vi "TC-4.59-backup.vi"() -> ()   [LabVIEW 2013]
uses:
  1. Sources/Lib/Lib.llb/CS mode.ctl
  1. Sources/Lib/Lib.llb/R.ctl
  1. Sources/Lib/Lib.llb/T.ctl
  1. Sources/Lib/Lib.llb/Calibrations.ctl
  1. Sources/Lib/Lib.llb/CS.lvclass
  1. Sources/Lib/Lib.llb/PID Settings.ctl
  1. Sources/Lib/Lib.llb/AVS_exc_n_ranges.ctl
  1. Sources/Lib/Lib.llb/AVS_excitation.ctl
  1. Sources/Lib/Lib.llb/AVS47_range.ctl
  1. Sources/Lib/Lib.llb/Ch descriptions.ctl
  1. Sources/Lib/Lib.llb/Cursor Controls.ctl
  1. Sources/Lib/Lib.llb/DataArray.ctl
  1. Sources/Lib/Lib.llb/Unit.ctl
  1. Sources/Lib/Lib.llb/Control 6.ctl
  1. Sources/Lib/Lib.llb/Control 4.ctl
  1. Sources/Lib/Lib.llb/Control 8.ctl
  1. Sources/Lib/Lib.llb/VI FPO Ref.ctl
  1. Sources/Lib/support/Class ID ENUM.ctl
  1. Sources/Lib/Lib.llb/Type Descriptor Enumeration__ogtk.ctl
  1. Sources/Lib/Lib.llb/Refnum Subtype Enum__ogtk.ctl
  1. Sources/Lib/Lib.llb/Waveform Subtype Enum__ogtk.ctl
  1. Sources/Lib/Lib.llb/LV Data cluster.ctl
  1. Sources/Lib/Lib.llb/Action.ctl
  Leiden to DSC/TC to DSC/Typedefs/TC-cluster.ctl
  1. Sources/Lib/Lib.llb/TCS.lvclass
  1. Sources/Lib/Lib.llb/QCS.lvclass
  1. Sources/Lib/Lib.llb/CS Emulation.lvclass
  1. Sources/Lib/Lib.llb/PCS.lvclass
  1. Sources/Lib/Lib.llb/Byte Params.ctl
  1. Sources/Lib/Lib.llb/MView.lvlib
panel:
  out "R Array":dbl[](array[numeric])
  out "_SetControl":T1
  out "ControlNames":string[](array[string])
  out "VIRef":T2 {"Array DataType" format="%.0x"; "WaveForm Type" format="%.0x"; "RefNum Type" format="%.0x"; "DataType" format="%.0x"}
  out "VI called?":bool=TRUE
  out "Error code":u8
  out "_zBridgeSetNr":u8 caption="zBridge set nr."
  out "_zBridgeDll":path=path "C:/Users/Sasha/Dropbox/Labview/LC Software/ImpSoft-V5.2.2-multithreaded/ImpBridgeLabview/ImpBridgeDll.dll"
  in  "_String":string="^ Click the Run button to start the program "
  in  "Top Toolbar":enum32{"Page 1", "Page 2"}(tab)
  in  "Load config":bool
  in  "Start":bool
  in  "Load Data":bool
  in  "Pause":bool
  in  "Stop":bool
  in  "Copy to Clipboard":bool
  in  "Save config":bool
  in  "Clear all plots":bool
  in  "ColorBox":enum32{"Page 1", "Page 2"}(tab)
  in  "Colors":picture
  out "Color":u32(colorbox)
  in  "Graph-open popup":bool
  out "_CalibFilesPath":path=path "C:/avs-47/aaaa"
  out "_LogFilesPath":path
  out "_AVS_VISA":refnum<visa-resource-name>="COM3"
  in  "Minimize UI 2":bool
  out "VI Version":string="TC" caption="V"
  in  "Minimize UI 1":bool
  in  "Main Panel":enum32{"AVS"}(tab)
  in  "Graph Controls Bar":enum32{"Page 1"}(tab)
  in  "Mode Buttons":T7
  in  "Erase all":bool
  in  "Plot-Save All":bool
  in  "Plot-save-screen":bool
  in  "Channels Panel":T8(tab)=enum."All"
  out "T0":dbl=nan caption="T" format="%#.2p"
  out "R0":dbl caption="R" format="%.3p"
  out "R-Plot 0":cluster{dbl[], dbl[]}(graph) caption="R-Plot"
  out "T1":dbl=nan caption="T" format="%#.2p"
  out "R1":dbl caption="R" format="%.3p"
  out "R-Plot 1":cluster{dbl[], dbl[]}(graph) caption="R-Plot"
  out "T2":dbl=nan caption="T" format="%#.2p"
  out "R2":dbl caption="R" format="%.3p"
  out "R-Plot 2":cluster{dbl[], dbl[]}(graph) caption="R-Plot"
  out "T3":dbl=nan caption="T" format="%#.2p"
  out "R3":dbl caption="R" format="%.3p"
  out "R-Plot 3":cluster{dbl[], dbl[]}(graph) caption="R-Plot"
  out "T4":dbl=nan caption="T" format="%#.2p"
  out "R4":dbl caption="R" format="%.3p"
  out "R-Plot 4":cluster{dbl[], dbl[]}(graph) caption="R-Plot"
  out "T5":dbl=nan caption="T" format="%#.2p"
  out "R5":dbl caption="R" format="%.3p"
  out "R-Plot 5":cluster{dbl[], dbl[]}(graph) caption="R-Plot"
  out "T6":dbl=nan caption="T" format="%#.2p"
  out "R6":dbl caption="R" format="%.3p"
  out "R-Plot 6":cluster{dbl[], dbl[]}(graph) caption="R-Plot"
  out "T7":dbl=nan caption="T" format="%#.2p"
  out "R7":dbl caption="R" format="%.3p"
  out "R-Plot 7":cluster{dbl[], dbl[]}(graph) caption="R-Plot"
  out "T8":dbl=nan caption="T" format="%#.2p"
  out "R8":dbl caption="R" format="%.3p"
  out "R-Plot 8":cluster{dbl[], dbl[]}(graph) caption="R-Plot"
  out "T9":dbl=nan caption="T" format="%#.2p"
  out "R9":dbl caption="R" format="%.3p"
  out "R-Plot 9":cluster{dbl[], dbl[]}(graph) caption="R-Plot"
  out "T Cluster":T9 {"T9" format="%.2p"; "T8" format="%.2p"; "T7" format="%.2p"; "T6" format="%.2p"; "T5" format="%.2p"; "T4" format="%.2p"; "T3" format="%.2p"; "T2" format="%.2p"; "T1" format="%.2p"; "T0" format="%.2p"}
  in  "Sensor Names":T10={"AVS Name 0"="C_still", "AVS Name 1"="3K", "AVS Name 2"="Still", "AVS Name 3"="50mK", "AVS Name 4"="MC", "AVS Name 5"="MC", "AVS Name 6"="MC", "AVS Name 7"="", "AVS Name 8"="", "AVS Name 9"=""}
  in  "Edit Calibrations":T11
  in  "Sensor Calibrations":T12 {"Sensor 10" items=["No Calibration", "PT100", "PT1000", "RuO2 10k", "RuO2 1k5", "RuO2 2k", "Emulation R", "PT 1000", "RuO2-10K-NEW", "testCMN", "No Calibration"]; "Sensor 9" items=["No Calibration", "PT100", "PT1000", "RuO2 10k", "RuO2 1k5", "RuO2 2k", "Emulation R", "PT 1000", "RuO2-10K-NEW", "testCMN", "No Calibration"]; "Sensor 8" items=["No Calibration", "PT100", "PT1000", "RuO2 10k", "RuO2 1k5", "RuO2 2k", "Emulation R", "PT 1000", "RuO2-10K-NEW", "testCMN", "No Calibration"]; "Sensor 7" items=["No Calibration", "PT100", "PT1000", "RuO2 10k", "RuO2 1k5", "RuO2 2k", "Emulation R", "PT 1000", "RuO2-10K-NEW", "testCMN", "No Calibration"]; "Sensor 6" items=["No Calibration", "PT100", "PT1000", "RuO2 10k", "RuO2 1k5", "RuO2 2k", "Emulation R", "PT 1000", "RuO2-10K-NEW", "testCMN", "No Calibration"]; "Sensor 5" items=["No Calibration", "PT100", "PT1000", "RuO2 10k", "RuO2 1k5", "RuO2 2k", "Emulation R", "PT 1000", "RuO2-10K-NEW", "testCMN", "No Calibration"]; "Sensor 4" items=["No Calibration", "PT100", "PT1000", "RuO2 10k", "RuO2 1k5", "RuO2 2k", "Emulation R", "PT 1000", "RuO2-10K-NEW", "testCMN", "No Calibration"]; "Sensor 3" items=["No Calibration", "PT100", "PT1000", "RuO2 10k", "RuO2 1k5", "RuO2 2k", "Emulation R", "PT 1000", "RuO2-10K-NEW", "testCMN", "No Calibration"]; "Sensor 2" items=["No Calibration", "PT100", "PT1000", "RuO2 10k", "RuO2 1k5", "RuO2 2k", "Emulation R", "PT 1000", "RuO2-10K-NEW", "testCMN", "No Calibration"]; "Sensor 1" items=["No Calibration", "PT100", "PT1000", "RuO2 10k", "RuO2 1k5", "RuO2 2k", "Emulation R", "PT 1000", "RuO2-10K-NEW", "testCMN", "No Calibration"]}
  out "Units":T13
  out "R Cluster":T14={"R0"=0.0, "R1"=0.0, "R2"=-0.0, "R3"=0.0, "R4"=0.0, "R5"=0.0, "R6"=0.0, "R7"=0.0, "R8"=0.0, "R9"=0.0} {"R9" format="%.3p"; "R8" format="%.3p"; "R7" format="%.3p"; "R6" format="%.3p"; "R5" format="%.3p"; "R4" format="%.3p"; "R3" format="%.3p"; "R2" format="%.3p"; "R1" format="%.3p"; "R0" format="%.3p"}
  in  "AVS Scan Parameters":enum32{"Page 1", "Page 2"}(tab)
  in  "AVS Exc&Ranges":T15={"Excitation 0"=4, "Excitation 1"=4, "Excitation 2"=3, "Excitation 3"=3, "Excitation 4"=3, "Excitation 5"=3, "Excitation 6"=3, "Excitation 7"=3, "Range 0"=5, "Range 1"=5, "Range 2"=5, "Range 3"=5, "Range 4"=5, "Range 5"=5, "Range 6"=5, "Range 7"=5} {"Range 7" items=["n.a."=-1, "open"=0, "2 Ohm"=1, "20 Ohm"=2, "200 Ohm"=3, "2k Ohm"=4, "20k Ohm"=5, "200k Ohm"=6, "2M Ohm"=7]; "Range 6" items=["n.a."=-1, "open"=0, "2 Ohm"=1, "20 Ohm"=2, "200 Ohm"=3, "2k Ohm"=4, "20k Ohm"=5, "200k Ohm"=6, "2M Ohm"=7]; "Range 5" items=["n.a."=-1, "open"=0, "2 Ohm"=1, "20 Ohm"=2, "200 Ohm"=3, "2k Ohm"=4, "20k Ohm"=5, "200k Ohm"=6, "2M Ohm"=7]; "Range 4" items=["n.a."=-1, "open"=0, "2 Ohm"=1, "20 Ohm"=2, "200 Ohm"=3, "2k Ohm"=4, "20k Ohm"=5, "200k Ohm"=6, "2M Ohm"=7]; "Range 3" items=["n.a."=-1, "open"=0, "2 Ohm"=1, "20 Ohm"=2, "200 Ohm"=3, "2k Ohm"=4, "20k Ohm"=5, "200k Ohm"=6, "2M Ohm"=7]; "Range 2" items=["n.a."=-1, "open"=0, "2 Ohm"=1, "20 Ohm"=2, "200 Ohm"=3, "2k Ohm"=4, "20k Ohm"=5, "200k Ohm"=6, "2M Ohm"=7]; "Range 1" items=["n.a."=-1, "open"=0, "2 Ohm"=1, "20 Ohm"=2, "200 Ohm"=3, "2k Ohm"=4, "20k Ohm"=5, "200k Ohm"=6, "2M Ohm"=7]; "Range 0" items=["n.a."=-1, "open"=0, "2 Ohm"=1, "20 Ohm"=2, "200 Ohm"=3, "2k Ohm"=4, "20k Ohm"=5, "200k Ohm"=6, "2M Ohm"=7]; "Excitation 7" items=["none", "3 µV", "10 µV", "30 µV", "100 µV", "300 µV", "1 mV", "3 mV"]; "Excitation 6" items=["none", "3 µV", "10 µV", "30 µV", "100 µV", "300 µV", "1 mV", "3 mV"]; "Excitation 5" items=["none", "3 µV", "10 µV", "30 µV", "100 µV", "300 µV", "1 mV", "3 mV"]; "Excitation 4" items=["none", "3 µV", "10 µV", "30 µV", "100 µV", "300 µV", "1 mV", "3 mV"]; "Excitation 3" items=["none", "3 µV", "10 µV", "30 µV", "100 µV", "300 µV", "1 mV", "3 mV"]; "Excitation 2" items=["none", "3 µV", "10 µV", "30 µV", "100 µV", "300 µV", "1 mV", "3 mV"]; "Excitation 1" items=["none", "3 µV", "10 µV", "30 µV", "100 µV", "300 µV", "1 mV", "3 mV"]; "Excitation 0" items=["none", "3 µV", "10 µV", "30 µV", "100 µV", "300 µV", "1 mV", "3 mV"]}
  out "zBridge.Scan Phase":T18
  out "zBridge params":T19
  out "uPlots":T20
  out "zBridge.Active Channels":T21={"active Channel 0"=TRUE, "active Channel 1"=TRUE, "active Channel 2"=TRUE, "active Channel 3"=FALSE, "active Channel 4"=FALSE, "active Channel 5"=FALSE, "active Channel 6"=FALSE, "active Channel 7"=FALSE, "active Channel 8"=FALSE, "active Channel 9"=FALSE}
  out "Waveform Chart":T22(graph)
  in  "_CS_Address":u32
  in  "Edit calibration":bool
  in  "Convert R-T":bool
  out "T7":dbl caption="T=" format="%#.2p"
  in  "QuickR":dbl caption="R=" format="%_6g"
  in  "_QuickConvertCal":u16(ring) items=["No Calibration", "PT100", "PT1000", "RuO2 10k", "RuO2 1k5", "RuO2 2k", "Emulation R", "PT 1000", "RuO2-10K-NEW", "testCMN", "No Calibration"]
  out "_CSMode1List[i]":T23[](array[typedef]) caption="I_list[i]" min=-1.0
  out "CS.Automode Current":T23[](array[typedef]) min=-1.0
  in  "Lower Panel":enum32{"Page 1", "Page 2"}(tab)
  in  "Data History/RT Settings":enum32{"History", "Settings"}(tab)=enum."Settings"
  out "AVS names small":T10={"AVS Name 0"="3K", "AVS Name 1"="Still", "AVS Name 2"="50 mK", "AVS Name 3"="MC", "AVS Name 4"="MC", "AVS Name 5"="", "AVS Name 6"="", "AVS Name 7"="", "AVS Name 8"="", "AVS Name 9"=""}
  out "zBridge.Active channel":T24
  out "Small T Cluster":T25 caption="T" {"T0" format="%#.2p"; "T1" format="%#.2p"; "T2" format="%#.2p"; "T3" format="%#.2p"; "T4" format="%#.2p"; "T5" format="%#.2p"; "T6" format="%#.2p"; "T7" format="%#.2p"; "T8" format="%#.2p"; "T9" format="%#.2p"}
  out "Small R Cluster":T26 caption="R" {"R0" format="%#_5p"; "R1" format="%#_5p"; "R2" format="%#_5p"; "R3" format="%#_5p"; "R4" format="%#_5p"; "R5" format="%#_5p"; "R6" format="%#_5p"; "R7" format="%#_5p"; "R8" format="%#_5p"; "R9" format="%#_5p"}
  out "Time":dbl format="%<%X\n%x>T"
  in  "Runtime Settings":T27={"Read AVS channels from"=0, "Last Channel"=7, "Delay Between Scans"=0, "Stabilisation Delay"=5.0, "Averages"=2, "Data Memory"=25000, "Filter Graphs"=FALSE, "Y_min"=0.0, "Y_max"=2000000.0, "Plot type"=enum."T vs Time", "Allow neg R"=TRUE, "Miniplot Time"=30.0} {"Miniplot Time" min=0.0; "Delay Between Scans" format="%.0f s"; "Averages" min=1 max=1000; "Stabilisation Delay" min=0.5; "Last Channel" min=0 max=7 step=1; "Read AVS channels from" min=0 max=7 step=1; "Y_max" format="%#_6f"; "Y_min" min=0.0 format="%#_6f"; "Data Memory" min=3 max=50000}
  out "CS.Current Value":dbl[](array[numeric])
  in  "Data Array":T28=[{"R"=[], "T"=[], "Time"=[]}, {"R"=[0.0, 2.0], "T"=[], "Time"=[]}]
  out "T Array":dbl[](array[numeric])
  in  "_ScanData":dbl[](array[numeric])
  out "_I3SetPnt":dbl
  out "_CurrentsChanged":bool
  in  "_AVSRanges":T29={"Excitationl 0"=5, "Excitation 1"=5, "Excitation 2"=5, "Excitation 3"=5, "Excitation 4"=5, "Excitation 5"=5, "Excitation 6"=5, "Excitation 7"=5} caption="Ranges" {"Excitation 7" items=["n.a."=-1, "open"=0, "2 Ohm"=1, "20 Ohm"=2, "200 Ohm"=3, "2k Ohm"=4, "20k Ohm"=5, "200k Ohm"=6, "2M Ohm"=7]; "Excitation 6" items=["n.a."=-1, "open"=0, "2 Ohm"=1, "20 Ohm"=2, "200 Ohm"=3, "2k Ohm"=4, "20k Ohm"=5, "200k Ohm"=6, "2M Ohm"=7]; "Excitation 5" items=["n.a."=-1, "open"=0, "2 Ohm"=1, "20 Ohm"=2, "200 Ohm"=3, "2k Ohm"=4, "20k Ohm"=5, "200k Ohm"=6, "2M Ohm"=7]; "Excitation 4" items=["n.a."=-1, "open"=0, "2 Ohm"=1, "20 Ohm"=2, "200 Ohm"=3, "2k Ohm"=4, "20k Ohm"=5, "200k Ohm"=6, "2M Ohm"=7]; "Excitation 3" items=["n.a."=-1, "open"=0, "2 Ohm"=1, "20 Ohm"=2, "200 Ohm"=3, "2k Ohm"=4, "20k Ohm"=5, "200k Ohm"=6, "2M Ohm"=7]; "Excitation 2" items=["n.a."=-1, "open"=0, "2 Ohm"=1, "20 Ohm"=2, "200 Ohm"=3, "2k Ohm"=4, "20k Ohm"=5, "200k Ohm"=6, "2M Ohm"=7]; "Excitation 1" items=["n.a."=-1, "open"=0, "2 Ohm"=1, "20 Ohm"=2, "200 Ohm"=3, "2k Ohm"=4, "20k Ohm"=5, "200k Ohm"=6, "2M Ohm"=7]; "Excitationl 0" items=["n.a."=-1, "open"=0, "2 Ohm"=1, "20 Ohm"=2, "200 Ohm"=3, "2k Ohm"=4, "20k Ohm"=5, "200k Ohm"=6, "2M Ohm"=7]}
  out "_CSClassRef":refnum<class "CS.lvclass">
  in  "CS Indicators Panel":enum32{"Page 1", "Page 2"}(tab)
  out "CS.Automode 0":bool
  out "CS.Automode 1":bool
  out "QCS. I0 Mapping":T30(ring) caption="Output to"
  in  "uA 0":u32
  in  "CS Cannel Names":T31={"CS Name 0"="N.C.", "CS Name 1"="3K", "CS Name 2"="Still", "CS Name 3"="MC"}
  out "I0":T32={"uA"="000", "ON"=FALSE, "Gated"=FALSE, "current flows"=FALSE, "Error"=FALSE} caption="Ch0 -"
  in  "uA 3":u32
  in  "uA 2":u32
  in  "uA 1":u32
  out "CS.Automode 3":bool
  out "CS.Automode 2":bool
  out "I3":T32={"uA"="000", "ON"=FALSE, "Gated"=FALSE, "current flows"=FALSE, "Error"=FALSE} caption="Chn 3"
  out "I2":T32={"uA"="000", "ON"=FALSE, "Gated"=FALSE, "current flows"=FALSE, "Error"=FALSE} caption="Chn 2"
  out "I1":T32={"uA"="000", "ON"=FALSE, "Gated"=FALSE, "current flows"=FALSE, "Error"=FALSE} caption="Chn 1"
  out "_ExtVIReference":refnum<vi>
  out "Small I":cluster{"I1":dbl, "I2":dbl, "I3":dbl, "I4":dbl} caption="I" {"I1" format="%#.2f"; "I2" format="%#.2p"; "I3" format="%#.2p"; "I4" format="%#.2p"}
  out "CS.Actual Current":dbl[](array[numeric])
  in  "Save Data 2":bool
  in  "Show PID graph?":bool
  in  "Set Color":bool
  out "_ZBridgeUnit":string caption="Unit"
  out "_zBridgeParText":string caption="zBridge params/Error"
  out "_CurCalibrations":T33
  out "_LMBDown":bool
  in  "Side Panel":T34(tab)
  in  "Reload Calibrations":bool
  in  "zBridge settings":bool
  out "CS.ID":string
  out "CS status":errorcluster
  out "General Error":errorcluster caption="General status"
  in  "Bridge settings":T35={"Bridge Type"=enum."AVS47A (GPIB interface)", "AVS RS232 Port"="COM5", "AVS GPIB Address"="GPIB0::20::INSTR", "Calibrations Folder"=path "C:/LC Data/Calibrations"}
  in  "CS Settings":T36={"TCS RS232 Port"="COM1", "TCS_Imax"=5, "CS type"=enum."TCS", "CS.QCS Device Nr"=0}
  in  "Data Logging Settings":T37={"Log Files Folder"=path "C:/LC Data/Data", "Log Files Name"="LogAVS", "Automode Files Name"="calibration", "Filenames Suffix"="_%Y-%m-%d-%H-%M-%S", "Delimeter"="\t", "New File Interval"=7, "New File Interval Units"=enum."Days", "Date Format"="%Y-%m-%d %H:%M:%S", "External VI Path"=path "", "Query Description"=FALSE, "Run Description"="\n"}
  out "Bridge status":errorcluster
  in  "CS.QCS I0 Output":T38(ring) caption="Set Channel 0 output to"
  in  "CS.Mode":T39 caption="CS mode"
  out "_TimeOld":dbl format="%#_16g"
  in  "CS Modes Panel":T40(tab)=enum."Automatic 1"
  in  "CS.I3":T41={"Toggle ON/OFF"=FALSE, "Toggle Gated"=FALSE, "I"=0, "Range"=enum."x1 uA"} caption="Chn 3" {"I" max=100000 step=1}
  in  "CS.I2":T41={"Toggle ON/OFF"=FALSE, "Toggle Gated"=FALSE, "I"=0, "Range"=enum."x1 uA"} caption="Chn 2" {"I" max=100000 step=1}
  in  "CS.I1":T41={"Toggle ON/OFF"=FALSE, "Toggle Gated"=FALSE, "I"=0, "Range"=enum."x1 uA"} caption="Chn 1" {"I" max=100000 step=1}
  in  "CS.I0":T41={"Toggle ON/OFF"=FALSE, "Toggle Gated"=FALSE, "I"=0, "Range"=enum."x1 uA"} caption="Chn 0" {"I" max=100000 step=1}
  in  "CS.Mode1.PID Settings":T42={"FB on 2"=enum."3", "Proportional Gain"=3.0, "Integral Gain"=3.0, "Derivative Gain"=1.0, "Deadband"=0.1, "Feed Fwd Gain [uA/mK]"=0.0, "Integral Gain Bandwidth"=10.0, "Integral Gain Background"=1.0, "Current limit, [uA]"=1.0} {"Integral Gain Background" format="%#.6g"; "Integral Gain Bandwidth" format="%#.6g"; "Feed Fwd Gain [uA/mK]" format="%#.5g"; "Deadband" format="%#.5g"; "Derivative Gain" format="%#.6g"; "Integral Gain" format="%#.6g"; "Proportional Gain" format="%#.6g"; "Current limit, [uA]" format="%#.5g"}
  in  "CS.Mode1.Start":bool
  in  "CS.Mode1.List":T23[][](array[typedef]) min=-1.0
  out "CS.Mode1.PID Column":T43[](array[typedef])
  out "CS.Mode1.Row":T44[](array[typedef])=[TRUE, FALSE, FALSE, FALSE, FALSE, FALSE, FALSE, FALSE, FALSE, FALSE]
  out "CS.Mode1.PID Stabilized?":bool caption="SP reached?"
  out "CS.Mode1.PID Error":dbl=10.0 caption="Error" format="%#_6f"
  out "CS.Mode1.Slope":dbl caption="Slope" format="%#_3g %"
  out "CS.Mode1.Timer":dbl caption="Timer" format="%<%H:%M:%S>t"
  out "CS.Mode1.List:Count":i32=10 caption="/"
  out "CS.Mode1.List:Index":i32=10 caption="Point #"
  in  "CS.Mode1.Next":bool
  in  "CS.Mode1.Reset PID":bool
  in  "CS.Mode1.Auto Advance":bool=TRUE caption="Enable automatic sweeping/list iteration"
  in  "CS.Mode1.Settings":T45={"Bridge Channel"=0, "N averages"=10, "Delay Time"=10.0, "T stability"=0.3, "FB on"=enum."Temperature"} {"Delay Time" min=0.0 format="%#_g min"; "Bridge Channel" min=-1 max=9 step=1}
  in  "CS.Mode1.Call VI?":bool caption="Call Ext. VI"
  out "CS.Mode1.VI State":T46(ring) caption="- state"
  in  "CS.Mode1.Trigger all TC":bool caption="Trigger other running TC instances"
  in  "CS.Mode1.List:Prev":bool
  in  "CS.Mode1.List:Next":bool
  in  "CS.Mode1.List:To First":bool
  in  "CS.Mode1.List:Save":bool
  in  "CS.Mode1.List:Load":bool
  in  "CS.Mode1.Write To Log":bool
  in  "CS.Mode1.PID":cluster{"Enabled":bool}
  in  "CS.Mode1.List:Clear":bool
  in  "CS.Mode2.Settings":T47={"FB on"=enum."Temperature", "Bridge Channel"=0, "Hysteresis"=10} {"Hysteresis" max=100 format="%.0f %%"; "Bridge Channel" min=-1 max=9 step=1}
  in  "CS.Mode2.Start":bool
  in  "CS.Mode2.Add Row":bool
  in  "CS.Mode2.New Row":dbl[](array[numeric])=[0.0, 0.0, 0.0, 0.0, 0.0, 0.0] caption="New range" min=-1.0
  in  "CS.Mode2.List":dbl[][](array[numeric])=[[0.0, 0.0, 0.0, 0.0, 0.0, inf]] min=-1.0
  out "CS.Mode2.Row":T44[](array[typedef])=[TRUE, FALSE, FALSE, FALSE, FALSE, FALSE, FALSE, FALSE, FALSE, FALSE]
  in  "T Sweep":T48={"Start value"=200.0, "End value"=250.0, "Step"=10.0, "Current"=0.0, "I_next"=FALSE, "I_prev"=FALSE, "Interrrupt Sweep"=FALSE, "Start"=FALSE, "Boolean"=TRUE} {"Step" min=0.0; "End value" min=0.0; "Start value" min=0.0}
  # "Quick convert R->T:"
  # "Ohm"
  # "mK"
  # "Ch#"
  # "Miniplot"
  # "Channel parameters"
  # "Impedance"
  # "Unit"
  # "Type of sensor"
  # "T [mK]"
  # "Description"
  # "0"
  # "1"
  # "2"
  # "3"
  # "4"
  # "5"
  # "6"
  # "7"
  # "8"
  # "9"
  # "0"
  # "1"
  # "2"
  # "3"
  # "4"
  # "5"
  # "7"
  # "8"
  # "9"
  # "6"
  # "auto"
  # "auto"
  # "auto"
  # "auto"
  # "gated"
  # "gated"
  # "gated"
  # "gated"
  # "Status"
  # "Current source mode"
  # "Current source manual control"
  # "Current source automatic mode #1"
  # "Currents List"
  # "Settings"
  # "I0"
  # "I1"
  # "I2"
  # "I3"
  # "Status"
  # "On temperature stabilized"
  # "Current source automatic mode #2"
  # "Currents List"
  # "Settings"
  # "T0"
  # "T1"
  # "I0"
  # "I1"
  # "I2"
  # "I3"
  # "T0"
  # "T1"
  # "I0"
  # "I1"
  # "I2"
  # "I3"
  # "Ch3"
types:
  T1 = typedef "MView.lvlib/LV Data cluster.ctl" = cluster{"Name":string, "Scalar":string, "Array":string[][]}
  T2 = typedef "MView.lvlib/VI FPO Ref.ctl" = cluster{"Control Ref ID":refnum<vi>[], "Full Name":string[], "ClassID":T3[], "Short Name":string[], "DataType":T4[], "RefNum Type":T5[], "WaveForm Type":T6[], "Parent":i32[], "Array DataType":T4[], "Owning VI":refnum<vi>[], "Active?":bool[]}
  T3 = typedef "Class ID ENUM.ctl" = enum16{"<Null>", "1", "2", "Generic", "Decoration", "Text", "Control", "ColorBox", "Boolean", "RefNum", "Variant", "Path", "ListBox", "Table", "Array", "Picture", "ActiveXContainer", "Numeric", "Digital", "NamedNumeric", "ColorRamp", "Slide", "GraphOrChart", "WaveformChart", "WaveformGraph", "IntensityChart", "IntensityGraph", "String", "IOName", "ComboBox", "Cluster", "Panel", "Knob", "NumWithScale", "Ring", "Enum", "GObject", "Plot", "Cursor", "NumericText", "Scale", "ColorScale", "GraphScale", "ColorGraphScale", "TypedRefNum", "OldKnobScale", "MCListbox", "MeasureData", "BVTag", "DAQName", "VISAName", "IVIName", "SlideScale", "TabControl", "Page", "TabArrayTabControl", "ConPane", "57", "58", "59", "60", "61", "62", "63", "64", "SubPanel", "TreeControl", "67", "68", "69", "70", "71", "72", "73", "74", "75", "SplitterBar"}
  T4 = typedef "Type Descriptor Enumeration__ogtk.ctl" = enum8{"<Null>", "I8", "I16", "I32", "I64", "U8", "U16", "U32", "U64", "SGL", "DBL", "EXT", "CSG", "CDB", "CXT", "0x0F", "0x10", "0x11", "0x12", "0x13", "0x14", "Enum U8", "Enum U16", "Enum U32", "Enum U64", "SGL PQ", "DBL PQ", "EXT PQ", "CSG PQ", "CDB PQ", "CXT PQ", "0x1F", "0x20", "Boolean", "0x22", "0x23", "0x24", "0x25", "0x26", "0x27", "0x28", "0x29", "0x2A", "0x2B", "0x2C", "0x2D", "0x2E", "0x2F", "String", "0x31", "Path", "Pict", "0x34", "0x35", "0x36", "DAQ", "0x38", "0x39", "0x3A", "0x3B", "0x3C", "0x3D", "0x3E", "0x3F", "Array", "0x41", "0x42", "0x43", "0x44", "0x45", "0x46", "0x47", "0x48", "0x49", "0x4A", "0x4B", "0x4C", "0x4D", "0x4E", "0x4F", "Cluster", "0x51", "0x52", "Variant", "Waveform", "0x55", "0x56", "0x57", "0x58", "0x59", "0x5A", "0x5B", "0x5C", "0x5D", "0x5E", "0x5F", "0x60", "0x61", "0x62", "0x63", "0x64", "0x65", "0x66", "0x67", "0x68", "0x69", "0x6A", "0x6B", "0x6C", "0x6D", "0x6E", "0x6F", "Refnum"}
  T5 = typedef "Refnum Subtype Enum__ogtk.ctl" = enum8{"Generic", "Datalog File Refnum", "Byte Stream File Refnum", "Device Refnum", "Occurence Refnum", "TCP Connection Refnum", "VISA Refnum (Obsolete)", "Automation Renum", "VI Server Refnum", "Menu Refnum", "IVI Refnum (Obsolete)", "IMAQ Session", "0x0C", "Datasocket Refnum", "VISA Resource", "IVI Logical Name", "UDP Connection Refnum", "Notifier Refnum", "Queue Refnum", "IrDA Refnum", "Hardware Plugin Refnum", "Hardware Plugin Tag Refnum", "DAQmx Refnum", "Event Registration Refnum", ".NET Refnum", "User Event Refnum", "0x1A", "Event Callback", "0x1C", "0x1D", "Only Used Internal to LabVIEW", "Bluetooth", "Data Value References", "RT FIFO", "TDM Streaming"}
  T6 = typedef "Waveform Subtype Enum__ogtk.ctl" = enum8{"<Not a Waveform Type>", "0x01", "Analog 16-bit signed", "Analog Double-Precision", "0x04", "Analog Single Precision", "Timestamp", "Digital Data", "Digital Waveform", "Dynamic Data", "Analog Extended-Precision", "Analog 8-bit unsigned", "Analog 16-bit unsigned", "Analog 32-bit unsigned", "Analog 8-bit signed", "Analog 32-bit signed", "Analog Complex Single-Precision", "Analog Complex Double-Precision", "Analog Complex Extended Precision", "Analog 64-bit signed", "Analog 64-bit unsigned"}
  T7 = typedef "Cursor Controls.ctl" = enum32{"No Selection", "Cursor mode", "Erase point", "Erase range"}
  T8 = enum32{"0", "1", "2", "3", "4", "5", "6", "7", "8", "9", "All", "PID loop"}
  T9 = typedef "T.ctl" = cluster{"T0":dbl, "T1":dbl, "T2":dbl, "T3":dbl, "T4":dbl, "T5":dbl, "T6":dbl, "T7":dbl, "T8":dbl, "T9":dbl}
  T10 = typedef "Ch descriptions.ctl" = cluster{"AVS Name 0":string, "AVS Name 1":string, "AVS Name 2":string, "AVS Name 3":string, "AVS Name 4":string, "AVS Name 5":string, "AVS Name 6":string, "AVS Name 7":string, "AVS Name 8":string, "AVS Name 9":string}
  T11 = cluster{"Boolean":bool, "Boolean 2":bool, "Boolean 3":bool, "Boolean 4":bool, "Boolean 5":bool, "Boolean 6":bool, "Boolean 7":bool, "Boolean 8":bool, "Boolean 9":bool, "Boolean 10":bool}
  T12 = typedef "Calibrations.ctl" = cluster{"Sensor 1":u16, "Sensor 2":u16, "Sensor 3":u16, "Sensor 4":u16, "Sensor 5":u16, "Sensor 6":u16, "Sensor 7":u16, "Sensor 8":u16, "Sensor 9":u16, "Sensor 10":u16}
  T13 = typedef "Unit.ctl" = cluster{"Value 0":string, "Value 1":string, "Value 2":string, "Value 3":string, "Value 4":string, "Value 5":string, "Value 6":string, "Value 7":string, "Value 8":string, "Value 9":string}
  T14 = typedef "R.ctl" = cluster{"R0":dbl, "R1":dbl, "R2":dbl, "R3":dbl, "R4":dbl, "R5":dbl, "R6":dbl, "R7":dbl, "R8":dbl, "R9":dbl}
  T15 = typedef "AVS_exc_n_ranges.ctl" = cluster{"Excitation 0":T16, "Excitation 1":T16, "Excitation 2":T16, "Excitation 3":T16, "Excitation 4":T16, "Excitation 5":T16, "Excitation 6":T16, "Excitation 7":T16, "Range 0":T17, "Range 1":T17, "Range 2":T17, "Range 3":T17, "Range 4":T17, "Range 5":T17, "Range 6":T17, "Range 7":T17}
  T16 = typedef "AVS_excitation.ctl" = i16
  T17 = typedef "AVS47_range.ctl" = i16
  T18 = cluster{"Value 0":dbl, "Value 1":dbl, "Value 2":dbl, "Value 3":dbl, "Value 4":dbl, "Value 5":dbl, "Value 6":dbl, "Value 7":dbl, "Value 8":dbl, "Value 9":dbl}
  T19 = cluster{"AVS Name 0":string, "AVS Name 1":string, "AVS Name 2":string, "AVS Name 3":string, "AVS Name 4":string, "AVS Name 5":string, "AVS Name 6":string, "AVS Name 7":string, "AVS Name 8":string, "AVS Name 9":string}
  T20 = cluster{"uPlot 0":cluster{dbl[], dbl[]}, "uPlot 1":cluster{dbl[], dbl[]}, "uPlot 2":cluster{dbl[], dbl[]}, "uPlot 3":cluster{dbl[], dbl[]}, "uPlot 4":cluster{dbl[], dbl[]}, "uPlot 5":cluster{dbl[], dbl[]}, "uPlot 6":cluster{dbl[], dbl[]}, "uPlot 7":cluster{dbl[], dbl[]}, "uPlot 8":cluster{dbl[], dbl[]}, "uPlot 9":cluster{dbl[], dbl[]}}
  T21 = cluster{"active Channel 0":bool, "active Channel 1":bool, "active Channel 2":bool, "active Channel 3":bool, "active Channel 4":bool, "active Channel 5":bool, "active Channel 6":bool, "active Channel 7":bool, "active Channel 8":bool, "active Channel 9":bool}
  T22 = cluster{"Ip":dbl, "Ii":dbl, "Id":dbl, "Iff":dbl, "I_tot":dbl}
  T23 = typedef "Control 4.ctl" = dbl
  T24 = cluster{"Boolean 5":bool, "Boolean 5":bool, "Boolean 5":bool, "Boolean 5":bool, "Boolean 5":bool, "Boolean 5":bool, "Boolean 5":bool, "Boolean 5":bool, "Boolean 5":bool, "Boolean 5":bool}
  T25 = cluster{"T0":dbl, "T1":dbl, "T2":dbl, "T3":dbl, "T4":dbl, "T5":dbl, "T6":dbl, "T7":dbl, "T8":dbl, "T9":dbl}
  T26 = cluster{"R0":dbl, "R1":dbl, "R2":dbl, "R3":dbl, "R4":dbl, "R5":dbl, "R6":dbl, "R7":dbl, "R8":dbl, "R9":dbl}
  T27 = cluster{"Read AVS channels from":i8, "Last Channel":i8, "Delay Between Scans":u32, "Stabilisation Delay":dbl, "Averages":u16, "Data Memory":u16, "Filter Graphs":bool, "Y_min":dbl, "Y_max":dbl, "Plot type":enum16{"R vs Time", "T vs Time"}, "Allow neg R":bool, "Miniplot Time":dbl}
  T28 = typedef "DataArray.ctl" = cluster{"R":dbl[], "T":dbl[], "Time":dbl[]}[]
  T29 = cluster{"Excitationl 0":i16, "Excitation 1":i16, "Excitation 2":i16, "Excitation 3":i16, "Excitation 4":i16, "Excitation 5":i16, "Excitation 6":i16, "Excitation 7":i16}
  T30 = enum16{"Chn 0", "Aux 0", "Aux 1", "Aux 2", "Aux 3"}
  T31 = cluster{"CS Name 0":string, "CS Name 1":string, "CS Name 2":string, "CS Name 3":string}
  T32 = cluster{"uA":string, "ON":bool, "Gated":bool, "current flows":bool, "Error":bool}
  T33 = cluster{"[0]":string, "[1]":string, "[2]":string, "[3]":string, "[4]":string, "[5]":string, "[6]":string, "[7]":string, "[8]":string, "[9]":string}
  T34 = enum32{"Devices Settings", "Current source control"}
  T35 = cluster{"Bridge Type":enum16{"AVS47A (GPIB interface)", "AVS47B (RS232 interface)", "AVS48SI (RS232 interface)", "AVS Emulation", "Impedance Bridge", "Disabled"}, "AVS RS232 Port":refnum<visa-resource-name>, "AVS GPIB Address":refnum<visa-resource-name>, "Calibrations Folder":path}
  T36 = cluster{"TCS RS232 Port":refnum<visa-resource-name>, "TCS_Imax":i32, "CS type":enum16{"TCS", "QCS v1", "PCS (n.a.)", "CS Emulation", "Disabled"}, "CS.QCS Device Nr":u16}
  T37 = cluster{"Log Files Folder":path, "Log Files Name":string, "Automode Files Name":string, "Filenames Suffix":string, "Delimeter":string, "New File Interval":u32, "New File Interval Units":enum16{"Minutes", "Hours", "Days"}, "Date Format":string, "External VI Path":path, "Query Description":bool, "Run Description":string}
  T38 = enum16{"Channel 0", "Aux 0", "Aux 1", "Aux 2", "Aux 3"}
  T39 = typedef "CS mode.ctl" = enum16{"Manual", "Mode 1", "Mode2"}
  T40 = enum32{"Manual", "Automatic 1", "Automatic 2", "Automatic 3"}
  T41 = cluster{"Toggle ON/OFF":bool, "Toggle Gated":bool, "I":u32, "Range":enum8{"Auto", "x1 uA", "x10 uA", "x100 uA", "x1 mA"}}
  T42 = typedef "PID Settings.ctl" = cluster{"FB on 2":enum16{"0", "1", "2", "3"}, "Proportional Gain":dbl, "Integral Gain":dbl, "Derivative Gain":dbl, "Deadband":dbl, "Feed Fwd Gain [uA/mK]":dbl, "Integral Gain Bandwidth":dbl, "Integral Gain Background":dbl, "Current limit, [uA]":dbl}
  T43 = typedef "Control 8.ctl" = bool
  T44 = typedef "Control 6.ctl" = bool
  T45 = cluster{"Bridge Channel":i32, "N averages":i32, "Delay Time":dbl, "T stability":dbl, "FB on":enum16{"Resistance", "Temperature"}}
  T46 = enum32{"Bad", "Idle", "Run top level", "Running"}
  T47 = cluster{"FB on":enum16{"Resistance", "Temperature"}, "Bridge Channel":i32, "Hysteresis":u8}
  T48 = cluster{"Start value":dbl, "End value":dbl, "Step":dbl, "Current":dbl, "I_next":bool, "I_prev":bool, "Interrrupt Sweep":bool, "Start":bool, "Boolean":bool}
  T49 = cluster{"UpdateChannelInfo":refnum<user-event>, "UpdateValuesAVS":refnum<user-event>, "UpdateCalibrations":refnum<user-event>, "UpdateLogFilePath":refnum<user-event>, "TempStabilized":refnum<user-event>, "Reset PID loop":refnum<user-event>, "UpdateValuesZBridge":refnum<user-event>, "CS Automode":refnum<user-event>, "CallExtVI":refnum<user-event>, "Data Array":refnum<user-event>}
  T50 = cluster{"Config folder":path, "Config File":path, "Calibrations Folder":path, "zBridge dll":path, "Variables Library":path}
  T51 = enum32{"Page Enabled", "Page Disabled", "Page Disabled & Grayed"}
  T52 = cluster{"error":bool, "code":i32, "source":string}
  T53 = typedef "Action.ctl" = enum16{"Init", "Write", "Read"}
  T54 = enum16{"AVS47A (GPIB interface)", "AVS47B (RS232 interface)", "AVS48", "AVS Emulation", "Impedance Bridge", "Disabled"}
  T55 = typedef "TC-cluster.ctl" = cluster{"R":dbl[], "T":dbl[], "I":dbl[], "AVS type":enum16{"AVS47A (GPIB interface)", "AVS47B (RS232 interface)", "AVS48", "AVS Emulation", "Impedance Bridge", "Disabled"}, "AVS names":cluster{"AVS Name 0":string, "AVS Name 1":string, "AVS Name 2":string, "AVS Name 3":string, "AVS Name 4":string, "AVS Name 5":string, "AVS Name 6":string, "AVS Name 7":string, "AVS Name 8":string, "AVS Name 9":string}, "Calibration":refnum<vi>[]}
  T56 = enum32{"No Selection", "Cursor mode", "Erase point", "Erase range"}
  T57 = enum16{"TCS", "QCS v1", "PCS (n.a.)", "CS Emulation", "Disabled"}
  T58 = enum8{"Auto", "x1 uA", "x10 uA", "x100 uA", "x1 mA"}
  T59 = cluster{"Cluster":cluster{"Time":dbl[], "T":dbl[]}, "Cluster":cluster{"Time":dbl[], "T":dbl[]}, "Cluster":cluster{"Time":dbl[], "T":dbl[]}, "Cluster":cluster{"Time":dbl[], "T":dbl[]}, "Cluster":cluster{"Time":dbl[], "T":dbl[]}, "Cluster":cluster{"Time":dbl[], "T":dbl[]}, "Cluster":cluster{"Time":dbl[], "T":dbl[]}, "Cluster":cluster{"Time":dbl[], "T":dbl[]}, "Cluster":cluster{"Time":dbl[], "T":dbl[]}, "Cluster":cluster{"Time":dbl[], "T":dbl[]}}
  T60 = enum32{"invalid app kind", "Development System", "Run Time System", "Student Edition", "Embedded LabVIEW", "Evaluation", "Custom"}
  T61 = enum16{"AVS47A (GPIB interface)", "AVS47B (RS232 interface)", "AVS48SI (RS232 interface)", "AVS Emulation", "Impedance Bridge", "Disabled"}
  T62 = cluster{"[0]":dbl, "[1]":dbl, "[2]":dbl, "[3]":dbl, "[4]":dbl, "[5]":dbl, "[6]":dbl, "[7]":dbl, "[8]":dbl, "[9]":dbl}
  T63 = cluster{"Temperature[0]":dbl, "Temperature[1]":dbl, "Temperature[2]":dbl, "Temperature[3]":dbl, "Temperature[4]":dbl, "Temperature[5]":dbl, "Temperature[6]":dbl, "Temperature[7]":dbl, "Temperature[8]":dbl, "Temperature[9]":dbl}
  T64 = cluster{"Current Time (double)":dbl, "R":dbl[], "T":dbl[]}
  T65 = typedef "File Info Record__ogtk.ctl" = cluster{"type":string, "creator":string, "permissions":i32, "data size":i32, "res size":i32, "creation date":u32, "modification date":u32, "bFolder":bool, "bInvisible":bool, "location":cluster{"vertical":i16, "horizontal":i16}, "owner":string, "group":string}
  T66 = cluster{"Units[0]":string, "Units[1]":string, "Units[2]":string, "Units[3]":string, "Units[4]":string, "Units[5]":string, "Units[6]":string, "Units[7]":string, "Units[8]":string, "Units[9]":string}
  T67 = cluster{"zBridge params[0]":string, "zBridge params[1]":string, "zBridge params[2]":string, "zBridge params[3]":string, "zBridge params[4]":string, "zBridge params[5]":string, "zBridge params[6]":string, "zBridge params[7]":string, "zBridge params[8]":string, "zBridge params[9]":string}
  T68 = cluster{"date/time string":string, "Value":dbl[], "Value":dbl[], "Value":dbl[]}
  T69 = typedef "imagedata.ctl" = cluster{"image type":i32, "image depth":i32, "image":u8[], "mask":u8[], "colors":u32[], "Rectangle":cluster{"left":i16, "top":i16, "right":i16, "bottom":i16}}
  T70 = typedef "LVPoint32TypeDef.ctl" = cluster{"Horizontal":i32, "Vertical":i32}
  T71 = cluster{"Shift":bool, "Ctrl":bool, "Alt":bool, "Cmd":bool, "Opt":bool}
  T72 = cluster{"Output Array":dbl[], "array w/ subset deleted":dbl[], "array w/ subset deleted":dbl[]}
  T73 = typedef "LVRectTypeDef.ctl" = cluster{"Left":i16, "Top":i16, "Right":i16, "Bottom":i16}
  T74 = typedef "Exc_n_Ranges.ctl" = cluster{"Excitationl 0":i16, "Excitation 1":i16, "Excitation 2":i16, "Excitation 3":i16, "Excitation 4":i16, "Excitation 5":i16, "Excitation 6":i16, "Excitation 7":i16, "Range 0":i16, "Range 1":i16, "Range 2":i16, "Range 3":i16, "Range 4":i16, "Range 5":i16, "Range 6":i16, "Range 7":i16}
  T75 = enum32{"HKEY_CLASSES_ROOT", "HKEY_CURRENT_USER", "HKEY_LOCAL_MACHINE", "HKEY_USERS", "HKEY_PERFORMANCE_DATA", "HKEY_CURRENT_CONFIG", "HKEY_DYN_DATA"}
  T76 = typedef "Byte Params.ctl" = enum8{"Active", "Channel Type", "Channel No", "Reference No", "RLC select", "Save Data", "L Inverted", "Menu Active"}
  T77 = typedef "LVPositionTypeDef.ctl" = cluster{"Left":i32, "Top":i32}
  T78 = cluster{"Range 0":i16, "Range 1":i16, "Range 2":i16, "Range 3":i16, "Range 4":i16, "Range 7":i16, "Range 5":i16, "Range 6":i16}
  T79 = cluster{"Range 0":i16, "Range 1":i16, "Range 2":i16, "Range 3":i16, "Range 4":i16, "Range 5":i16, "Range 6":i16, "Range 7":i16}
  T80 = cluster{"RANGE 0":u16, "RANGE 1":u16, "RANGE 2":u16, "RANGE 3":u16, "RANGE 4":u16, "RANGE 5":u16, "RANGE 6":u16, "RANGE 7":u16}
  T81 = typedef "LCR Channel parameters.ctl" = cluster{"Set_number":u8, "Set_char":u16, "Ch_number":u8, "Ch_type":u8, "Freq":dbl, "T_int":dbl, "I_exc":dbl, "V_exc":dbl, "SNR":dbl, "Vnoise":dbl, "P_diss":dbl}
  T82 = typedef "CS Data.ctl" = cluster{"Range":u8, "Current":dbl, "Current (string)":string, "On?":bool, "G?":bool, "I?":bool, "Err?":bool}
  T83 = typedef "TCS indicator.ctl" = cluster{"uA":string, " ON":bool, "Gated":bool, "current flows":bool, "Error":bool}
  T84 = cluster{"Toggle ON/OFF":bool, "Toggle Gated":bool}
  T85 = cluster{"Current":u32, "Range":enum16{"Auto", "x1 uA", "x10 uA", "x100 uA", "x1 mA"}}
  T86 = typedef "TCS manual control.ctl" = cluster{"Toggle ON/OFF":bool, "Toggle Gated":bool, "Current":u32, "Range":enum8{"Auto", "x1 uA", "x10 uA", "x100 uA", "x1 mA"}}
  T87 = cluster{"Status[0]":i32, "Status[1]":i32, "Status[2]":i32, "Status[3]":i32, "Status[4]":i32, "Status[5]":i32, "Status[6]":i32, "Status[7]":i32, "Status[8]":i32, "Status[9]":i32}
  T88 = cluster{"Active":bool, "Active":bool, "Active":bool, "Active":bool, "Active":bool, "Active":bool, "Active":bool, "Active":bool, "Active":bool, "Active":bool}
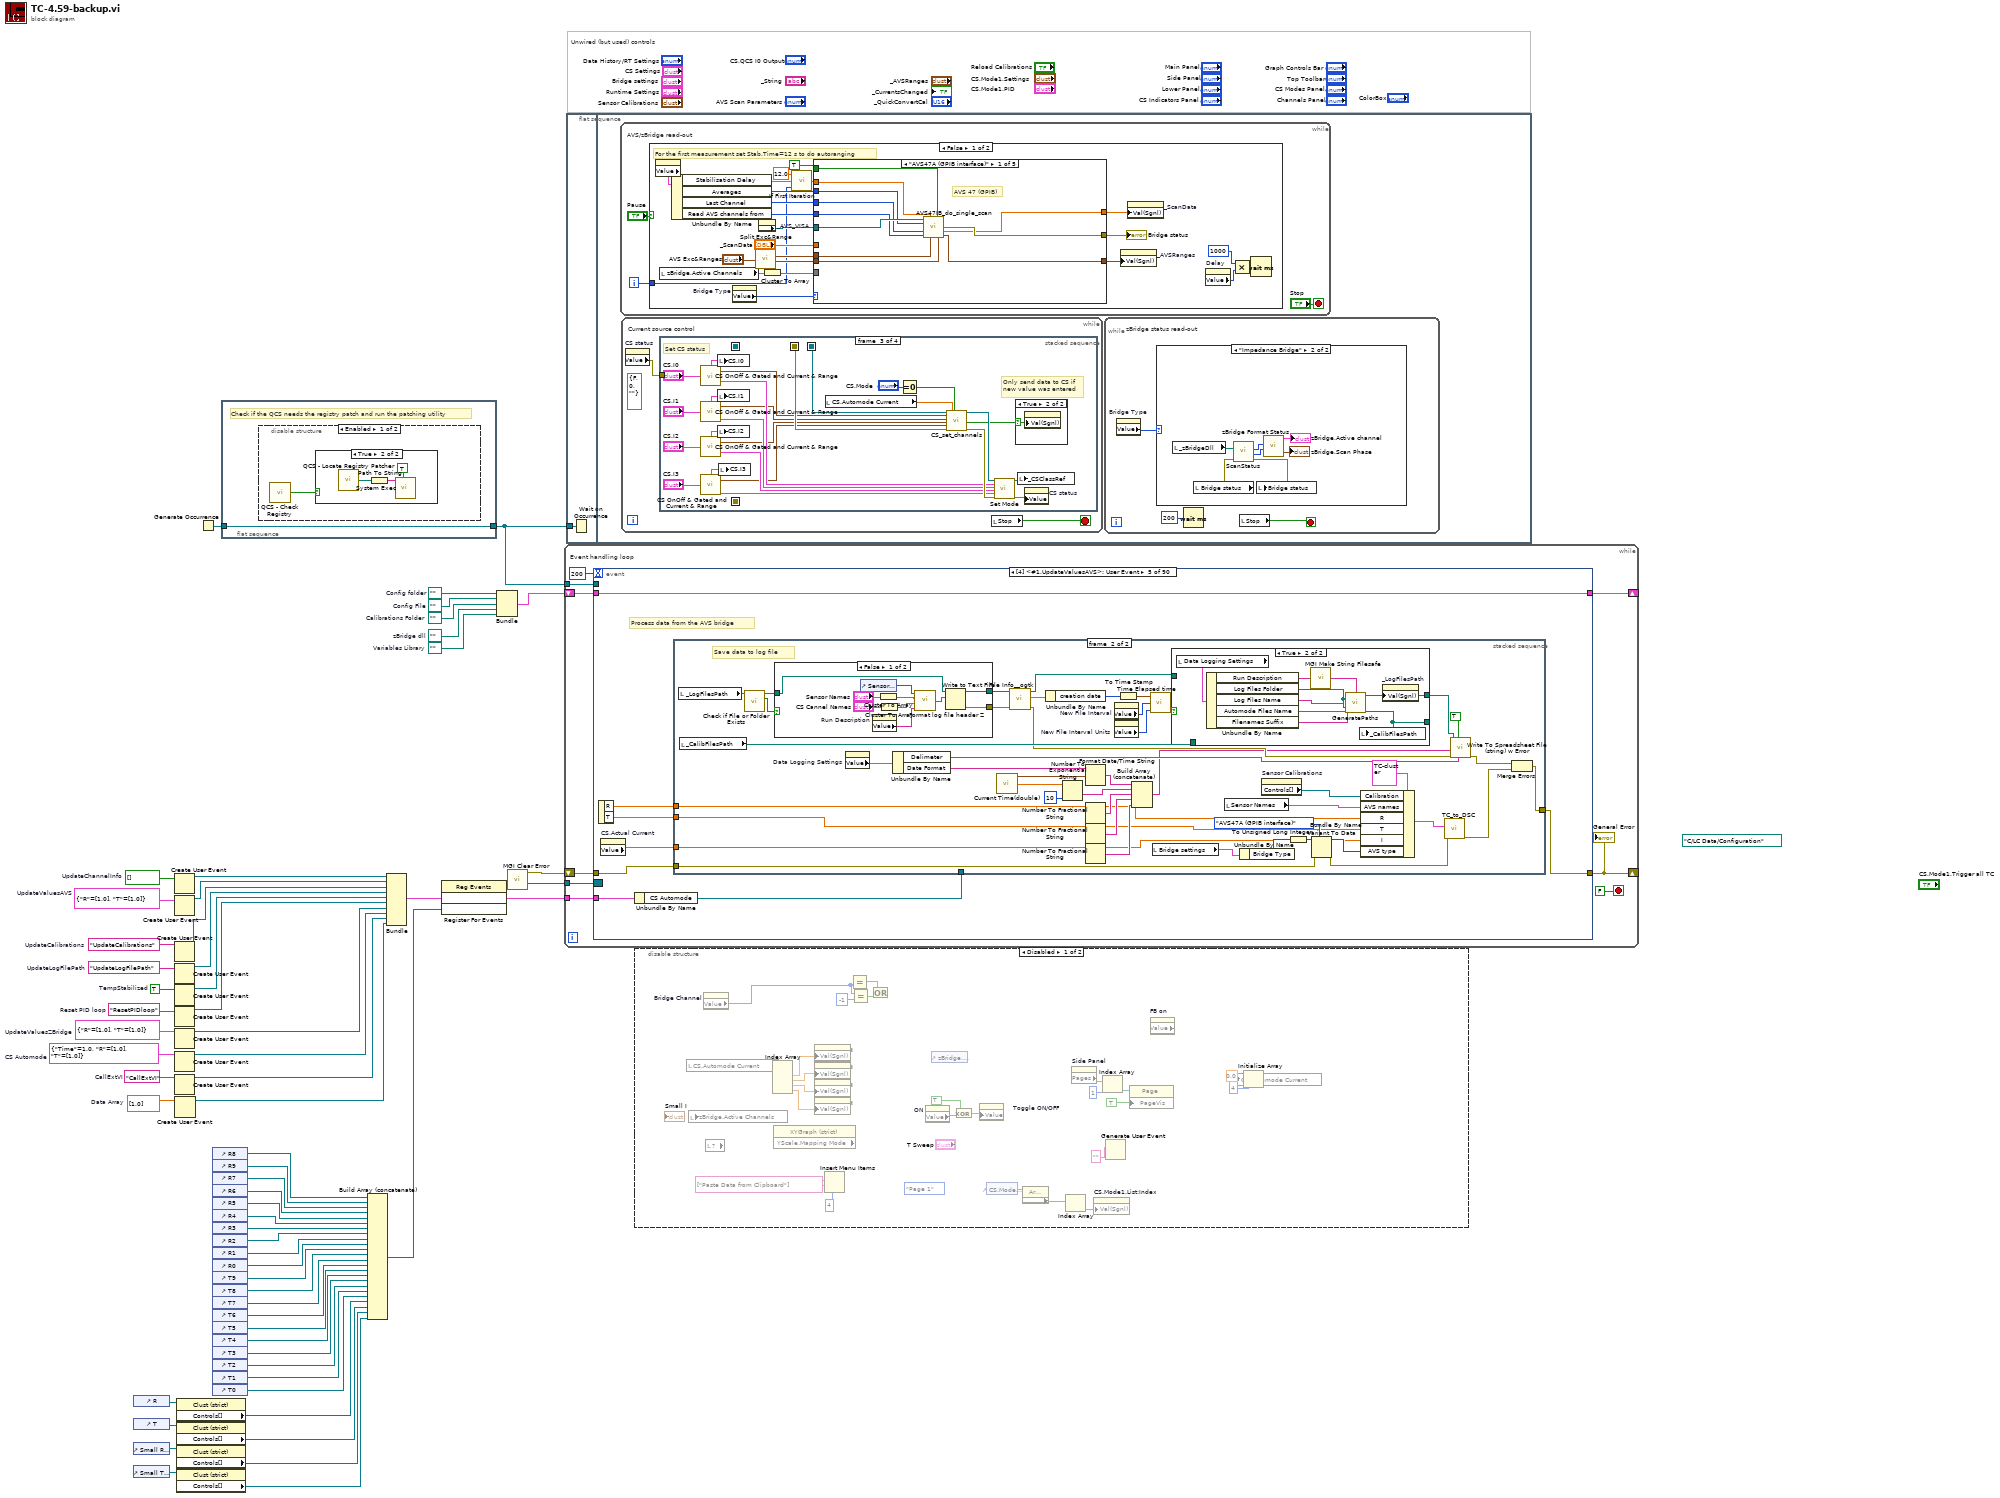
[diagram p0: block diagram]
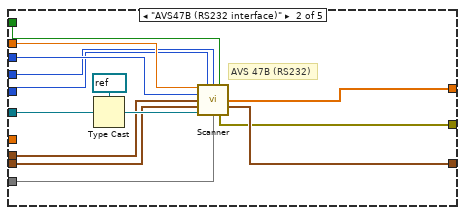
[diagram p5: hidden frame]
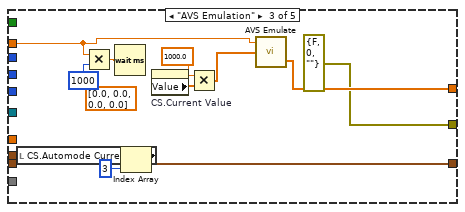
[diagram p6: hidden frame]
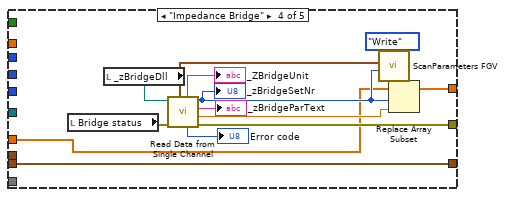
[diagram p7: hidden frame]
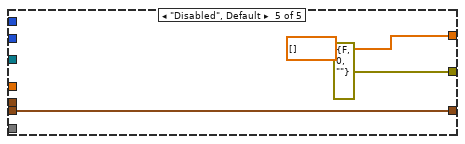
[diagram p8: hidden frame]
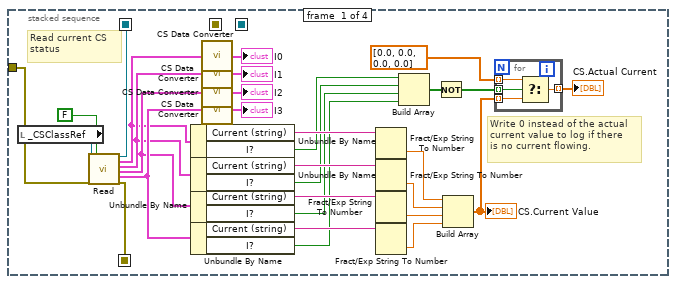
[diagram p10: hidden frame]
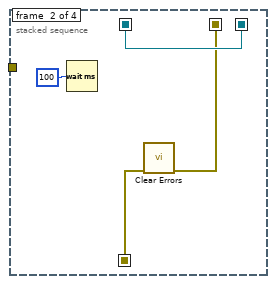
[diagram p11: hidden frame]
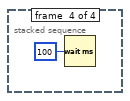
[diagram p13: hidden frame]
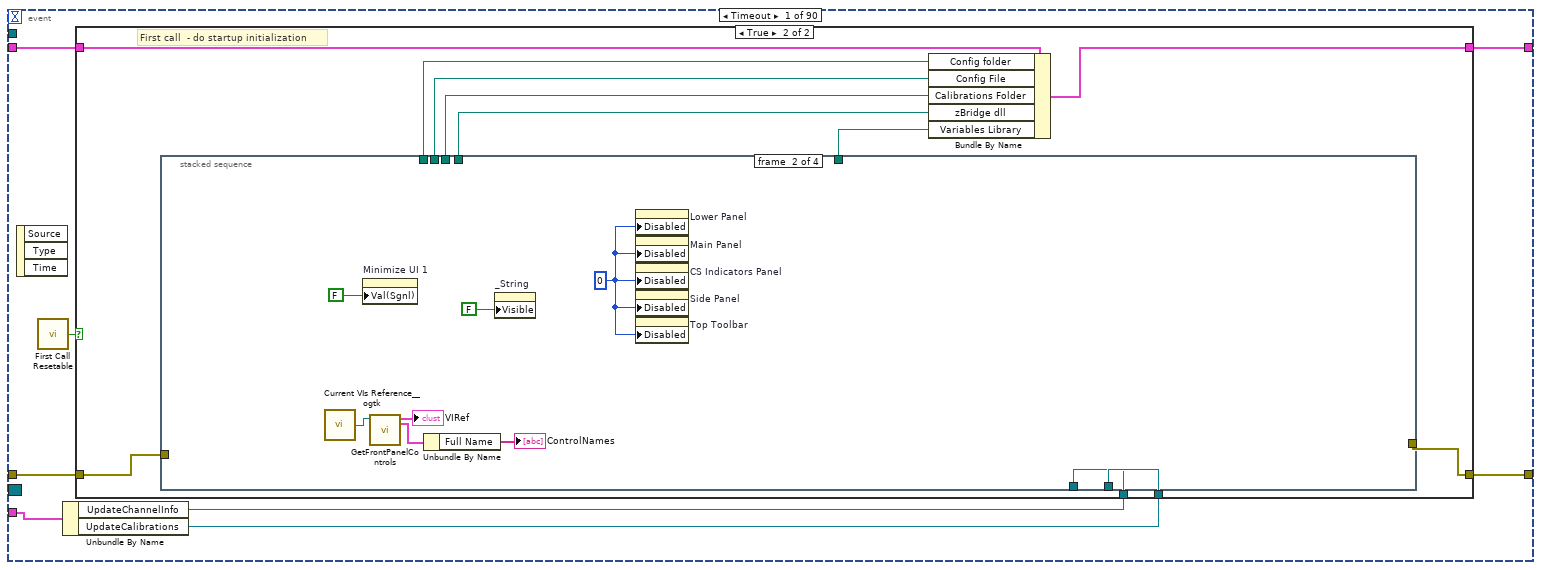
[diagram p15: hidden frame]
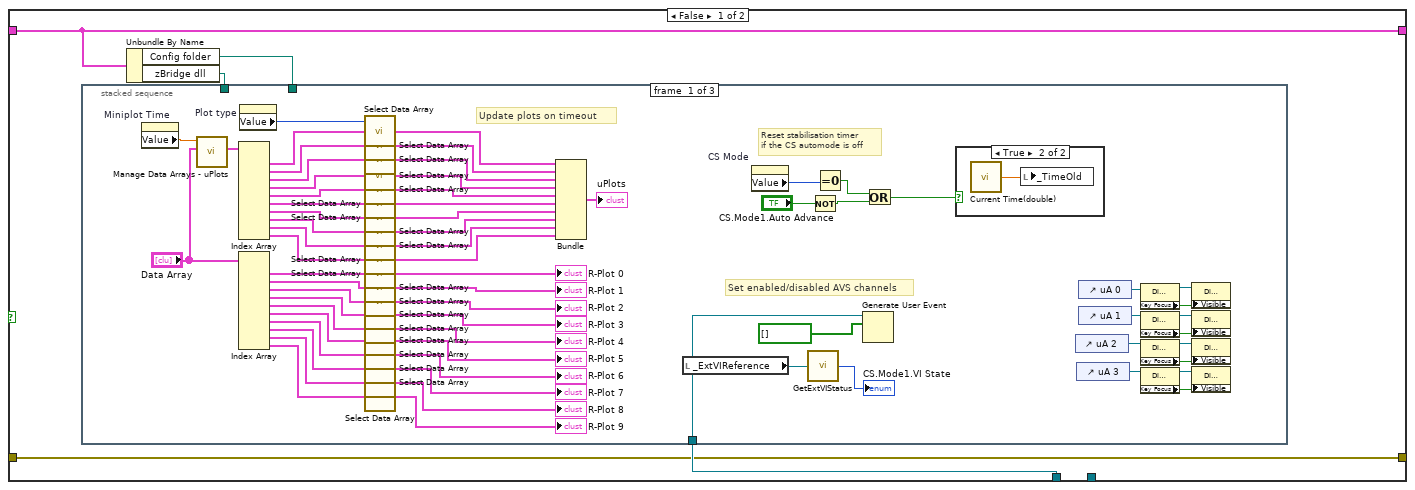
[diagram p16: hidden frame]
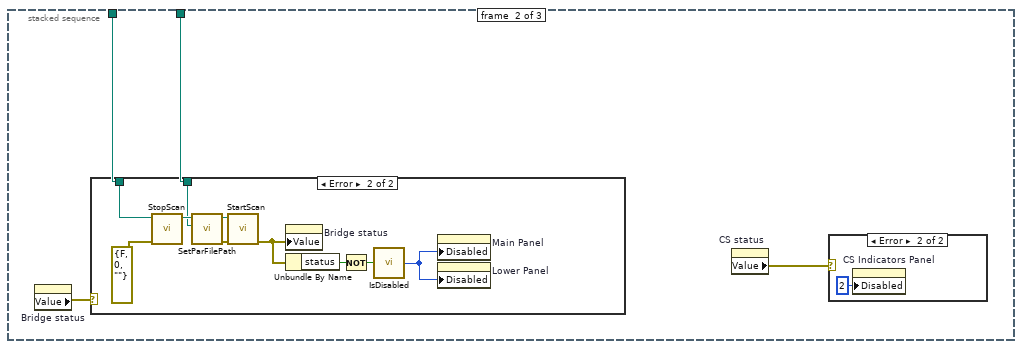
[diagram p18: hidden frame]
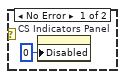
[diagram p19: hidden frame]
diagram:
  w30 = path ""  # Variables Library
  w31 = path ""  # zBridge dll
  w32 = path ""  # Calibrations Folder
  w33 = path ""  # Config File
  w35 = path ""  # Config folder
  (unwired) path "C:/LC Data/Configuration" ("Relative path (.)")
  w38 = dbl[] [1.0]  # Data Array
  w52 = "CallExtVI"  # CallExtVI
  w53 = bool[] []  # UpdateChannelInfo
  w54 = cluster{"Time":dbl, "R":dbl[], "T":dbl[]} {"Time"=1.0, "R"=[1.0], "T"=[1.0]}  # CS Automode
  w55 = cluster{"R":dbl[], "T":dbl[]} {"R"=[1.0], "T"=[1.0]}  # UpdateValuesAVS
  w56 = cluster{"R":dbl[], "T":dbl[]} {"R"=[1.0], "T"=[1.0]}  # UpdateValuesZBridge
  w57 = "ResetPIDloop"  # Reset PID loop
  w58 = TRUE  # TempStabilized
  w59 = "UpdateLogFilePath"  # UpdateLogFilePath
  w60 = "UpdateCalibrations"  # UpdateCalibrations
  # "Unwired (but used) controls"
  n1 = control-ref of="R"() -> (w29:refnum<vi>)
  n2 = control-ref of="T"() -> (w28:refnum<vi>)
  n3 = control-ref of="Small R Cluster"() -> (w4:refnum<vi>)
  n4 = control-ref of="Small T Cluster"() -> (w3:refnum<vi>)
  n5 = Create User Event(user event datatype=w53) -> (user event=w50:refnum<user-event>)  [unwired: 1 in, 1 out]
  n6 = Create User Event(user event datatype=w55) -> (user event=w49:refnum<user-event>)  [unwired: 1 in, 1 out]
  n7 = Create User Event(user event datatype=w60) -> (user event=w48:refnum<user-event>)  [unwired: 1 in, 1 out]
  n8 = Create User Event(user event datatype=w59) -> (user event=w47:refnum<user-event>)  [unwired: 1 in, 1 out]
  n9 = Create User Event ("TempStabilized")(user event datatype=w58) -> (user event=w46:refnum<user-event>)  [unwired: 1 in, 1 out]
  n10 = Create User Event(user event datatype=w57) -> (user event=w45:refnum<user-event>)  [unwired: 1 in, 1 out]
  n11 = Create User Event(user event datatype=w56) -> (user event=w44:refnum<user-event>)  [unwired: 1 in, 1 out]
  n12 = Create User Event(user event datatype=w54) -> (user event=w43:refnum<user-event>)  [unwired: 1 in, 1 out]
  n13 = Create User Event(user event datatype=w52) -> (user event=w42:refnum<user-event>)  [unwired: 1 in, 1 out]
  n14 = Create User Event(user event datatype=w38) -> (user event=w39:refnum<user-event>)  [unwired: 1 in, 1 out]
  n15 = property class="Clust (strict)"(reference=w29) -> ("Controls[]"=w7:refnum<vi>[])  [unwired: 1 in, 2 out]
  n16 = property class="Clust (strict)"(reference=w28) -> ("Controls[]"=w6:refnum<vi>[])  [unwired: 1 in, 2 out]
  n17 = property class="Clust (strict)"(reference=w4) -> ("Controls[]"=w2:refnum<vi>[])  [unwired: 1 in, 2 out]
  n18 = property class="Clust (strict)"(reference=w3) -> ("Controls[]"=w1:refnum<vi>[])  [unwired: 1 in, 2 out]
  n19 = Generate Occurrence() -> (w37:refnum<k4>)
  n20 = control-ref of="R8"() -> (w27:refnum<vi>)
  n21 = control-ref of="R9"() -> (w26:refnum<vi>)
  n22 = control-ref of="R7"() -> (w25:refnum<vi>)
  n23 = control-ref of="R6"() -> (w24:refnum<vi>)
  n24 = control-ref of="R5"() -> (w23:refnum<vi>)
  n25 = control-ref of="R4"() -> (w22:refnum<vi>)
  n26 = control-ref of="R3"() -> (w21:refnum<vi>)
  n27 = control-ref of="R2"() -> (w20:refnum<vi>)
  n28 = control-ref of="R1"() -> (w19:refnum<vi>)
  n29 = control-ref of="R0"() -> (w18:refnum<vi>)
  n30 = control-ref of="T9"() -> (w17:refnum<vi>)
  n31 = control-ref of="T8"() -> (w16:refnum<vi>)
  n32 = control-ref of="T7"() -> (w15:refnum<vi>)
  n33 = control-ref of="T6"() -> (w14:refnum<vi>)
  n34 = control-ref of="T5"() -> (w13:refnum<vi>)
  n35 = control-ref of="T4"() -> (w12:refnum<vi>)
  n36 = control-ref of="T3"() -> (w11:refnum<vi>)
  n37 = control-ref of="T2"() -> (w10:refnum<vi>)
  n38 = control-ref of="T1"() -> (w9:refnum<vi>)
  n39 = control-ref of="T0"() -> (w8:refnum<vi>)
  n40 = flat-sequence {
    tunnel: w37 -> [w61]
    tunnel: [w61] -> w36
    frame #0 {
      # "Check if the QCS needs the registry patch and run the patching utility"
      n41 = disable-structure shown="Enabled" {
        frame Enabled {
          n42 = call "QCS - Check Registry.vi"() -> ("QCS needs reset?"=w62:bool)  [unwired: 5 in]
          n43 = case shown="True" w62 {
            frame False {
            }
            frame True {
              n44 = call "QCS - Locate Registry Patcher.vi"() -> ("dup path"=w64:path)  [unwired: 5 in]
              n45 = Path To String(path=w64) -> (string=w65:string)
              n46 = call <vilib>:"System Exec.vi"("wait until completion? (T)"=TRUE, "command line"=w65) -> ()  [unwired: 6 in, 4 out]
            }
          }
        }
        frame Disabled {
        }
      }
    }
  }
  n47 = Build Array (concatenate)(w27, w26, w25, w24, w23, w22, w21, w20, w19, w18, w17, w16, w15, w14, w13, w12, w11, w10, w9, w8, w7, w6, w2, w1) -> (w5:refnum<vi>[])
  n48 = Bundle("UpdateChannelInfo"=w50, "UpdateValuesAVS"=w49, "UpdateCalibrations"=w48, "UpdateLogFilePath"=w47, "TempStabilized"=w46, "Reset PID loop"=w45, "UpdateValuesZBridge"=w44, "CS Automode"=w43, "CallExtVI"=w42, "Data Array"=w39) -> (w41:T49)  [unwired: 1 in]
  n49 = register-events(w41, w5) -> (reference out=w51:refnum<event-registration>)  [unwired: 2 in, 1 out]
  n50 = Bundle("Config folder"=w35, "Config File"=w33, "Calibrations Folder"=w32, "zBridge dll"=w31, "Variables Library"=w30) -> (w34:T50)  [unwired: 1 in]
  n51 = call "MGI Clear Error.vi"() -> ("Error Out"=w40:errorcluster)  [unwired: 7 in]
  n52 = while {
    tunnel: w51 -> [w73]
    shift-right: [w70] -> _
    shift-left: w40 -> [w71]
    tunnel: w41 -> [w69]
    tunnel: w36 -> [w68]
    shift-right: [w66] -> _
    shift-left: w34 -> [w67]
    stop <- FALSE stop-if-true
    # "Event handling loop"
    n53 = event shown="[4] <#1.UpdateValuesAVS>: User Event" {
      selector: w73 -> [_ _ _ _ _ _ _ _ _ _ _ _ _ _ _ _ _ _ _ _ _ _ _ _ _ _ _ _ _ _ _ _ _ _ _ _ _ _ _ _ _ _ _ _ _ _ _ _ _ _ _ _ _ _ _ _ _ _ _ _ _ _ _ _ _ _ _ _ _ _ _ _ _ _ _ _ _ _ _ _ _ _ _ _ _ _ _ _ _ _]
      dyn-events: _ -> [_ _ _ _ _ _ _ _ _ _ _ _ _ _ _ _ _ _ _ _ _ _ _ _ _ _ _ _ _ _ _ _ _ _ _ _ _ _ _ _ _ _ _ _ _ _ _ _ _ _ _ _ _ _ _ _ _ _ _ _ _ _ _ _ _ _ _ _ _ _ _ _ _ _ _ _ _ _ _ _ _ _ _ _ _ _ _ _ _ _]
      timeout: 200 -> [_ _ _ _ _ _ _ _ _ _ _ _ _ _ _ _ _ _ _ _ _ _ _ _ _ _ _ _ _ _ _ _ _ _ _ _ _ _ _ _ _ _ _ _ _ _ _ _ _ _ _ _ _ _ _ _ _ _ _ _ _ _ _ _ _ _ _ _ _ _ _ _ _ _ _ _ _ _ _ _ _ _ _ _ _ _ _ _ _ _]
      tunnel: w71 -> [w82 _ _ w525 w573 w663 _ _ w869 _ _ _ w998 w1007 _ _ _ _ _ _ _ _ _ w1256 _ w1265 _ _ _ _ _ _ _ _ w1370 _ _ _ _ _ _ _ _ _ _ _ _ _ _ _ _ _ _ _ _ _ _ w1796 w1816 _ _ _ _ _ w1961 _ _ _ _ _ _ _ _ _ _ _ _ _ _ _ _ _ _ _ _ _ _ _ _ _]
      tunnel: [w81 _ _ w528 w572 w658 _ _ w867 _ _ _ w997 w1007 _ _ _ _ _ _ _ _ _ w1256 _ w1265 _ _ _ _ _ _ w1352 _ w1370 _ _ _ _ _ _ _ _ _ _ _ _ _ _ _ _ _ _ _ _ _ _ w1795 w1815 _ _ _ _ _ w1961 _ _ _ _ _ _ _ _ _ _ _ _ _ _ _ _ _ _ _ _ _ _ _ _ _] -> w70
      tunnel: w69 -> [w79 _ _ w510 w568 w660 w759 w848 _ _ _ _ _ _ _ _ _ _ _ _ _ _ _ _ _ _ w1296 w1318 _ _ _ _ _ w1360 w1368 _ _ _ _ _ _ _ _ _ _ _ _ _ _ _ _ _ _ _ _ _ _ _ w1810 _ w1891 w1905 _ _ _ _ _ w1967 _ _ w1989 w2006 w2010 _ _ _ _ _ _ _ _ _ _ w2090 _ _ _ _ _ _]
      tunnel: w68 -> [_ w343 _ _ _ _ _ _ _ _ _ _ _ _ _ _ _ _ _ _ _ _ _ _ _ _ _ _ _ _ _ _ _ _ _ _ _ _ _ _ _ _ _ _ _ _ _ _ _ _ _ _ _ _ _ _ _ _ _ _ _ _ _ _ _ _ _ _ _ _ _ _ _ _ _ _ _ _ _ _ _ _ _ _ _ _ _ _ _ _]
      tunnel: w67 -> [w75 w342 w474 w506 w566 w657 w755 w846 w866 w903 w960 w988 w995 w1003 w1046 w1063 w1129 w1142 w1182 w1184 w1187 w1200 w1243 w1251 w1259 w1263 w1294 w1316 w1320 w1323 w1331 w1340 w1350 w1358 w1363 w1390 w1394 w1469 w1476 w1483 w1525 w1553 w1587 w1614 w1620 w1628 w1636 w1645 w1654 w1656 w1701 w1709 w1714 w1737 w1754 w1779 w1783 w1787 w1808 w1879 w1889 w1903 w1913 w1938 w1960 w1962 w1963 w1965 w1971 w1975 w1986 w2004 w2008 w2021 w2028 w2029 w2037 w2040 w2044 w2048 w2051 w2077 w2083 w2088 w2092 w2096 w2117 w2129 w2139 w2141]
      tunnel: [w76 w342 w474 w506 w566 w657 w755 w846 w866 w903 w960 w988 w994 w1003 w1046 w1063 w1129 w1142 w1182 w1184 w1187 w1200 w1243 w1251 w1259 w1263 w1294 w1316 w1320 w1323 w1331 w1340 w1350 w1358 w1363 w1390 w1394 w1469 w1476 w1483 w1525 w1553 w1587 w1614 w1620 w1628 w1636 w1645 w1654 w1656 w1701 w1709 w1714 w1737 w1754 w1779 w1783 w1787 w1808 w1879 w1889 w1903 w1913 w1938 w1960 w1962 w1963 w1965 w1971 w1975 w1986 w2004 w2008 w2021 w2028 w2029 w2037 w2040 w2044 w2048 w2051 w2077 w2083 w2088 w2092 w2096 w2117 w2129 w2139 w2141] -> w66
      event Timeout {
        n54 = event-data() -> ()  [unwired: 1 in, 3 out]
        n55 = call "First Call Resetable.vi"() -> ("First Call?"=w80:bool)
        n56 = Unbundle By Name(w79) -> ("UpdateChannelInfo"=w77:refnum<user-event>, "UpdateCalibrations"=w78:refnum<user-event>)
        n57 = case shown="True" w80 {
          tunnel: w82 -> [w86 w211]
          tunnel: [w86 w209] -> w81
          tunnel: w78 -> [_ w210]
          tunnel: w77 -> [w87 w208]
          tunnel: w75 -> [w85 w207]
          tunnel: [w85 w206] -> w76
          frame False {
            n58 = Unbundle By Name(w85) -> ("Config folder"=w84:path, "zBridge dll"=w83:path)
            n59 = stacked-sequence {
              tunnel: w87 -> [w88 _ _]
              tunnel: w84 -> [_ w156 _]
              tunnel: w83 -> [_ w155 _]
              frame #0 {
                # "Update plots on timeout"
                # "Set enabled/disabled AVS channels"
                # "Reset stabilisation timer\nif the CS automode is off"
                n60 = property on="Miniplot Time" class="DigNum (strict)"() -> ("Value"=w149:dbl)  [unwired: 2 in, 2 out]
                n61 = call "Manage Data Arrays - uPlots.vi"("Data In"="Data Array", "Data Memory"=w149) -> ("Data Out"=w104:T28)  [unwired: 7 in]
                n62 = Index Array(array=w104) -> (element #1=w119:cluster{"R":dbl[], "T":dbl[], "Time":dbl[]}, element #2=w120:cluster{"R":dbl[], "T":dbl[], "Time":dbl[]}, element #3=w121:cluster{"R":dbl[], "T":dbl[], "Time":dbl[]}, element #4=w122:cluster{"R":dbl[], "T":dbl[], "Time":dbl[]}, element #5=w123:cluster{"R":dbl[], "T":dbl[], "Time":dbl[]}, element #6=w124:cluster{"R":dbl[], "T":dbl[], "Time":dbl[]}, element #7=w125:cluster{"R":dbl[], "T":dbl[], "Time":dbl[]}, element #8=w126:cluster{"R":dbl[], "T":dbl[], "Time":dbl[]}, element #9=w127:cluster{"R":dbl[], "T":dbl[], "Time":dbl[]}, element #10=w128:cluster{"R":dbl[], "T":dbl[], "Time":dbl[]})  [unwired: 10 in]
                n63 = Index Array(array="Data Array") -> (element #1=w148:cluster{"R":dbl[], "T":dbl[], "Time":dbl[]}, element #2=w147:cluster{"R":dbl[], "T":dbl[], "Time":dbl[]}, element #3=w146:cluster{"R":dbl[], "T":dbl[], "Time":dbl[]}, element #4=w145:cluster{"R":dbl[], "T":dbl[], "Time":dbl[]}, element #5=w144:cluster{"R":dbl[], "T":dbl[], "Time":dbl[]}, element #6=w143:cluster{"R":dbl[], "T":dbl[], "Time":dbl[]}, element #7=w142:cluster{"R":dbl[], "T":dbl[], "Time":dbl[]}, element #8=w141:cluster{"R":dbl[], "T":dbl[], "Time":dbl[]}, element #9=w140:cluster{"R":dbl[], "T":dbl[], "Time":dbl[]}, element #10=w139:cluster{"R":dbl[], "T":dbl[], "Time":dbl[]})  [unwired: 10 in]
                n64 = property on="Plot type" class="Enum (strict)"() -> ("Value"=w107:enum16{"R vs Time", "T vs Time"})  [unwired: 2 in, 2 out]
                n65 = call "Select Data Array.vi"("Cluster 2"=w119, "Value"=w107) -> ("Cluster"=w129:cluster{"Time":dbl[], "T":dbl[]})
                n66 = call "Select Data Array.vi"("Cluster 2"=w120, "Value"=w107) -> ("Cluster"=w130:cluster{"Time":dbl[], "T":dbl[]})
                n67 = call "Select Data Array.vi"("Cluster 2"=w121, "Value"=w107) -> ("Cluster"=w131:cluster{"Time":dbl[], "T":dbl[]})
                n68 = call "Select Data Array.vi"("Cluster 2"=w122, "Value"=w107) -> ("Cluster"=w132:cluster{"Time":dbl[], "T":dbl[]})
                n69 = call "Select Data Array.vi"("Cluster 2"=w123, "Value"=w107) -> ("Cluster"=w138:cluster{"Time":dbl[], "T":dbl[]})
                n70 = call "Select Data Array.vi"("Cluster 2"=w124, "Value"=w107) -> ("Cluster"=w133:cluster{"Time":dbl[], "T":dbl[]})
                n71 = call "Select Data Array.vi"("Cluster 2"=w125, "Value"=w107) -> ("Cluster"=w134:cluster{"Time":dbl[], "T":dbl[]})
                n72 = call "Select Data Array.vi"("Cluster 2"=w126, "Value"=w107) -> ("Cluster"=w135:cluster{"Time":dbl[], "T":dbl[]})
                n73 = call "Select Data Array.vi"("Cluster 2"=w127, "Value"=w107) -> ("Cluster"=w136:cluster{"Time":dbl[], "T":dbl[]})
                n74 = call "Select Data Array.vi"("Cluster 2"=w128, "Value"=w107) -> ("Cluster"=w137:cluster{"Time":dbl[], "T":dbl[]})
                n75 = call "Select Data Array.vi"("Cluster 2"=w148, "Value"=w107) -> ("Cluster"=→"R-Plot 0":cluster{"Time":dbl[], "T":dbl[]})
                n76 = call "Select Data Array.vi"("Cluster 2"=w147, "Value"=w107) -> ("Cluster"=→"R-Plot 1":cluster{"Time":dbl[], "T":dbl[]})
                n77 = call "Select Data Array.vi"("Cluster 2"=w146, "Value"=w107) -> ("Cluster"=→"R-Plot 2":cluster{"Time":dbl[], "T":dbl[]})
                n78 = call "Select Data Array.vi"("Cluster 2"=w145, "Value"=w107) -> ("Cluster"=→"R-Plot 3":cluster{"Time":dbl[], "T":dbl[]})
                n79 = call "Select Data Array.vi"("Cluster 2"=w144, "Value"=w107) -> ("Cluster"=→"R-Plot 4":cluster{"Time":dbl[], "T":dbl[]})
                n80 = call "Select Data Array.vi"("Cluster 2"=w143, "Value"=w107) -> ("Cluster"=→"R-Plot 5":cluster{"Time":dbl[], "T":dbl[]})
                n81 = call "Select Data Array.vi"("Cluster 2"=w142, "Value"=w107) -> ("Cluster"=→"R-Plot 6":cluster{"Time":dbl[], "T":dbl[]})
                n82 = call "Select Data Array.vi"("Cluster 2"=w141, "Value"=w107) -> ("Cluster"=→"R-Plot 7":cluster{"Time":dbl[], "T":dbl[]})
                n83 = call "Select Data Array.vi"("Cluster 2"=w140, "Value"=w107) -> ("Cluster"=→"R-Plot 8":cluster{"Time":dbl[], "T":dbl[]})
                n84 = call "Select Data Array.vi"("Cluster 2"=w139, "Value"=w107) -> ("Cluster"=→"R-Plot 9":cluster{"Time":dbl[], "T":dbl[]})
                n85 = Bundle("Cluster"=w129, "Cluster"=w130, "Cluster"=w131, "Cluster"=w132, "Cluster"=w138, "Cluster"=w133, "Cluster"=w134, "Cluster"=w135, "Cluster"=w136, "Cluster"=w137) -> (→"uPlots":T59)  [unwired: 1 in]
                n86 = local read "_ExtVIReference"() -> (w103:refnum<vi>)
                n87 = property on="CS Mode" class="Enum (strict)"() -> ("Value"=w152:T39)  [unwired: 2 in, 2 out]
                n88 = call "GetExtVIStatus.vi"("vi reference in"=w103) -> ("Exec.State"=→"CS.Mode1.VI State":T46)  [unwired: 2 out]
                n89 = Not(x="CS.Mode1.Auto Advance") -> (.not. x?=w151:bool)
                n90 = Equal To 0?(x=w152) -> (x = 0?=w101:bool)
                n91 = Generate User Event(user event=w88, event data cluster=bool[] [] ("event data")) -> ()  [unwired: 2 in, 2 out]
                n92 = Or(x=w101, y=w151) -> (x .or. y?=w150:bool)
                n93 = case shown="True" w150 {
                  frame False {
                  }
                  frame True {
                    n94 = call "Current Time(double).vi"() -> ("Current Time (double)"=w154:dbl)  [unwired: 6 in, 1 out]
                    n95 = local write "_TimeOld"(w154) -> ()
                  }
                }
                n96 = control-ref of="uA 2"() -> (w89:refnum<vi>)
                n97 = control-ref of="uA 3"() -> (w90:refnum<vi>)
                n98 = control-ref of="uA 0"() -> (w100:refnum<vi>)
                n99 = control-ref of="uA 1"() -> (w96:refnum<vi>)
                n100 = property class="DigNum (strict)"(reference=w100) -> (reference out=w99:refnum<vi>, "Key Focus"=w98:bool)  [unwired: 1 in, 1 out]
                n101 = property class="DigNum (strict)"(reference=w96) -> (reference out=w97:refnum<vi>, "Key Focus"=w95:bool)  [unwired: 1 in, 1 out]
                n102 = property class="DigNum (strict)"(reference=w89) -> (reference out=w91:refnum<vi>, "Key Focus"=w92:bool)  [unwired: 1 in, 1 out]
                n103 = property class="DigNum (strict)"(reference=w90) -> (reference out=w93:refnum<vi>, "Key Focus"=w94:bool)  [unwired: 1 in, 1 out]
                n104 = property class="DigNum (strict)"(reference=w99, "Visible"=w98) -> ()  [unwired: 1 in, 2 out]
                n105 = property class="DigNum (strict)"(reference=w97, "Visible"=w95) -> ()  [unwired: 1 in, 2 out]
                n106 = property class="DigNum (strict)"(reference=w91, "Visible"=w92) -> ()  [unwired: 1 in, 2 out]
                n107 = property class="DigNum (strict)"(reference=w93, "Visible"=w94) -> ()  [unwired: 1 in, 2 out]
              }
              frame #1 {
                n108 = property on="Bridge status" class="Clust (strict)"() -> ("Value"=w158:errorcluster)  [unwired: 2 in, 2 out]
                n109 = case shown="Error" w158 {
                  tunnel: w156 -> [_ w162]
                  tunnel: w155 -> [_ w161]
                  frame No Error {
                  }
                  frame Error {
                    n110 = call "StopScan.vi"("error in (no error)"=errorcluster {"status"=FALSE, "code"=0, "source"=""}, "path in"=w161) -> ("path out"=w168:path)  [unwired: 8 in, 1 out]
                    n111 = call "SetParFilePath.vi"("path"=w162, "zDll"=w168) -> ("error out"=w170:errorcluster, "zDll out"=w169:path)  [unwired: 8 in]
                    n112 = call "StartScan.vi"("error in (no error)"=w170, "path in"=w169) -> ("error out"=w166:errorcluster)  [unwired: 8 in, 1 out]
                    n113 = property on="Bridge status" class="Clust (strict)"("Value"=w166) -> ()  [unwired: 2 in, 2 out]
                    n114 = Unbundle By Name(w166) -> ("status"=w164:bool)
                    n115 = Not(x=w164) -> (.not. x?=w165:bool)
                    n116 = call "IsDisabled.vi"("Enabled?"=w165) -> ("Numeric"=w163:i16)
                    n117 = property on="Main Panel" class="TabCtl (strict)"("Disabled"=w163) -> ()  [unwired: 2 in, 2 out]
                    n118 = property on="Lower Panel" class="TabCtl (strict)"("Disabled"=w163) -> ()  [unwired: 2 in, 2 out]
                  }
                }
                n119 = property on="CS status" class="Clust (strict)"() -> ("Value"=w157:errorcluster)  [unwired: 2 in, 2 out]
                n120 = case shown="Error" w157 {
                  frame No Error {
                    n121 = property on="CS Indicators Panel" class="TabCtl (strict)"("Disabled"=u8 0) -> ()  [unwired: 2 in, 2 out]
                  }
                  frame Error {
                    n122 = property on="CS Indicators Panel" class="TabCtl (strict)"("Disabled"=u8 2) -> ()  [unwired: 2 in, 2 out]
                  }
                }
              }
              frame #2 {
                # "Check if the structure is \nnot empty and only one\nof Scalar or Array is set"
                # "Set FP control value from external script/program"
                n123 = local read "_SetControl"() -> (w171:T1)
                n124 = Unbundle By Name(w171) -> ("Name"=w173:string, "Scalar"=w172:string, "Array"=w181:string[][])
                n125 = call "Empty 2D Array (String)__ogtk.vi"("Array"=w181) -> ("Empty Array?"=w178:bool)  [unwired: 8 in]
                n126 = Empty String/Path?(string/path=w173) -> (empty?=w177:bool)
                n127 = Empty String/Path?(string/path=w172) -> (empty?=w176:bool)
                n128 = Not(x=w177) -> (.not. x?=w175:bool)
                n129 = Not(x=w176) -> (.not. x?=w179:bool)
                n130 = Not(x=w178) -> (.not. x?=w182:bool)
                n131 = Exclusive Or(1:w182, 2:w179) -> (0:w180:bool)
                n132 = And(x=w175, y=w180) -> (x .and. y?=w174:bool)
                n133 = case shown="True" w174 {
                  tunnel: w173 -> [_ w186]
                  tunnel: w172 -> [_ w185]
                  tunnel: w181 -> [_ w184]
                  tunnel: w182 -> [_ w183]
                  frame False {
                  }
                  frame True {
                    n134 = flat-sequence {
                      tunnel: w186 -> [w190]
                      tunnel: w185 -> [w189]
                      tunnel: w184 -> [w187]
                      tunnel: w183 -> [w188]
                      frame #0 {
                        n135 = local read "VIRef"() -> (w191:T2)
                        n136 = case shown="False" w188 {
                          tunnel: w191 -> [w194 w197]
                          tunnel: w190 -> [w193 w196]
                          tunnel: w189 -> [w192 _]
                          tunnel: w187 -> [_ w195]
                          frame False {
                            n137 = call "Push2VI.vi"("New Value"=w192, "element"=w193, "VIRef"=w194) -> ()  [unwired: 8 in, 1 out]
                          }
                          frame True {
                            n138 = call "PushArray2VI.vi"("Str"=w195, "element"=w196, "VIRef"=w197) -> ()  [unwired: 8 in, 1 out]
                          }
                        }
                      }
                      frame #1 {
                        w199 = ""
                        n139 = Bundle(w199, w199, "Array"=string[][] []) -> (→"_SetControl":cluster{string, string, "Array":string[][]})  [unwired: 1 in]
                      }
                    }
                  }
                }
              }
            }
          }
          frame True {
            # "First call  - do startup initialization"
            n140 = stacked-sequence {
              tunnel: w211 -> [_ _ w256 _]
              tunnel: [_ _ w250 _] -> w209
              tunnel: w210 -> [_ _ w252 _]
              tunnel: w208 -> [_ _ _ w310]
              tunnel: [_ _ w248 _] -> w205
              tunnel: [_ _ w249 _] -> w204
              tunnel: [_ _ w247 _] -> w203
              tunnel: [_ _ w245 _] -> w202
              tunnel: [w212 _ _ _] -> w201
              frame #0 {
                # "Set control bindings"
                # "\\\\localhost\\DR TempControl\\Currents(In)"
                # "\\\\localhost\\DR TempControl\\Temperatures"
                # "\\\\localhost\\DR TempControl\\Resistances"
                # "\\\\localhost\\DR TempControl\\Currents(Out)"
                n141 = disable-structure shown="RUN_TIME_ENGINE==True" {
                  disable-tunnel: [w225 "\\\\localhost\\DR TempControl\\"] -> w213
                  disable-tunnel: [w222 w235] -> w212
                  frame condition #0 {
                    w232 = u16 0 items=["overwrite", "ask first", "don't overwrite"] ("overwrite")
                    # "Deploy the shared variable library. If there are few copies of the program\nrunning - generate unique name for every copy."
                    n142 = call "Enum Variables.vi"("regular expression"="DR TempControl.*") -> ("Containers"=w230:string[])  [unwired: 15 in, 3 out]
                    n143 = call "Generate New Name.vi"("Existing names"=w230, "Base Name"="DR TempControl") -> ("New Name (path)"=w227:path, "New Name"=w226:string)  [unwired: 16 in]
                    n144 = call "Temporary Directory__ogtk.vi"("Relative path (.)"=w227) -> ("Temporary Directory (+ Relative)"=w231:path)
                    n145 = call "Current VIs Parent Directory__ogtk.vi"("Relative path (.)"=path "DR TempControl.lvlib" ("Library Path")) -> ("Parent Directory (+ Relative)"=w233:path)  [unwired: 4 in]
                    n146 = call <vilib>:"Librarian Copy.vi"("source"=w233, "overwrite"=w232, "destination"=w231) -> ("dup destination"=w222:path)  [unwired: 7 in, 1 out]
                    n147 = invoke class="App" method="Library.Deploy Library"("libPath"=w222) -> ()  [unwired: 4 in, 5 out]
                    n148 = Concatenate Strings("\\\\localhost\\" ("string"), w226, "\\" ("string")) -> (w225:string)
                  }
                  frame condition #1 (active) {
                    # "Default library is deployed automatically in development environment"
                    n149 = call "Current VIs Parent Directory__ogtk.vi"("Relative path (.)"=path "DR TempControl.lvlib" ("Library Path")) -> ("Parent Directory (+ Relative)"=w235:path)  [unwired: 4 in]
                  }
                }
                n150 = Concatenate Strings(w213, "Resistances" ("string")) -> (w219:string)
                n151 = Concatenate Strings(w213, "Temperatures" ("string")) -> (w216:string)
                n152 = Concatenate Strings(w213, "Currents(Out)" ("string")) -> (w215:string)
                n153 = Concatenate Strings(w213, "Currents(In)" ("string")) -> (w214:string)
                n154 = property on="R Array" class="Arr (strict)"("FPB.URL"=w219) -> ()  [unwired: 2 in, 2 out]
                n155 = property on="T Array" class="Arr (strict)"("FPB.URL"=w216) -> ()  [unwired: 2 in, 2 out]
                n156 = property on="CS.Actual Current" class="Arr (strict)"("FPB.URL"=w215) -> ()  [unwired: 2 in, 2 out]
                n157 = property on="CS.Automode Current" class="Arr (strict)"("FPB.URL"=w214) -> ()  [unwired: 2 in, 2 out]
              }
              frame #1 {
                w243 = u8 0 ("Disabled")
                n158 = call "Current VIs Reference__ogtk.vi"() -> ("Current VI's reference"=w241:refnum<vi>)  [unwired: 5 in]
                n159 = property on="Minimize UI 1" class="Bool (strict)"("Val(Sgnl)"=FALSE ("Value (Signaling)")) -> ()  [unwired: 2 in, 2 out]
                n160 = call "GetFrontPanelControls.vi"("Ref to VI"=w241) -> ("VIRef"=w240:T2)  [unwired: 9 in, 1 out]
                "VIRef" <- w240
                n161 = Unbundle By Name(w240) -> ("Full Name"=→"ControlNames":string[])
                n162 = property on="_String" class="Str"("Visible"=FALSE) -> ()  [unwired: 2 in, 2 out]
                n163 = property on="Lower Panel" class="TabCtl (strict)"("Disabled"=w243) -> ()  [unwired: 2 in, 2 out]
                n164 = property on="Main Panel" class="TabCtl (strict)"("Disabled"=w243) -> ()  [unwired: 2 in, 2 out]
                n165 = property on="CS Indicators Panel" class="TabCtl (strict)"("Disabled"=w243) -> ()  [unwired: 2 in, 2 out]
                n166 = property on="Side Panel" class="TabCtl (strict)"("Disabled"=w243) -> ()  [unwired: 2 in, 2 out]
                n167 = property on="Top Toolbar" class="TabCtl (strict)"("Disabled"=w243) -> ()  [unwired: 2 in, 2 out]
              }
              frame #2 {
                # "Read settings from the config file"
                n168 = flat-sequence {
                  tunnel: w256 -> [w257]
                  tunnel: [w257] -> w251
                  tunnel: [w260] -> w249
                  tunnel: [w261] -> w248
                  tunnel: [w262] -> w247
                  tunnel: [w261] -> w246
                  tunnel: [w258] -> w245
                  tunnel: [w277] -> w255
                  tunnel: w251 -> [w276]
                  tunnel: w246 -> [w278]
                  tunnel: w255 -> [w288]
                  tunnel: [w288] -> w254
                  tunnel: [w292] -> w253
                  tunnel: w254 -> [w289]
                  tunnel: w253 -> [w297]
                  tunnel: [w297] -> w244
                  tunnel: [w301] -> w250
                  tunnel: w252 -> [w298]
                  tunnel: w244 -> [w299]
                  frame #0 {
                    w263 = path "C:/LC Data" ("LC Data")
                    n169 = call "Generate config file path.vi"("LC data path"=w263) -> ("Config folder"=w262:path)  [unwired: 18 in]
                    n170 = call "Build Path - Traditional__ogtk.vi"("name or relative path"="config.ini", "base path"=w262) -> ("appended path"=w261:path)
                    n171 = call "Build Path - Traditional__ogtk.vi"("name or relative path"="Calibrations", "base path"=w263) -> ("appended path"=w260:path)
                    n172 = property on="Calibrations Folder" class="Path"("Value"=w260) -> ()  [unwired: 2 in, 2 out]
                    n173 = call "Current VIs Parent Directory__ogtk.vi"("Relative path (.)"=path "data/ImpBridgeDll.dll" ("Library Path")) -> ("Parent Directory (+ Relative)"=w258:path)  [unwired: 4 in]
                    "_zBridgeDll" <- w258
                  }
                  frame #1 {
                    n174 = control-ref of="zBridge.Active Channels"() -> (w275:refnum<vi>)
                    n175 = control-ref of="CS Settings"() -> (w274:refnum<vi>)
                    n176 = control-ref of="Bridge settings"() -> (w273:refnum<vi>)
                    n177 = control-ref of="Runtime Settings"() -> (w272:refnum<vi>)
                    n178 = control-ref of="Data Logging Settings"() -> (w271:refnum<vi>)
                    n179 = control-ref of="PID setup"() -> (w270:refnum<vi>)
                    n180 = control-ref of="CS Cannel Names"() -> (w284:refnum<vi>)
                    n181 = control-ref of="AVS names"() -> (w266:refnum<vi>)
                    n182 = control-ref of="_CurCalibrations"() -> (w267:refnum<vi>)
                    n183 = control-ref of="CS.Mode1.PID"() -> (w268:refnum<vi>)
                    n184 = control-ref of="CS.Mode1.Settings"() -> (w269:refnum<vi>)
                    n185 = call "Current VIs Parent Directory__ogtk.vi"("Relative path (.)"=path "data/config.ini") -> ("Parent Directory (+ Relative)"=w281:path)  [unwired: 4 in]
                    n186 = Build Array(w275, w274, w273, w272, w271, w270, w284, w266, w267, w268, w269) -> (w280:refnum<vi>[])
                    n187 = call "Save Load Settings to File by Ref with path.vi"("Array of Cluster References"=w280, "Action"=enum8{"Load", "Save"}."Load", "error in (no error)"=w276, "Configuration file"=w281) -> ("error out"=w283:errorcluster)  [unwired: 5 in]
                    n188 = call "MGI Clear Error.vi"("Error In"=w283) -> ("Error Out"=w282:errorcluster)  [unwired: 6 in]
                    n189 = call "Save Load Settings to File by Ref with path.vi"("Array of Cluster References"=w280, "Action"=enum8{"Load", "Save"}."Load", "error in (no error)"=w282, "Configuration file"=w278) -> ("error out"=w277:errorcluster)  [unwired: 5 in]
                  }
                  frame #2 {
                    n190 = Wait (ms)(milliseconds to wait=250) -> ()  [unwired: 1 out]
                  }
                  frame #3 {
                    n191 = control-ref of="Sensor Calibrations"() -> (w291:refnum<vi>)
                    n192 = control-ref of="_CurCalibrations"() -> (w290:refnum<vi>)
                    n193 = control-ref of="Calibrations Folder"() -> (w294:refnum<vi>)
                    n194 = control-ref of="_QuickConvertCal"() -> (w293:refnum<vi>)
                    n195 = control-ref of="Sensor 1"() -> (w295:refnum<vi>)
                    n196 = call "ReloadCalibrations.vi"("error in (no error)"=w289, "Quick convert sensors"=w293, "CurCalibrations"=w290, "Calibration files path"=w294, "Channel1 sensors"=w295, "Channels list"=w291) -> ("error out"=w292:errorcluster)  [unwired: 1 in]
                  }
                  frame #4 {
                    n197 = Wait (ms)(milliseconds to wait=250) -> ()  [unwired: 1 out]
                  }
                  frame #5 {
                    n198 = Generate User Event(user event=w298, event data cluster="" ("event data"), error in=w299) -> (error out=w301:errorcluster)  [unwired: 1 in, 1 out]
                  }
                }
              }
              frame #3 {
                w302 = FALSE ("Mode1 ON")
                w320 = u8 0 ("Disabled")
                # "Set enabled/disabled AVS channels"
                # "Reset pid parameters"
                # "Print VI version in the low left corner"
                # "Reset Current lists\nto first element"
                # "Hardware settings"
                # "Reset currents lists"
                # "Set initial controls state"
                n199 = call "Currents-Temp list - check ranges.vi"() -> ("I_list out"=w313:dbl[][])  [unwired: 5 in]
                n200 = property on="Start" class="Bool (strict)"("Visible"=TRUE, "Disabled"=u8 0, "Value"=FALSE ("start")) -> ()  [unwired: 2 in, 2 out]
                n201 = property on="CS.Mode1.List:Index" class="DigNum (strict)"("Val(Sgnl)"=1 ("Value (Signaling)")) -> ()  [unwired: 2 in, 2 out]
                n202 = property on="CS Mode" class="Enum (strict)"("Val(Sgnl)"=CS_mode."Manual" ("CS Mode")) -> ()  [unwired: 2 in, 2 out]
                n203 = local write "CS.Mode2.List"(w313) -> ()
                n204 = property on="CS.Mode1.List:To First" class="Bool (strict)"("Val(Sgnl)"=TRUE ("Value (Signaling)")) -> ()  [unwired: 2 in, 2 out]
                n205 = property on="CS.Mode1.Start" class="Bool (strict)"("Value"=w302) -> ()  [unwired: 2 in, 2 out]
                n206 = property on="CS.Mode2.Start" class="Bool (strict)"("Value"=w302) -> ()  [unwired: 2 in, 2 out]
                n207 = property on="CS.QCS I0 Output" class="Enum (strict)"("Disabled"=u8 2, "Val(Sgnl)"=T38."Channel 0" ("Map Channel 0 to")) -> ()  [unwired: 2 in, 2 out]
                n208 = property on="Bridge Type" class="Enum (strict)"("Disabled"=w320) -> ()  [unwired: 2 in, 2 out]
                n209 = property on="AVS GPIB Address" class="VISAName"("Disabled"=w320) -> ()  [unwired: 2 in, 2 out]
                n210 = property on="TCS RS232 Port" class="VISAName"("Disabled"=w320) -> ()  [unwired: 2 in, 2 out]
                n211 = property on="CS type" class="Enum (strict)"("Disabled"=w320) -> ()  [unwired: 2 in, 2 out]
                n212 = property on="CS.QCS Device Nr" class="DigNum (strict)"("Disabled"=w320) -> ()  [unwired: 2 in, 2 out]
                n213 = property on="Side Panel" class="TabCtl (strict)"("Value"=T34."Devices Settings" ("Tab Control 2")) -> ("Pages"=w307:refnum<vi>[])  [unwired: 2 in, 2 out]
                n214 = Index Array(array=w307, index=1) -> (element=w304:refnum<vi>)
                n215 = property class="App"() -> ("App.Kind"=w316:T60)  [unwired: 2 in, 2 out]
                n216 = property class="Page"(reference=w304, "PageEnb"=T51."Page Disabled & Grayed" ("Page Enabled State")) -> ()  [unwired: 1 in, 2 out]
                n217 = case shown="\"Run Time System\"" w316 {
                  tunnel: [w325 w336] -> w317
                  frame "invalid app kind", Default {
                    n218 = control-ref of="This VI"() -> (w332:refnum<vi>)
                    n219 = property class="VI"(reference=w332) -> ("Hist.Revision"=w331:u32)  [unwired: 1 in, 2 out]
                    n220 = Divide(x=w331, y=1000.0 ("x")) -> (x/y=w327:dbl)
                    n221 = Number To Fractional String(use system decimal point (T)=FALSE, number=w327, precision (6)=i16 2) -> (F-format string=w326:string)  [unwired: 1 in]
                    n222 = Concatenate Strings("" ("string"), w326) -> (w325:string)
                  }
                  frame "Run Time System" {
                    n223 = Current VI's Path() -> (path=w338:path)
                    n224 = Strip Path(path=w338) -> (stripped path=w337:path)  [unwired: 1 out]
                    n225 = Path To String(path=w337) -> (string=w335:string)
                    n226 = invoke class="FileVersionInfo" method="GetVersionInfo"(reference=refnum<k24> refnum (".NET object"), "fileName"=w335) -> ("GetVersionInfo"=w334:refnum<k24>)  [unwired: 2 in, 3 out]
                    n227 = property class="FileVersionInfo"(reference=w334) -> ("FileVersion"=w336:string)  [unwired: 1 in, 2 out]
                  }
                }
                "VI Version" <- w317
                n228 = property on="Channels Panel" class="TabCtl (strict)"("Val(Sgnl)"=T8."All" ("Value (Signaling)")) -> ()  [unwired: 2 in, 2 out]
                n229 = local write "CS.Mode1.PID Error"(0.0 ("T_error")) -> ()
                n230 = Generate User Event(user event=w310, event data cluster=bool[] [] ("event data")) -> ()  [unwired: 2 in, 2 out]
              }
            }
            n231 = Bundle By Name(cluster=w207, "Config folder"=w203, "Config File"=w205, "Calibrations Folder"=w204, "zBridge dll"=w202, "Variables Library"=w201) -> (w206:T50)
          }
        }
      }
      event "Start": Value Change {
        # "\"Start\" button clicked -> start measuring"
        n232 = event-data() -> ()  [unwired: 1 in, 6 out]
        n233 = Unbundle By Name(w342) -> ("Config File"=w339:path, "zBridge dll"=w340:path, "Config folder"=w341:path)
        n234 = stacked-sequence {
          tunnel: w343 -> [_ _ _ _ _ _ w470]
          tunnel: w341 -> [_ _ _ _ w412 _ _]
          tunnel: w340 -> [_ _ _ _ w411 _ _]
          tunnel: w339 -> [_ w353 _ _ _ _ _]
          frame #0 {
            n235 = property on="Run Description" class="Str"() -> ("Value"=w346:string)  [unwired: 2 in, 2 out]
            n236 = property on="Query Description" class="Bool (strict)"() -> ("Value"=w345:bool)  [unwired: 2 in, 2 out]
            n237 = Not(x=w345) -> (.not. x?=w344:bool)
            n238 = call "Run Reference DLG.vi"("Enable"=w345, "Run Reference"=w346, "Dont' ask again"=w344) -> ("Dont' ask again"=w348:bool, "Run Reference"=w349:string, "OK"=w350:bool)  [unwired: 13 in, 1 out]
            n239 = Not(x=w348) -> (.not. x?=w347:bool)
            n240 = case shown="True" w350 {
              tunnel: w349 -> [_ w352]
              tunnel: w347 -> [_ w351]
              frame False {
              }
              frame True {
                n241 = property on="Run Description" class="Str"("Val(Sgnl)"=w352) -> ()  [unwired: 2 in, 2 out]
                n242 = property on="Query Description" class="Bool (strict)"("Val(Sgnl)"=w351) -> ()  [unwired: 2 in, 2 out]
              }
            }
          }
          frame #1 {
            # "Save new settings to config file"
            n243 = control-ref of="zBridge.Active Channels"() -> (w357:refnum<vi>)
            n244 = control-ref of="CS.Mode1.PID"() -> (w356:refnum<vi>)
            n245 = control-ref of="CS.Mode1.Settings"() -> (w355:refnum<vi>)
            n246 = control-ref of="CS.Mode1.Settings"() -> (w354:refnum<vi>)
            n247 = control-ref of="CS Cannel Names"() -> (w360:refnum<vi>)
            n248 = control-ref of="AVS names"() -> (w359:refnum<vi>)
            n249 = control-ref of="_CurCalibrations"() -> (w358:refnum<vi>)
            n250 = control-ref of="Bridge settings"() -> (w365:refnum<vi>)
            n251 = control-ref of="Runtime Settings"() -> (w366:refnum<vi>)
            n252 = control-ref of="CS Settings"() -> (w364:refnum<vi>)
            n253 = control-ref of="Sensor Calibrations"() -> (w367:refnum<vi>)
            n254 = control-ref of="PID setup"() -> (w368:refnum<vi>)
            n255 = control-ref of="Data Logging Settings"() -> (w363:refnum<vi>)
            n256 = Build Array(w357, w365, w366, w364, w363, w367, w368, w360, w359, w358, w356, w355, w354) -> (w361:refnum<vi>[])
            n257 = call "Save Load Settings to File by Ref with path.vi"("Array of Cluster References"=w361, "Action"=enum8{"Load", "Save"}."Save", "Configuration file"=w353) -> ()  [unwired: 6 in, 1 out]
          }
          frame #2 {
            w384 = u8 2 ("Disabled")
            # "Reset stop button"
            # "Hide Disable Start button"
            # "Load external calibration VI"
            # "Set controls\nInitialize data for run"
            # "Lock hardware settings"
            n258 = property on="Bridge Type" class="Enum (strict)"("Disabled"=w384) -> ()  [unwired: 2 in, 2 out]
            n259 = property on="AVS GPIB Address" class="VISAName"("Disabled"=w384) -> ()  [unwired: 2 in, 2 out]
            n260 = property on="AVS RS232 Port" class="VISAName"("Disabled"=w384) -> ()  [unwired: 2 in, 2 out]
            n261 = property on="TCS RS232 Port" class="VISAName"("Disabled"=w384) -> ()  [unwired: 2 in, 2 out]
            n262 = property on="CS type" class="Enum (strict)"("Disabled"=w384) -> ()  [unwired: 2 in, 2 out]
            n263 = property on="CS.QCS Device Nr" class="DigNum (strict)"("Disabled"=w384) -> ()  [unwired: 2 in, 2 out]
            n264 = property on="CS.QCS I0 Output" class="Enum (strict)"("Disabled"=u8 0) -> ()  [unwired: 2 in, 2 out]
            n265 = call "Current Time(double).vi"() -> ("Current Time (double)"=w373:dbl)  [unwired: 6 in, 1 out]
            n266 = local write "_TimeOld"(w373) -> ()
            n267 = property on="External VI Path" class="Path"() -> ("Value"=w383:path)  [unwired: 2 in, 2 out]
            n268 = vi-ref "OnTempStabilizedRef.vi"() -> (w382:refnum<vi>)
            n269 = local write "VI called?"(FALSE ("VI called?")) -> ()
            n270 = Open VI Reference(type specifier VI Refnum (for type only)=w382, vi path=w383) -> (vi reference=→"_ExtVIReference":refnum<vi>)  [unwired: 4 in, 1 out]
            n271 = property on="Start" class="Bool (strict)"("Visible"=TRUE, "Disabled"=u8 2) -> ()  [unwired: 2 in, 2 out]
            n272 = Initialize Array(cluster{"R":dbl[], "T":dbl[], "Time":dbl[]} {"R"=[], "T"=[], "Time"=[]}, 10 ("dimension size")) -> (w377:cluster{"R":dbl[], "T":dbl[], "Time":dbl[]}[])
            n273 = local write "Data Array"(w377) -> ()
            n274 = disable-structure shown="Enabled" {
              frame Enabled {
                n275 = property on="Stop" class="Bool (strict)"("Value"=FALSE ("MainStopButton")) -> ()  [unwired: 2 in, 2 out]
              }
              frame Disabled {
              }
            }
            n276 = property on="Side Panel" class="TabCtl (strict)"() -> ("Pages"=w372:refnum<vi>[])  [unwired: 2 in, 2 out]
            n277 = Index Array(array=w372, index=1) -> (element=w370:refnum<vi>)
            n278 = property class="Page"(reference=w370, "PageEnb"=T51."Page Enabled" ("Page Enabled State")) -> ()  [unwired: 1 in, 2 out]
          }
          frame #3 {
            # "Initialize CS"
            n279 = local read "_CSClassRef"() -> (w396:refnum<class "CS.lvclass">)
            n280 = call-dynamic "Initialize.vi"("CS in"=w396, "HW Address"="_CS_Address", "error in (no error)"=T52 {"error"=FALSE, "code"=0, "source"=""} ("error in")) -> ("CS out"=w389:refnum<class "CS.lvclass">, "Instrument ID"=→"CS.ID":string, "error out"=w388:errorcluster)  [unwired: 10 in]
            n281 = call-dynamic "Get Currents & Ranges.vi"("CS.lvclass in"=w389, "error in (no error)"=w388) -> ("CS.lvclass out"=w397:refnum<class "CS.lvclass">, "I0"=w398:cluster{"Value":dbl, "Range":dbl}, "I1"=w390:cluster{"Value":dbl, "Range":dbl}, "I2"=w391:cluster{"Value":dbl, "Range":dbl}, "I3"=w392:cluster{"Value":dbl, "Range":dbl}, "error out"=w394:errorcluster)  [unwired: 12 in]
            "CS status" <- w394
            n282 = local write "_CSClassRef"(w397) -> ()
            n283 = Unbundle By Name(w394) -> ("status"=w386:bool)
            n284 = case shown="False" w386 {
              tunnel: w390 -> [w410 _]
              tunnel: w391 -> [w409 _]
              tunnel: w392 -> [w408 _]
              tunnel: w398 -> [w402 _]
              frame False {
                n285 = Unbundle By Name(w402) -> ("Value"=w401:dbl, "Range"=w400:dbl)
                n286 = Unbundle By Name(w410) -> ("Value"=w407:dbl, "Range"=w406:dbl)
                n287 = Unbundle By Name(w409) -> ("Value"=w405:dbl, "Range"=w404:dbl)
                n288 = Unbundle By Name(w408) -> ("Value"=w399:dbl, "Range"=w403:dbl)
                n289 = property on="I" class="DigNum (strict)"("Value"=w401) -> ()  [unwired: 2 in, 2 out]
                n290 = property on="I" class="DigNum (strict)"("Value"=w407) -> ()  [unwired: 2 in, 2 out]
                n291 = property on="I" class="DigNum (strict)"("Value"=w405) -> ()  [unwired: 2 in, 2 out]
                n292 = property on="I" class="DigNum (strict)"("Value"=w399) -> ()  [unwired: 2 in, 2 out]
                n293 = property on="Range" class="Enum (strict)"("Value"=w400) -> ()  [unwired: 2 in, 2 out]
                n294 = property on="Range" class="Enum (strict)"("Value"=w406) -> ()  [unwired: 2 in, 2 out]
                n295 = property on="Range" class="Enum (strict)"("Value"=w404) -> ()  [unwired: 2 in, 2 out]
                n296 = property on="Range" class="Enum (strict)"("Value"=w403) -> ()  [unwired: 2 in, 2 out]
              }
              frame True {
              }
            }
          }
          frame #4 {
            # "Initialize AVS/zBridge"
            n297 = property on="Bridge Type" class="Enum (strict)"() -> ("Value"=w417:T61)  [unwired: 2 in, 2 out]
            n298 = case shown="\"AVS47A (GPIB interface)\"" w417 {
              tunnel: [w423 w432 w448 refnum<visa-resource-name> refnum ("dup VISA session") refnum<visa-resource-name> refnum ("dup VISA session")] -> w416
              tunnel: [w422 w435 _ w456 errorcluster {"status"=FALSE, "code"=0, "source"=""} ("error out")] -> w415
              tunnel: [_ _ w447 _ _] -> _
              tunnel: w412 -> [_ _ _ w453 _]
              tunnel: w411 -> [_ _ _ w452 _]
              frame "AVS47A (GPIB interface)" {
                # "Set default Parameters,\n enable Autoranging"
                n299 = property on="AVS GPIB Address" class="VISAName"() -> ("Value"=w418:refnum<visa-resource-name>)  [unwired: 2 in, 2 out]
                n300 = call "AVS47IB Initialize.vi"("Instr. Descriptor (GPIB::)"=w418) -> ("VISA session"=w431:refnum<visa-resource-name>, "error out"=w419:errorcluster)  [unwired: 13 in]
                n301 = call "AVS47IB Stop.vi"("VISA session"=w431, "error in (no error)"=w419) -> ("dup VISA session"=w429:refnum<visa-resource-name>, "error out"=w421:errorcluster)  [unwired: 12 in]
                n302 = call "AVS47IB Go Remote.vi"("VISA session"=w429, "error in (no error)"=w421) -> ("dup VISA session"=w430:refnum<visa-resource-name>, "error out"=w420:errorcluster)  [unwired: 12 in]
                n303 = call "AVS47IB Configure 47IB.vi"("VISA session"=w430, "Printer Enabled (-1:no change)"=i8 0, "Buffer Enabled (-1:no change)"=i8 0, "Message Headers Included  (-1:no change)"=i8 0, "Autoranging Enabled (-1:no change)"=i8 1, "Stabilisation Delay (-1:no change)"=i8 15, "error in (no error)"=w420) -> ("dup VISA session"=w423:refnum<visa-resource-name>, "error out"=w422:errorcluster)  [unwired: 7 in]
              }
              frame "AVS47B (RS232 interface)" {
                n304 = property on="Bridge settings" class="Clust (strict)"() -> ("Value"=w439:T35)  [unwired: 2 in, 2 out]
                n305 = Unbundle By Name(w439) -> ("AVS RS232 Port"=w438:refnum<visa-resource-name>)
                n306 = call "InitPort_b.vi"("VISA resource"=w438) -> ("error out"=w434:errorcluster, "dup VISA resource"=w437:refnum<visa-resource-name>)  [unwired: 5 in]
                n307 = Type Cast(type=refnum<visa-resource-name> refnum ("dup VISA session"), x=w437) -> (*(type *) &x=w433:refnum<visa-resource-name>)
                n308 = case shown="Error" w434 {
                  selector: w434 -> [w440 w443]
                  tunnel: w433 -> [w441 w445]
                  tunnel: [w440 w444] -> w435
                  tunnel: [w441 refnum<visa-resource-name> refnum ("dup VISA session")] -> w432
                  frame No Error {
                  }
                  frame Error {
                    n309 = VISA Close(VISA resource name=w445, error in (no error)=w443) -> (error out=w444:errorcluster)
                  }
                }
              }
              frame "AVS48SI (RS232 interface)" {
                n310 = property on="Bridge settings" class="Clust (strict)"() -> ("Value"=w451:T35)  [unwired: 2 in, 2 out]
                n311 = Unbundle By Name(w451) -> ("AVS RS232 Port"=w449:refnum<visa-resource-name>)
                n312 = call "Configure Hardware.vi"("VISA RESOURCE NAME"=w449) -> ("THREAD OUT"=w446:string)  [unwired: 14 in]
                n313 = call "Configure Sensor Wiring of CHs.vi"("THREAD IN"=w446) -> ("THREAD OUT"=w447:string)  [unwired: 10 in]
                n314 = Type Cast(type=refnum<visa-resource-name> refnum ("dup VISA session"), x=w449) -> (*(type *) &x=w448:refnum<visa-resource-name>)
              }
              frame "Impedance Bridge" {
                n315 = call "SetParFilePath.vi"("path"=w453, "zDll"=w452) -> ("error out"=w455:errorcluster, "zDll out"=w454:path)  [unwired: 8 in]
                n316 = call "StartScan.vi"("error in (no error)"=w455, "path in"=w454) -> ("error out"=w456:errorcluster)  [unwired: 8 in, 1 out]
              }
              frame "Disabled", Default {
              }
            }
            "_AVS_VISA" <- w416
            n317 = property on="Bridge status" class="Clust (strict)"("Value"=w415) -> ()  [unwired: 2 in, 2 out]
            n318 = property on="_ScanData" class="Arr (strict)"("Value"=dbl[] [0.0, 0.0, 0.0, 0.0, 0.0, 0.0, 0.0, 0.0, 0.0, 0.0] ("R_array")) -> ()  [unwired: 2 in, 2 out]
            n319 = call "ScanParameters FGV.vi"("Action"=Action."Init") -> ()  [unwired: 10 in, 1 out]
          }
          frame #5 {
            # "Generate paths for log files"
            n320 = Unbundle By Name("Data Logging Settings") -> ("Run Description"=w463:string, "Filenames Suffix"=w464:string, "Log Files Folder"=w461:path, "Log Files Name"=w467:string, "Automode Files Name"=w466:string)
            n321 = call "Create Dir if Non-Existant__ogtk.vi"("Directory Path"=w461) -> ("dup Directory Path"=w460:path)  [unwired: 8 in, 2 out]
            n322 = call "MGI Make String Filesafe.vi"("String In"=w463) -> ("Filesafe String Out"=w462:string)
            n323 = call "GeneratePaths.vi"("Filename Suffix"=w464, "Run description"=w462, "AVS_Path"=w460, "AVS_FName"=w467, "CAL_Path"=w460, "CAL_FName"=w466) -> ("Generated Log path"=w465:path, "Generated Calib path"=→"_CalibFilesPath":path)  [unwired: 8 in]
            n324 = property on="_LogFilesPath" class="Path"("Val(Sgnl)"=w465) -> ()  [unwired: 2 in, 2 out]
          }
          frame #6 {
            # "Start measurements"
            n325 = Set Occurrence(w470) -> ()
          }
        }
      }
      event "Stop": Value Change; Application Instance Close {
        # "\"Stop\" button pressed -> Stop measuring."
        n326 = event-data() -> ()  [unwired: 1 in, 1 out]
        n327 = flat-sequence {
          tunnel: w472 -> [w475]
          tunnel: w473 -> [w490]
          tunnel: w471 -> [w504]
          frame #0 {
            # "Save settings to config file"
            n328 = control-ref of="zBridge.Active Channels"() -> (w478:refnum<vi>)
            n329 = control-ref of="Bridge settings"() -> (w485:refnum<vi>)
            n330 = control-ref of="Runtime Settings"() -> (w484:refnum<vi>)
            n331 = control-ref of="CS Settings"() -> (w486:refnum<vi>)
            n332 = control-ref of="Data Logging Settings"() -> (w487:refnum<vi>)
            n333 = control-ref of="Sensor Calibrations"() -> (w483:refnum<vi>)
            n334 = control-ref of="PID Settings"() -> (w482:refnum<vi>)
            n335 = control-ref of="CS Cannel Names"() -> (w481:refnum<vi>)
            n336 = control-ref of="Channel names"() -> (w480:refnum<vi>)
            n337 = control-ref of="Curent Calibrations"() -> (w479:refnum<vi>)
            n338 = control-ref of="CS.Mode1.PID"() -> (w477:refnum<vi>)
            n339 = control-ref of="CS.Mode1.Settings"() -> (w476:refnum<vi>)
            n340 = Build Array(w478, w485, w484, w486, w487, w483, w482, w481, w480, w479, w477, w476) -> (w489:refnum<vi>[])
            n341 = call "Save Load Settings to File by Ref with path.vi"("Array of Cluster References"=w489, "Action"=enum8{"Load", "Save"}."Save", "Configuration file"=w475) -> ()  [unwired: 6 in, 1 out]
          }
          frame #1 {
            # "Free serial ports"
            n342 = control-ref of="_AVS_VISA"() -> (w491:refnum<vi>)
            n343 = control-ref of="TCS RS232 Port"() -> (w496:refnum<vi>)
            n344 = call "StopScan.vi"("path in"=w490) -> ()  [unwired: 9 in, 2 out]
            n345 = property class="VISAName"(reference=w491) -> (error out=w493:errorcluster, "Value"=w492:refnum<visa-resource-name>)  [unwired: 1 in, 1 out]
            n346 = property class="VISAName"(reference=w496) -> (error out=w494:errorcluster, "Value"=w495:refnum<visa-resource-name>)  [unwired: 1 in, 1 out]
            n347 = VISA Close(VISA resource name=w492, error in (no error)=w493) -> ()  [unwired: 1 out]
            n348 = VISA Close(VISA resource name=w495, error in (no error)=w494) -> ()  [unwired: 1 out]
          }
          frame #2 {
            w498 = u8 0 ("Disabled")
            # "Reset controls state"
            n349 = property on="Bridge Type" class="Enum (strict)"("Disabled"=w498) -> ()  [unwired: 2 in, 2 out]
            n350 = property on="AVS GPIB Address" class="VISAName"("Disabled"=w498) -> ()  [unwired: 2 in, 2 out]
            n351 = property on="AVS RS232 Port" class="VISAName"("Disabled"=w498) -> ()  [unwired: 2 in, 2 out]
            n352 = property on="TCS RS232 Port" class="VISAName"("Disabled"=w498) -> ()  [unwired: 2 in, 2 out]
            n353 = property on="CS type" class="Enum (strict)"("Disabled"=w498) -> ()  [unwired: 2 in, 2 out]
            n354 = property on="CS.QCS Device Nr" class="DigNum (strict)"("Disabled"=w498) -> ()  [unwired: 2 in, 2 out]
            n355 = property on="Start" class="Bool (strict)"("Visible"=TRUE, "Disabled"=u8 0, "Value"=FALSE ("start")) -> ()  [unwired: 2 in, 2 out]
            n356 = property on="Stop" class="Bool (strict)"("Value"=FALSE ("MainStopButton")) -> ()  [unwired: 2 in, 2 out]
          }
          frame #3 {
            w502 = u8 2 ("Disabled")
            # "Disable UI"
            n357 = property on="Top Toolbar" class="TabCtl (strict)"("Disabled"=w502) -> ()  [unwired: 2 in, 2 out]
            n358 = property on="Main Panel" class="TabCtl (strict)"("Disabled"=w502) -> ()  [unwired: 2 in, 2 out]
            n359 = property on="CS Indicators Panel" class="TabCtl (strict)"("Disabled"=w502) -> ()  [unwired: 2 in, 2 out]
            n360 = property on="Side Panel" class="TabCtl (strict)"("Disabled"=w502) -> ()  [unwired: 2 in, 2 out]
            n361 = property on="Lower Panel" class="TabCtl (strict)"("Disabled"=w502) -> ()  [unwired: 2 in, 2 out]
            n362 = property on="_String" class="Str"("Visible"=TRUE) -> ()  [unwired: 2 in, 2 out]
          }
          frame #4 {
            n363 = invoke class="App" method="Library.UndeployLibrary"("libPath"=w504) -> ()  [unwired: 4 in, 5 out]
          }
          frame #5 {
            # "Stop \nexecution"
            n364 = Stop(stop? (T)=TRUE) -> ()
          }
        }
        n365 = Unbundle By Name(w474) -> ("Variables Library"=w471:path, "zBridge dll"=w473:path, "Config File"=w472:path)
      }
      event "_ScanData": Value Change {
        # "Convert 8 elements AVS\narray to 10 elements"
        # "Received new data from AVS/zBridge. Do general tasks - update indicators, calculate temperature and pass the data further to AVS/zBridge specific processing"
        n366 = event-data() -> ("NewVal"=w522:dbl[])  [unwired: 1 in]
        n367 = Unbundle By Name(w510) -> ("UpdateValuesAVS"=w508:refnum<user-event>, "UpdateValuesZBridge"=w509:refnum<user-event>)
        n368 = Unbundle By Name(w506) -> ("Calibrations Folder"=w507:path)
        n369 = for {
          tunnel: w522 -> [w551] mode=indexing
          tunnel: [w549] -> w518 mode=indexing
          n370 = Less?(x=w551, y=1e+25) -> (x < y?=w552:bool)
          n371 = Select(t=w551, s=w552, f=inf) -> (s? t:f=w549:dbl)
        }
        n372 = Index Array(array=w518) -> (element #1=→"R0":dbl, element #2=→"R1":dbl, element #3=→"R2":dbl, element #4=→"R3":dbl, element #5=→"R4":dbl, element #6=→"R5":dbl, element #7=→"R6":dbl, element #8=→"R7":dbl, element #9=→"R8":dbl, element #10=→"R9":dbl)  [unwired: 10 in]
        n373 = Array To Cluster(array=w518) -> (cluster=w512:T62)
        "R Cluster" <- w512
        n374 = Cluster To Array(cluster=w512) -> (array=w511:dbl[])
        n375 = Absolute Value(x=w511) -> (abs(x)=w519:dbl[])
        n376 = property on="Allow neg R" class="Bool (strict)"() -> ("Value"=w517:bool)  [unwired: 2 in, 2 out]
        n377 = Select(t=w511, s=w517, f=w519) -> (s? t:f=w516:dbl[])
        "R Array" <- w516
        n378 = local read "_CurCalibrations"() -> (w524:T33)
        n379 = Cluster To Array(cluster=w524) -> (array=w523:string[])
        n380 = call "Resistance to Temp no Ext.vi"("error in"=w525, "Path"=w507, "CurCalibrations"=w523, "Resistance"=w516) -> ("Temperature"=w514:dbl[])  [unwired: 1 in, 3 out]
        "T Array" <- w514
        n381 = Array To Cluster(array=w514) -> (cluster=w530:T63)
        "T Cluster" <- w530
        n382 = Unbundle(w530) -> ("Temperature[0]"=→"T0":dbl, "Temperature[1]"=→"T1":dbl, "Temperature[2]"=→"T2":dbl, "Temperature[3]"=→"T3":dbl, "Temperature[4]"=→"T4":dbl, "Temperature[5]"=→"T5":dbl, "Temperature[6]"=→"T6":dbl, "Temperature[7]"=→"T7":dbl, "Temperature[8]"=→"T8":dbl, "Temperature[9]"=→"T9":dbl)
        n383 = property on="Mode Buttons" class="RadioBtnsControl (strict)"() -> ("Value"=w529:T7)  [unwired: 2 in, 2 out]
        n384 = Array To Cluster(array=w516) -> (cluster=w515:T62)
        n385 = Array To Cluster(array=w514) -> (cluster=w513:T63)
        n386 = case shown="\"No Selection\", Default" w529 {
          tunnel: w513 -> [w564 _]
          tunnel: w515 -> [w565 _]
          frame "No Selection", Default {
            n387 = call "Current Time(double).vi"() -> ("Current Time (double)"=→"Time":dbl)  [unwired: 6 in, 1 out]
            "Small R Cluster" <- w565
            "Small T Cluster" <- w564
          }
          frame "Cursor mode" {
          }
        }
        n388 = Bundle(w516, "Temperature"=w514) -> (w527:cluster{dbl[], "Temperature":dbl[]})  [unwired: 1 in]
        n389 = property on="Bridge Type" class="Enum (strict)"() -> ("Value"=w526:T61)  [unwired: 2 in, 2 out]
        n390 = case shown="\"AVS47B (RS232 interface)\", Default" w526 {
          tunnel: [w557 w558 w561] -> w528
          tunnel: w525 -> [w556 w558 w562]
          tunnel: w527 -> [w555 _ w560]
          tunnel: w509 -> [_ _ w559]
          tunnel: w508 -> [w554 _ _]
          frame "AVS47B (RS232 interface)", Default {
            n391 = Generate User Event(user event=w554, event data cluster=w555, error in=w556) -> (error out=w557:errorcluster)  [unwired: 1 in, 1 out]
          }
          frame "Disabled" {
          }
          frame "Impedance Bridge" {
            n392 = Generate User Event(user event=w559, event data cluster=w560, error in=w562) -> (error out=w561:errorcluster)  [unwired: 1 in, 1 out]
          }
        }
      }
      event User Event {
        # "Process data from the AVS bridge"
        n393 = event-data() -> ("R"=w570:dbl[], "T"=w569:dbl[])  [unwired: 1 in]
        n394 = property on="CS.Actual Current" class="Arr (strict)"() -> ("Value"=w571:dbl[])  [unwired: 2 in, 2 out]
        n395 = Unbundle By Name(w568) -> ("CS Automode"=w567:refnum<user-event>)
        n396 = stacked-sequence {
          tunnel: w573 -> [_ w597]
          tunnel: [_ w626] -> w572
          tunnel: w571 -> [_ w591]
          tunnel: w570 -> [w581 w593]
          tunnel: w569 -> [w580 w592]
          tunnel: w567 -> [w578 _]
          frame #0 {
            # "Filter data and add it to the data array. \nDo PID"
            n397 = property on="Runtime Settings" class="Clust (strict)"() -> ("Value"=w584:T27)  [unwired: 2 in, 2 out]
            n398 = Unbundle By Name(w584) -> ("Y_max"=w587:dbl, "Y_min"=w586:dbl, "Filter Graphs"=w585:bool)
            n399 = local read "Data Array"() -> (w582:T28)
            n400 = property on="Data Memory" class="DigNum (strict)"() -> ("Value"=w589:u16)  [unwired: 2 in, 2 out]
            n401 = call "Current Time(double).vi"() -> ("Current Time (double)"=w579:dbl)  [unwired: 6 in, 1 out]
            n402 = call "Manage Data Arrays - AVS.vi"("Y_max"=w587, "Y_min"=w586, "Filter Graph Results"=w585, "Append New Data"=TRUE, "Data In"=w582, "Curr R"=w581, "Curr T"=w580, "Curr Time"=w579, "Data Memory"=w589) -> ("Data Out"=w583:T28)  [unwired: 10 in]
            n403 = Bundle("Current Time (double)"=w579, "R"=w581, "T"=w580) -> (w590:T64)  [unwired: 1 in]
            n404 = local write "Data Array"(w583) -> ()
            n405 = Generate User Event(user event=w578, event data cluster=w590) -> ()  [unwired: 2 in, 2 out]
            n406 = Initialize Array("Ohm" ("AVS Name 0"), 10 ("dimension size")) -> (w577:string[])
            n407 = Array To Cluster(array=w577) -> (cluster=w574:T33)
            n408 = local write "Units"(w574) -> ()
          }
          frame #1 {
            # "Save data to log file"
            n409 = local read "_LogFilesPath"() -> (w624:path)
            n410 = local read "_CalibFilesPath"() -> (w625:path)
            n411 = call <vilib>:"Check if File or Folder Exists.vi"("path"=w624) -> ("file or folder exists?"=w616:bool, "dup path"=w617:path)  [unwired: 8 in, 1 out]
            n412 = case shown="False" w616 {
              tunnel: w617 -> [w649 w656]
              tunnel: [w649 w656] -> w618
              tunnel: [w647 _] -> w610
              frame False {
                n413 = control-ref of="Sensor Calibrations"() -> (w652:refnum<vi>)
                n414 = property on="Run Description" class="Str"() -> ("Value"=w648:string)  [unwired: 2 in, 2 out]
                n415 = Cluster To Array(cluster="Sensor Names") -> (array=w654:string[])
                n416 = Cluster To Array(cluster="CS Cannel Names") -> (array=w655:string[])
                n417 = call "Format log file header Z.vi"("Thermometer"=w652, "AVS names"=w654, "CS Names"=w655, "Run description"=w648) -> ("String"=w650:string)  [unwired: 1 in]
                n418 = Write to Text File(file (use dialog)=w649, text=w650) -> (error out=w647:errorcluster)  [unwired: 2 in, 2 out]
              }
              frame True {
              }
            }
            n419 = property on="Data Logging Settings" class="Clust (strict)"() -> ("Value"=w635:T37)  [unwired: 2 in, 2 out]
            n420 = Unbundle By Name(w635) -> ("Delimeter"=w608:string, "Date Format"=w634:string)
            n421 = call "Current Time(double).vi"() -> ("Current Time"=w611:timestamp, "Current Time (double)"=w612:dbl)  [unwired: 6 in]
            n422 = call "File Info__ogtk.vi"("error in (no error)"=w610, "file"=w618) -> ("error out"=w609:errorcluster, "file info"=w614:T65, "file out"=w623:path)  [unwired: 4 in]
            n423 = Unbundle By Name(w614) -> ("creation date"=w615:u32)
            n424 = Number To Exponential String(number=w612, precision (6)=i16 10) -> (E-format string=w606:string)  [unwired: 2 in]
            n425 = Format Date/Time String(time format string (%c)=w634, seconds (now)=w611) -> (date/time string=w631:string)  [unwired: 1 in]
            n426 = Number To Fractional String(number=w593) -> (F-format string=w633:string[])  [unwired: 3 in]
            n427 = Number To Fractional String(number=w592) -> (F-format string=w632:string[])  [unwired: 3 in]
            n428 = Number To Fractional String(number=w591) -> (F-format string=w630:string[])  [unwired: 3 in]
            n429 = property on="New File Interval" class="DigNum (strict)"() -> ("Value"=w619:u32)  [unwired: 2 in, 2 out]
            n430 = property on="New File Interval Units" class="Enum (strict)"() -> ("Value"=w620:enum16{"Minutes", "Hours", "Days"})  [unwired: 2 in, 2 out]
            n431 = To Time Stamp(1:w615) -> (0:w621:timestamp)
            n432 = Build Array (concatenate)(w631, w606, w633, w632, w630) -> (w607:string[])
            n433 = call "Time Elapsed time.vi"("Time Units"=w620, "Delay Time"=w619, "Time Old In"=w621) -> ("T>dT?"=w622:bool)  [unwired: 2 out]
            n434 = local read "Bridge settings"() -> (w598:T35)
            n435 = case shown="True" w622 {
              tunnel: [w637 w640] -> w613
              tunnel: [w636 w641] -> _
              tunnel: w623 -> [w637 _]
              tunnel: w625 -> [w636 _]
              frame False {
              }
              frame True {
                n436 = local read "Data Logging Settings"() -> (w642:T37)
                n437 = Unbundle By Name(w642) -> ("Run Description"=w638:string, "Log Files Folder"=w646:path, "Log Files Name"=w644:string, "Automode Files Name"=w645:string, "Filenames Suffix"=w643:string)
                n438 = call "MGI Make String Filesafe.vi"("String In"=w638) -> ("Filesafe String Out"=w639:string)
                n439 = call "GeneratePaths.vi"("Filename Suffix"=w643, "Run description"=w639, "AVS_Path"=w646, "AVS_FName"=w644, "CAL_Path"=w646, "CAL_FName"=w645) -> ("Generated Log path"=w640:path, "Generated Calib path"=w641:path)  [unwired: 8 in]
                n440 = local write "_CalibFilesPath"(w641) -> ()
                n441 = property on="_LogFilesPath" class="Path"("Val(Sgnl)"=w640) -> ()  [unwired: 2 in, 2 out]
              }
            }
            n442 = local read "Sensor Names"() -> (w594:T10)
            n443 = Unbundle By Name(w598) -> ("Bridge Type"=w601:T61)
            n444 = property on="Sensor Calibrations" class="Clust (strict)"() -> ("Controls[]"=w595:refnum<vi>[])  [unwired: 2 in, 2 out]
            n445 = To Unsigned Long Integer(number=w601) -> (unsigned 32bit integer=w602:u32)
            n446 = Variant To Data(error in=w597, type=T54."AVS47A (GPIB interface)" ("AVS type"), Variant=w602) -> (data=w600:T54, error out=w596:errorcluster)
            n447 = Bundle By Name(cluster=T55 {"R"=[], "T"=[], "I"=[], "AVS type"=enum."AVS47A (GPIB interface)", "AVS names"={"AVS Name 0"="", "AVS Name 1"="", "AVS Name 2"="", "AVS Name 3"="", "AVS Name 4"="", "AVS Name 5"="", "AVS Name 6"="", "AVS Name 7"="", "AVS Name 8"="", "AVS Name 9"=""}, "Calibration"=[]} ("TC Cluster"), "Calibration"=w595, "AVS names"=w594, "R"=w593, "T"=w592, "I"=w591, "AVS type"=w600) -> (w605:T55)
            n448 = call "TC_to_DSC.vi"("error in (no error)"=w596, "TC Cluster"=w605) -> ("error out"=w604:errorcluster)  [unwired: 9 in]
            n449 = call "Write To Spreadsheet File (string) w Error.vi"("delimiter (\\t)"=w608, "append to file? (new file:F)"=TRUE, "error in"=w609, "1D data"=w607, "file path (dialog if empty)"=w613) -> ("error out"=w627:errorcluster)  [unwired: 5 in, 1 out]
            n450 = Merge Errors(w627, w604) -> (w626:errorcluster)
          }
        }
      }
      event User Event {
        # "Process data from the zBridge bridge"
        n451 = event-data() -> ("R"=w666:dbl[], "T"=w665:dbl[])  [unwired: 1 in]
        n452 = property on="CS.Actual Current" class="Arr (strict)"() -> ("Value"=w664:dbl[])  [unwired: 2 in, 2 out]
        n453 = local read "_zBridgeParText"() -> (w661:string)
        n454 = local read "_zBridgeSetNr"() -> (w667:u8)
        n455 = local read "_ZBridgeUnit"() -> (w662:string)
        n456 = Unbundle By Name(w660) -> ("CS Automode"=w659:refnum<user-event>)
        n457 = stacked-sequence {
          tunnel: w661 -> [w688 _]
          tunnel: w667 -> [w673 w696]
          tunnel: w666 -> [w671 w722]
          tunnel: w665 -> [w670 w721]
          tunnel: w664 -> [_ w720]
          tunnel: w663 -> [_ w719]
          tunnel: [_ w718] -> w658
          tunnel: w662 -> [w675 _]
          tunnel: w659 -> [w672 _]
          frame #0 {
            # "Only do PID after measuring\non selected channel( or any \nchannel if -1 is selected)"
            n458 = local read "zBridge params"() -> (w674:T19)
            n459 = local read "Units"() -> (w676:T13)
            n460 = Cluster To Array(cluster=w676) -> (array=w679:string[])
            n461 = Cluster To Array(cluster=w674) -> (array=w689:string[])
            n462 = Replace Array Subset(array=w679, new element=w675, index=w673) -> (w678:string[])
            n463 = Replace Array Subset(array=w689, new element=w688, index=w673) -> (w690:string[])
            n464 = Array To Cluster(array=w678) -> (cluster=→"Units":T66)
            n465 = Array To Cluster(array=w690) -> (cluster=→"zBridge params":T67)
            n466 = property on="Runtime Settings" class="Clust (strict)"() -> ("Value"=w682:T27)  [unwired: 2 in, 2 out]
            n467 = Unbundle By Name(w682) -> ("Y_max"=w685:dbl, "Y_min"=w684:dbl, "Filter Graphs"=w683:bool)
            n468 = local read "Data Array"() -> (w680:T28)
            n469 = property on="Data Memory" class="DigNum (strict)"() -> ("Value"=w687:u16)  [unwired: 2 in, 2 out]
            n470 = call "Current Time(double).vi"() -> ("Current Time (double)"=w668:dbl)  [unwired: 6 in, 1 out]
            n471 = call "Manage Data Arrays - zBridge.vi"("Y_max"=w685, "Y_min"=w684, "Filter Graph Results"=w683, "Append New Data"=TRUE, "Data In"=w680, "Curr R"=w671, "Curr T"=w670, "Curr Time"=w668, "Channel"=w673, "Data Memory"=w687) -> ("Data Out"=w681:T28)  [unwired: 9 in]
            n472 = local write "Data Array"(w681) -> ()
            n473 = Bundle("Current Time (double)"=w668, "R"=w671, "T"=w670) -> (w669:T64)  [unwired: 1 in]
            n474 = Generate User Event(user event=w672, event data cluster=w669) -> ()  [unwired: 2 in, 2 out]
          }
          frame #1 {
            n475 = local read "_LogFilesPath"() -> (w699:path)
            n476 = local read "Data Logging Settings"() -> (w717:T37)
            n477 = call "Strip Path Extension - Path__ogtk.vi"("path"=w699) -> ("root"=w700:string, "extension"=w703:string)
            n478 = Format Into String(format string="_%d", initial string=w700, w696) -> (resulting string=w701:string)  [unwired: 1 in, 1 out]
            n479 = Concatenate Strings(w701, "." ("string"), w703) -> (w698:string)
            n480 = Unbundle By Name(w717) -> ("Delimeter"=w733:string, "Date Format"=w732:string)
            n481 = String To Path(string=w698) -> (path=w697:path)
            n482 = call <vilib>:"Check if File or Folder Exists.vi"("path"=w697) -> ("file or folder exists?"=w708:bool, "dup path"=w709:path)  [unwired: 8 in, 1 out]
            n483 = case shown="False" w708 {
              tunnel: w709 -> [w751 w754]
              tunnel: [w751 w754] -> w710
              tunnel: [w745 _] -> w693
              frame False {
                n484 = local read "CS Cannel Names"() -> (w749:T31)
                n485 = local read "Sensor Names"() -> (w750:T10)
                n486 = control-ref of="Sensor Calibrations"() -> (w753:refnum<vi>)
                n487 = property on="Run Description" class="Str"() -> ("Value"=w746:string)  [unwired: 2 in, 2 out]
                n488 = Cluster To Array(cluster=w750) -> (array=w747:string[])
                n489 = Cluster To Array(cluster=w749) -> (array=w748:string[])
                n490 = call "Format log file header Z.vi"("Thermometer"=w753, "AVS names"=w747, "CS Names"=w748, "Run description"=w746) -> ("String"=w752:string)  [unwired: 1 in]
                n491 = Write to Text File(file (use dialog)=w751, text=w752) -> (error out=w745:errorcluster)  [unwired: 2 in, 2 out]
              }
              frame True {
              }
            }
            n492 = call "Current Time(double).vi"() -> ("Current Time"=w694:timestamp, "Current Time (double)"=w695:dbl)  [unwired: 6 in]
            n493 = Number To Exponential String(number=w695, precision (6)=i16 10) -> (E-format string=w725:string)  [unwired: 2 in]
            n494 = Format Date/Time String(time format string (%c)=w732, seconds (now)=w694) -> (date/time string=w729:string)  [unwired: 1 in]
            n495 = Number To Exponential String(number=w722) -> (E-format string=w731:string[])  [unwired: 3 in]
            n496 = Number To Engineering String(4:w721) -> (0:w730:string[])  [unwired: 3 in]
            n497 = Number To Fractional String(number=w720) -> (F-format string=w728:string[])  [unwired: 3 in]
            n498 = call "File Info__ogtk.vi"("error in (no error)"=w693, "file"=w710) -> ("error out"=w692:errorcluster, "file info"=w706:T65, "file out"=w715:path)  [unwired: 4 in]
            n499 = Unbundle By Name(w706) -> ("creation date"=w707:u32)
            n500 = Build Array (concatenate)(w729, w725, w731, w730, w728) -> (w727:string[])
            n501 = local read "_CalibFilesPath"() -> (w716:path)
            n502 = property on="New File Interval" class="DigNum (strict)"() -> ("Value"=w711:u32)  [unwired: 2 in, 2 out]
            n503 = property on="New File Interval Units" class="Enum (strict)"() -> ("Value"=w712:enum16{"Minutes", "Hours", "Days"})  [unwired: 2 in, 2 out]
            n504 = To Time Stamp(1:w707) -> (0:w713:timestamp)
            n505 = call "Time Elapsed time.vi"("Time Units"=w712, "Delay Time"=w711, "Time Old In"=w713) -> ("T>dT?"=w714:bool)  [unwired: 2 out]
            n506 = case shown="True" w714 {
              tunnel: [w735 w738] -> w705
              tunnel: [w734 w740] -> _
              tunnel: w715 -> [w735 _]
              tunnel: w716 -> [w734 _]
              frame False {
              }
              frame True {
                n507 = local read "Data Logging Settings"() -> (w741:T37)
                n508 = Unbundle By Name(w741) -> ("Run Description"=w737:string, "Filenames Suffix"=w739:string, "Log Files Folder"=w744:path, "Log Files Name"=w742:string, "Automode Files Name"=w743:string)
                n509 = call "MGI Make String Filesafe.vi"("String In"=w737) -> ("Filesafe String Out"=w736:string)
                n510 = call "GeneratePaths.vi"("Filename Suffix"=w739, "Run description"=w736, "AVS_Path"=w744, "AVS_FName"=w742, "CAL_Path"=w744, "CAL_FName"=w743) -> ("Generated Log path"=w738:path, "Generated Calib path"=w740:path)  [unwired: 8 in]
                n511 = local write "_CalibFilesPath"(w740) -> ()
                n512 = property on="_LogFilesPath" class="Path"("Val(Sgnl)"=w738) -> ()  [unwired: 2 in, 2 out]
              }
            }
            n513 = call "Write To Spreadsheet File (string) w Error.vi"("delimiter (\\t)"=w733, "append to file? (new file:F)"=TRUE, "error in"=w692, "1D data"=w727, "file path (dialog if empty)"=w705) -> ("error out"=w723:errorcluster)  [unwired: 5 in, 1 out]
            n514 = Merge Errors(w723, w719) -> (w718:errorcluster)
          }
        }
      }
      event User Event {
        # "Current source automatic mode"
        n515 = event-data() -> ("R"=w761:dbl[], "T"=w762:dbl[], "Time"=w756:dbl)  [unwired: 1 in, 4 out]
        n516 = local read "CS.Mode"() -> (w760:T39)
        n517 = Unbundle By Name(w759) -> ("CallExtVI"=w758:refnum<user-event>, "TempStabilized"=w757:refnum<user-event>)
        n518 = case shown="\"Mode2\"" w760 {
          tunnel: w762 -> [_ w766 w841]
          tunnel: w761 -> [_ w767 w842]
          tunnel: w758 -> [_ w769 _]
          tunnel: w757 -> [_ w768 _]
          tunnel: w756 -> [_ w765 _]
          frame "Manual", Default {
          }
          frame "Mode 1" {
            n519 = call "MGI Change Detector (T).vi"("Value"="CS.Mode1.Start") -> ("Changed?"=w763:bool)
            n520 = case shown="True" "CS.Mode1.Start" {
              tunnel: w769 -> [_ w782]
              tunnel: w768 -> [_ w781]
              tunnel: w767 -> [_ w780]
              tunnel: w766 -> [_ w779]
              tunnel: w765 -> [_ w776]
              tunnel: w763 -> [_ w770]
              frame False {
              }
              frame True {
                # "Check if PID error (SP-PV)==0"
                # "Check if temperature\nis stabilized"
                # "T sabilized?"
                # "If TCS auto mode enabled and temperature is not changing => fire TempStabilized event to save log and set new CS point. Otherwise do PID (if enabled)."
                # "Check if stabilization delay time \nis elapsed"
                n521 = property on="R/T?" class="Enum (strict)"() -> ("Value"=w778:enum16{"Resistance", "Temperature"})  [unwired: 2 in, 2 out]
                n522 = case shown="\"Temperature\"" w778 {
                  tunnel: [w797 w798] -> w775
                  tunnel: w780 -> [w797 _]
                  tunnel: w779 -> [_ w798]
                  frame "Resistance", Default {
                  }
                  frame "Temperature" {
                  }
                }
                n523 = property on="Bridge Channel" class="DigNum (strict)"() -> ("Value"=w774:i32)  [unwired: 2 in, 2 out]
                n524 = Index Array(array=w775, index=w774) -> (element=w773:dbl)
                n525 = local read "CS.Mode1.PID Error"() -> (w789:dbl)
                n526 = property on="FB on 2" class="Enum (strict)"() -> ("Value"=w771:enum16{"0", "1", "2", "3"})  [unwired: 2 in, 2 out]
                n527 = local read "_CSMode1List[i]"() -> (w783:T23[])
                n528 = local read "_TimeOld"() -> (w795:dbl)
                n529 = property on="Delay Time" class="DigNum (strict)"() -> ("Value"=w785:dbl)  [unwired: 2 in, 2 out]
                n530 = property on="N averages" class="DigNum (strict)"() -> ("Value"=w772:i32)  [unwired: 2 in, 2 out]
                n531 = property on="T stability" class="DigNum (strict)"() -> ("Value"=w784:dbl)  [unwired: 2 in, 2 out]
                n532 = Equal To 0?(x=w789) -> (x = 0?=w787:bool)
                n533 = call "Derivatives Pt by Pt.vi"("initialize"=w770, "accuracy (%)"=w784, "Time"=w776, "Data"=w773, "Points to avg"=w772) -> ("Stable?"=w788:bool, "Stability (%)"=→"CS.Mode1.Slope":dbl, "dt (s)"=w792:dbl)  [unwired: 2 in]
                n534 = Index Array(array=w783, index=w771) -> (element=w796:T23)
                n535 = call "Time Elapsed dbl.vi"("Delay Time"=w785, "Time Old In"=w795) -> ("T>dT?"=w777:bool, "Delta T"=→"CS.Mode1.Timer":dbl, "Time New Out"=w794:dbl)  [unwired: 1 in]
                n536 = Compound Arithmetic op=AND(w777, w787, w788) -> (w790:bool)
                "CS.Mode1.PID Stabilized?" <- w790
                n537 = property on="Enable PID" class="Bool (strict)"() -> ("Value"=w786:bool)  [unwired: 2 in, 2 out]
                n538 = case shown="False" w790 {
                  tunnel: w794 -> [_ w818]
                  tunnel: w792 -> [w814 _]
                  tunnel: w786 -> [w804 _]
                  tunnel: w796 -> [w812 _]
                  tunnel: w783 -> [w809 _]
                  tunnel: w771 -> [w802 _]
                  tunnel: w782 -> [_ w816]
                  tunnel: w781 -> [_ w815]
                  tunnel: w773 -> [w801 _]
                  tunnel: w770 -> [w799 _]
                  frame False {
                    # "Temperature is not stable. If enabled, do PID regulation"
                    n539 = local read "CS.Current Value"() -> (w806:dbl[])
                    n540 = Index Array(array=w806, index=w802) -> (element=w807:dbl)
                    n541 = Multiply(x=1000.0, y=w807) -> (x*y=w805:dbl)
                    n542 = call "PID control incremental.vi"("Process Variable"=w801, "dt"=w814, "Setpoint"=w812, "PID Settings"="CS.Mode1.PID Settings", "I in"=w805, "PID Enabled"=w804, "Reset"=w799) -> ("PID output I"=→"Waveform Chart":T22, "err out"=→"CS.Mode1.PID Error":dbl, "I out"=w811:dbl)  [unwired: 9 in, 1 out]
                    n543 = Replace Array Subset(array=w809, new element=w811, index=w802) -> (→"CS.Automode Current":T23[])
                  }
                  frame True {
                    # "Temperature is stable & automode is on"
                    n544 = case shown="False" "CS.Mode1.Call VI?" {
                      tunnel: w818 -> [w821 _]
                      tunnel: w816 -> [_ w822]
                      tunnel: w815 -> [w819 _]
                      frame False {
                        # "External VI call disabled -> proceed\nwith automode"
                        n545 = local write "_TimeOld"(w821) -> ()
                        n546 = Generate User Event(user event=w819, event data cluster=TRUE ("event data")) -> ()  [unwired: 2 in, 2 out]
                      }
                      frame True {
                        # "Call external VI"
                        n547 = Generate User Event(user event=w822, event data cluster="" ("event data")) -> ()  [unwired: 2 in, 2 out]
                      }
                    }
                  }
                }
              }
            }
          }
          frame "Mode2" {
            n548 = Unbundle By Name("CS.Mode2.Settings") -> ("Hysteresis"=w824:u8, "Bridge Channel"=w825:i32, "FB on"=w826:enum16{"Resistance", "Temperature"})
            n549 = case shown="\"Resistance\", Default" w826 {
              tunnel: [w844 w845] -> w840
              tunnel: w842 -> [w844 _]
              tunnel: w841 -> [_ w845]
              frame "Resistance", Default {
              }
              frame "Temperature" {
              }
            }
            n550 = Index Array(array=w840, index=w825) -> (element=w839:dbl)
            n551 = local read "CS.Mode2.List"() -> (w838:dbl[][])
            n552 = call "Currents-Temp list  - T in range-.vi"("List in"=w838, "T"=w839, "T1 index"=1, "T0 index"=0, "Hysteresis"=w824) -> ("List index"=w832:i32, "I_out"=w831:dbl[])  [unwired: 1 out]
            n553 = case shown="True" "CS.Mode2.Start" {
              tunnel: w831 -> [_ w843]
              frame False {
              }
              frame True {
                n554 = local write "CS.Automode Current"(w843) -> ()
              }
            }
            n555 = Initialize Array(FALSE, 16 ("dimension size")) -> (w835:bool[])
            n556 = Replace Array Subset(array=w835, new element=TRUE ("new element/subarray"), index=w832) -> (→"CS.Mode2.Row":bool[])
          }
        }
      }
      event User Event {
        n557 = event-data() -> ()  [unwired: 1 in, 5 out]
        n558 = Unbundle By Name(w848) -> ("TempStabilized"=w847:refnum<user-event>)
        n559 = local read "_ExtVIReference"() -> (w852:refnum<vi>)
        n560 = call "GetExtVIStatus.vi"("vi reference in"=w852) -> ("vi reference out"=w849:refnum<vi>, "Exec.State"=w851:T46, "Finished?"=w850:bool)
        n561 = case shown="\"Idle\"" w851 {
          tunnel: w850 -> [_ _]
          tunnel: w849 -> [_ w854]
          tunnel: w847 -> [_ w853]
          frame "Bad", Default {
          }
          frame "Idle" {
            n562 = local read "VI called?"() -> (w855:bool)
            n563 = case shown="False" w855 {
              tunnel: w854 -> [w857 _]
              tunnel: w853 -> [_ w864]
              frame False {
                n564 = property on="_ScanData" class="Arr (strict)"() -> ("Value"=w860:dbl[])  [unwired: 2 in, 2 out]
                n565 = property on="T Array" class="Arr (strict)"() -> ("Value"=w861:dbl[])  [unwired: 2 in, 2 out]
                n566 = property on="CS.Current Value" class="Arr (strict)"() -> ("Value"=w862:dbl[])  [unwired: 2 in, 2 out]
                n567 = Format Date/Time String() -> (date/time string=w859:string)  [unwired: 3 in]
                n568 = Bundle("date/time string"=w859, "Value"=w860, "Value"=w861, "Value"=w862) -> (w858:T68)  [unwired: 1 in]
                n569 = call "CallExtVI.vi"("vi reference in"=w857, "Cluster"=w858) -> ()  [unwired: 1 out]
                "VI called?" <- TRUE ("VI called?")
              }
              frame True {
                n570 = call "Current Time(double).vi"() -> ("Current Time (double)"=w863:dbl)  [unwired: 6 in, 1 out]
                n571 = Generate User Event(user event=w864, event data cluster=TRUE ("event data")) -> ()  [unwired: 2 in, 2 out]
                n572 = local write "_TimeOld"(w863) -> ()
              }
            }
          }
        }
      }
      event User Event {
        # "CS automode\nT is stabilized"
        n573 = event-data() -> ("TempStabilized"=w868:bool)  [unwired: 1 in, 4 out]
        n574 = stacked-sequence {
          tunnel: w869 -> [w875 _]
          tunnel: [w876 _] -> w867
          tunnel: w868 -> [_ w896]
          frame #0 {
            # "Step1: Save R,T,I values to calibration file. Make screenshot when creating the calibration file."
            n575 = property on="_CalibFilesPath" class="Path"() -> ("Value"=w871:path)  [unwired: 2 in, 2 out]
            n576 = call "File Exists - Scalar__ogtk.vi"("file path"=w871) -> ("exists"=w872:bool)  [unwired: 6 in, 1 out]
            n577 = case shown="False" w872 {
              tunnel: w871 -> [w885 w895]
              tunnel: [w885 w895] -> w870
              frame False {
                n578 = local read "CS Cannel Names"() -> (w891:T31)
                n579 = local read "Sensor Names"() -> (w892:T10)
                n580 = property on="Run Description" class="Str"() -> ("Value"=w888:string)  [unwired: 2 in, 2 out]
                n581 = control-ref of="Sensor Calibrations"() -> (w894:refnum<vi>)
                n582 = Cluster To Array(cluster=w892) -> (array=w889:string[])
                n583 = Cluster To Array(cluster=w891) -> (array=w890:string[])
                n584 = call "Format log file header Z.vi"("Thermometer"=w894, "AVS names"=w889, "CS Names"=w890, "Run description"=w888) -> ("String"=w893:string)  [unwired: 1 in]
                n585 = control-ref of="This VI"() -> (w887:refnum<vi>)
                n586 = Write to Text File(file (use dialog)=w885, text=w893) -> ()  [unwired: 2 in, 3 out]
                n587 = invoke class="VI" method="FP.Get Image"(reference=w887) -> ("image data"=w886:T69)  [unwired: 5 in, 5 out]
                n588 = call "Convert File Extension (Path)__ogtk.vi"("new ending (none)"="png" ("name or relative path"), "file name"=w885) -> ("new filename"=w884:path)  [unwired: 1 out]
                n589 = call <vilib>:"Write PNG File.vi"("image data"=w886, "path to PNG file"=w884) -> ()  [unwired: 8 in, 2 out]
              }
              frame True {
              }
            }
            n590 = local write "VI called?"(FALSE ("VI called?")) -> ()
            n591 = property on="Data Logging Settings" class="Clust (strict)"() -> ("Value"=w879:T37)  [unwired: 2 in, 2 out]
            n592 = Unbundle By Name(w879) -> ("Date Format"=w880:string, "Delimeter"=w877:string)
            n593 = property on="R" class="Clust (strict)"() -> ("Value"=w878:T14)  [unwired: 2 in, 2 out]
            n594 = property on="T" class="Clust (strict)"() -> ("Value"=w882:T9)  [unwired: 2 in, 2 out]
            n595 = property on="CS.Current Value" class="Arr (strict)"() -> ("Value"=w881:dbl[])  [unwired: 2 in, 2 out]
            n596 = call "Write to cal log file.vi"("Value 2"=w881, "Date/Time Format"=w880, "Value 3"=w882, "Value"=w878, "Delimeter"=w877, "Value 4"=w870) -> ("error out"=w874:errorcluster)  [unwired: 1 out]
            n597 = Merge Errors(w874, w875) -> (w876:errorcluster)
          }
          frame #1 {
            # "Step 2: Sweep through the currents list"
            n598 = case shown="True" w896 {
              frame False {
              }
              frame True {
                n599 = local read "CS.Mode1.List:Count"() -> (w898:i32)
                n600 = local read "CS.Mode1.List:Index"() -> (w899:i32)
                n601 = Less?(x=w899, y=w898) -> (x < y?=w897:bool)
                n602 = case shown="False" w897 {
                  frame False {
                    n603 = property on="CS Mode" class="Enum (strict)"("Val(Sgnl)"=CS_mode."Manual" ("CS Mode")) -> ()  [unwired: 2 in, 2 out]
                  }
                  frame True {
                    n604 = property on="CS.Mode1.List:Next" class="Bool (strict)"("Val(Sgnl)"=TRUE) -> ()  [unwired: 2 in, 2 out]
                  }
                }
              }
            }
          }
        }
      }
      event User Event {
        # "Disable controls for disabled channels"
        n605 = event-data() -> ()  [unwired: 1 in, 5 out]
        n606 = Unbundle By Name(w903) -> ("zBridge dll"=w902:path)
        n607 = property on="Bridge Type" class="Enum (strict)"() -> ("Value"=w911:T61)  [unwired: 2 in, 2 out]
        n608 = case shown="Default" w911 {
          tunnel: [w921 w933 w941] -> w910
          tunnel: w902 -> [_ w932 _]
          frame Default {
            n609 = property on="Runtime Settings" class="Clust (strict)"() -> ("Value"=w925:T27)  [unwired: 2 in, 2 out]
            n610 = Unbundle By Name(w925) -> ("Read AVS channels from"=w923:i8, "Last Channel"=w924:i8)
            n611 = for {
              N: 10 -> [_]
              tunnel: w924 -> [w927]
              tunnel: w923 -> [w928]
              tunnel: [w926] -> w921 mode=indexing
              i -> [w929]
              n612 = Less Or Equal?(x=w928, y=w929) -> (x <= y?=w931:bool)
              n613 = Less Or Equal?(x=w929, y=w927) -> (x <= y?=w930:bool)
              n614 = And(x=w931, y=w930) -> (x .and. y?=w926:bool)
            }
          }
          frame "Impedance Bridge" {
            n615 = for {
              N: 10 -> [_]
              tunnel: [w936] -> w934 mode=indexing
              tunnel: w932 -> [w937]
              i -> [w939]
              n616 = call "GetByteParam.vi"("ParNo"=u8 0, "SetNo"=w939, "zDll"=w937) -> ("return type"=w936:u8)  [unwired: 6 in, 2 out]
            }
            n617 = Greater Than 0?(x=w934) -> (x > 0?=w933:bool[])
          }
          frame "AVS47B (RS232 interface)" {
            n618 = local read "zBridge.Active Channels"() -> (w940:T21)
            n619 = Cluster To Array(cluster=w940) -> (array=w941:bool[])
          }
        }
        n620 = control-ref of="zBridge.Active Channels"() -> (w917:refnum<vi>)
        n621 = control-ref of="AVS Exc&Ranges"() -> (w913:refnum<vi>)
        n622 = control-ref of="R"() -> (w918:refnum<vi>)
        n623 = control-ref of="Sensor Calibrations"() -> (w919:refnum<vi>)
        n624 = control-ref of="T"() -> (w920:refnum<vi>)
        n625 = control-ref of="uPlots"() -> (w914:refnum<vi>)
        n626 = control-ref of="AVS names"() -> (w912:refnum<vi>)
        n627 = control-ref of="zBridge params"() -> (w909:refnum<vi>)
        n628 = control-ref of="zBridge.Scan Phase"() -> (w908:refnum<vi>)
        n629 = control-ref of="Units"() -> (w907:refnum<vi>)
        n630 = control-ref of="AVS names small"() -> (w906:refnum<vi>)
        n631 = control-ref of="Small R Cluster"() -> (w905:refnum<vi>)
        n632 = control-ref of="Small T Cluster"() -> (w904:refnum<vi>)
        n633 = Build Array(w917, w913, w918, w919, w920, w914, w912, w909, w908, w907, w906, w905, w904) -> (w915:refnum<vi>[])
        n634 = Array Size(array=w915) -> (size(s)=w916:i32)
        n635 = for {
          N: w916 -> [_]
          tunnel: w915 -> [w945] mode=indexing
          tunnel: w910 -> [w942]
          n636 = property class="Clust"(reference=w945) -> ("Controls[]"=w943:refnum<vi>[])  [unwired: 1 in, 2 out]
          n637 = Array Size(array=w943) -> (size(s)=w944:i32)
          n638 = for {
            N: w944 -> [_]
            tunnel: w943 -> [w947] mode=indexing
            tunnel: w942 -> [w946] mode=indexing
            n639 = case shown="True" w946 {
              tunnel: w947 -> [w948 w953]
              frame False {
                n640 = property class="Ctl"(reference=w948, "Disabled"=u8 2) -> ("ClassName"=w949:string)  [unwired: 1 in, 2 out]
                n641 = case shown="\"Boolean\"" w949 {
                  tunnel: w948 -> [_ w952 _]
                  frame "False", Default {
                  }
                  frame "Boolean" {
                    n642 = property class="Ctl"(reference=w952, "Value"=FALSE) -> ()  [unwired: 1 in, 2 out]
                  }
                  frame "Ring" {
                  }
                }
              }
              frame True {
                n643 = property class="Ctl"(reference=w953, "Disabled"=u8 0) -> ("ClassName"=w954:string)  [unwired: 1 in, 2 out]
                n644 = case shown="\"False\", Default" w954 {
                  tunnel: w953 -> [_ w957]
                  frame "False", Default {
                  }
                  frame "Boolean" {
                    n645 = property class="Ctl"(reference=w957, "Value"=TRUE) -> ()  [unwired: 1 in, 2 out]
                  }
                }
              }
            }
          }
        }
      }
      event Mouse Down? {
        n646 = event-data() -> ("CtlRef"=w959:refnum<vi>, "Mods.Double Click"=w958:bool)  [unwired: 1 in]
        n647 = disable-structure shown="Enabled" {
          disable-tunnel: w958 -> [w962 _]
          disable-tunnel: w959 -> [w961 _]
          frame Enabled {
            n648 = case shown="True" w962 {
              tunnel: w961 -> [_ w981]
              frame False {
              }
              frame True {
                w977 = 128  # call and forget
                n649 = property class="Ctl"(reference=w981) -> ("Label.Text"=w980:string)  [unwired: 1 in, 2 out]
                n650 = local read "Sensor Names"() -> (w968:T10)
                n651 = call "Slice String 1__ogtk.vi"("Subset (i:j)"="-1", "String"=w980) -> ("Substring (String[i:j])"=w978:string)  [unwired: 7 in]
                n652 = Decimal String To Number(string=w978) -> (number=w963:i32)  [unwired: 2 in, 1 out]
                n653 = Cluster To Array(cluster=w968) -> (array=w967:string[])
                n654 = Index Array(array=w967, index=w963) -> (element=w966:string)
                n655 = vi-ref "Text Popup.vi"() -> (w974:refnum<vi>)
                n656 = property class="VI"(reference=w974) -> (error out=w975:errorcluster, "Name"=w976:string)  [unwired: 1 in, 1 out]
                n657 = Open VI Reference(type specifier VI Refnum (for type only)=refnum<vi> refnum, vi path=w976, options=w977, error in (no error)=w975) -> (vi reference=w973:refnum<vi>, error out=w970:errorcluster)  [unwired: 2 in]
                n658 = control-ref of="T Array"() -> (w964:refnum<vi>)
                n659 = control-ref of="R Array"() -> (w965:refnum<vi>)
                n660 = call-by-ref "Start Asynchronous Call"(reference=w973, error in=w970, "Title"=w966, "R_array"=w965, "T_array"=w964, "Index"=w963) -> (reference out=w971:refnum<vi>, error out=w969:errorcluster)  [unwired: 16 in]
                n661 = Close Reference(reference=w971, error in (no error)=w969) -> ()  [unwired: 1 out]
              }
            }
          }
          frame Disabled {
          }
        }
        n662 = event-data() -> ()  [unwired: 2 in, 1 out]
      }
      event "_LogFilesPath": Value Change {
        # "Modify window title to show measurement information"
        n663 = event-data() -> ("NewVal"=w991:path)  [unwired: 1 in, 5 out]
        n664 = property class="App"() -> ("App.Dir"=w983:path)  [unwired: 2 in, 2 out]
        n665 = property on="Run Description" class="Str"() -> ("Value"=w984:string)  [unwired: 2 in, 2 out]
        n666 = property on="Bridge Type" class="Enum (strict)"() -> ("RingText.Text"=w985:string)  [unwired: 2 in, 2 out]
        n667 = property on="CS type" class="Enum (strict)"() -> ("RingText.Text"=w986:string)  [unwired: 2 in, 2 out]
        n668 = Path To String(path=w991) -> (string=w987:string)
        n669 = Strip Path(path=w983) -> (name=w982:string)  [unwired: 1 out]
        n670 = Format Into String(format string="%s - %s - %s - %s   (%s)", w982, w984, w985, w986, w987) -> (resulting string=w989:string)  [unwired: 2 in, 1 out]
        n671 = control-ref of="This VI"() -> (w992:refnum<vi>)
        n672 = property class="VI"(reference=w992, "Front Panel.Title"=w989) -> ()  [unwired: 1 in, 2 out]
      }
      event "Reload Calibrations", "Bridge settings.Calibrations Folder": Value Change {
        # "Refresh the list of calibration files"
        n673 = event-data() -> ()  [unwired: 1 in, 1 out]
        n674 = property on="Calibrations Folder" class="Path"() -> ("Value"=w993:path)  [unwired: 2 in, 2 out]
        n675 = control-ref of="Sensor Calibrations"() -> (w1002:refnum<vi>)
        n676 = control-ref of="_CurCalibrations"() -> (w996:refnum<vi>)
        n677 = control-ref of="Calibrations Folder"() -> (w1000:refnum<vi>)
        n678 = control-ref of="_QuickConvertCal"() -> (w999:refnum<vi>)
        n679 = control-ref of="Sensor 1"() -> (w1001:refnum<vi>)
        n680 = Bundle By Name(cluster=w995, "Calibrations Folder"=w993) -> (w994:T50)
        n681 = call "ReloadCalibrations.vi"("error in (no error)"=w998, "Quick convert sensors"=w999, "CurCalibrations"=w996, "Calibration files path"=w1000, "Channel1 sensors"=w1001, "Channels list"=w1002) -> ("error out"=w997:errorcluster)  [unwired: 1 in]
      }
      event Value Change {
        w1009 = refnum<vi> refnum  # XYGraph
        # "Show cursor on plot is \"Cursor\" or \"Delete points\" mode is enabled"
        # "!!NOTE:This routine assumes that XY graph is control #0 on tab page!!"
        n682 = event-data() -> ("NewVal"=w1005:T7)  [unwired: 1 in, 5 out]
        n683 = property on="Channels Panel" class="TabCtl (strict)"() -> ("Pages"=w1013:refnum<vi>[], "Value"=w1012:T8)  [unwired: 2 in, 2 out]
        n684 = Index Array(array=w1013, index=w1012) -> (element=w1011:refnum<vi>)
        n685 = property class="Page"(reference=w1011) -> ("ControlsOnPage"=w1006:refnum<vi>[])  [unwired: 1 in, 2 out]
        n686 = Index Array(array=w1006, index=0) -> (element=w1010:refnum<vi>)
        n687 = Type Cast(type=w1009, x=w1010) -> (*(type *) &x=w1004:refnum<vi>)
        n688 = case shown="\"Erase range\"" w1005 {
          tunnel: w1004 -> [w1014 w1023 w1031 w1039]
          frame "No Selection", Default {
            n689 = property class="XYGraph"(reference=w1014, "Active Cursor"=u32 0, "Cursor.Visible"=FALSE) -> (reference out=w1017:refnum<vi>)  [unwired: 1 in, 1 out]
            n690 = property class="XYGraph"(reference=w1017, "Active Cursor"=u32 1, "Cursor.Visible"=FALSE) -> ()  [unwired: 1 in, 2 out]
          }
          frame "Erase range" {
            n691 = property class="XYGraph"(reference=w1023, "Active Cursor"=u32 0, "Cursor.Visible"=TRUE, "Cursor.Cursor Color"=u32 16777062, "Cursor.Cursor Index"=0, "ActPaletteTool"=0 ("Palette:Active Tool")) -> (reference out=w1026:refnum<vi>)  [unwired: 1 in, 1 out]
            n692 = property class="XYGraph"(reference=w1026, "Active Cursor"=u32 1, "Cursor.Visible"=TRUE, "Cursor.Cursor Color"=u32 6618880) -> ()  [unwired: 1 in, 2 out]
          }
          frame "Cursor mode" {
            n693 = property class="XYGraph"(reference=w1031, "Active Cursor"=u32 0, "Cursor.Visible"=TRUE, "Cursor.Cursor Color"=u32 6618880, "ActPaletteTool"=0 ("Palette:Active Tool")) -> (reference out=w1034:refnum<vi>)  [unwired: 1 in, 1 out]
            n694 = property class="XYGraph"(reference=w1034, "Active Cursor"=u32 1, "Cursor.Visible"=FALSE) -> ()  [unwired: 1 in, 2 out]
          }
          frame "Erase point" {
            n695 = property class="XYGraph"(reference=w1039, "Active Cursor"=u32 0, "Cursor.Visible"=TRUE, "Cursor.Cursor Color"=u32 16777062, "ActPaletteTool"=0 ("Palette:Active Tool")) -> (reference out=w1042:refnum<vi>)  [unwired: 1 in, 1 out]
            n696 = property class="XYGraph"(reference=w1042, "Active Cursor"=u32 1, "Cursor.Visible"=FALSE) -> ()  [unwired: 1 in, 2 out]
          }
        }
      }
      event "R-Plot 0", "R-Plot 1", "R-Plot 2", "R-Plot 3", "R-Plot 4", "R-Plot 5", "R-Plot 6", "R-Plot 7", "R-Plot 8", "R-Plot 9": Mouse Down? {
        # "Disabled"
        n697 = event-data() -> ("CtlRef"=w1048:refnum<vi>, "Button"=w1053:u16, "Mods.Double Click"=w1050:bool)  [unwired: 1 in, 5 out]
        n698 = Equal?(x=u16 1, y=w1053) -> (x = y?=w1051:bool)
        n699 = And(x=w1051, y=w1050) -> (x .and. y?=w1049:bool)
        n700 = disable-structure shown="Disabled" {
          disable-tunnel: w1049 -> [w1056 _]
          disable-tunnel: w1048 -> [w1055 _]
          disable-tunnel: "Mode Buttons" -> [w1054 _]
          frame Disabled {
            n701 = case shown="True" w1056 {
              tunnel: w1054 -> [_ w1058]
              tunnel: w1055 -> [_ w1057]
              frame False {
              }
              frame True {
                n702 = case shown="\"Erase range\"" w1058 {
                  tunnel: w1057 -> [_ w1059]
                  frame "No Selection", Default {
                  }
                  frame "Erase range" {
                    n703 = property class="XYGraph (strict)"(reference=w1059, "ActPaletteTool"=0 ("Palette:Active Tool"), "Active Cursor"=u32 0, "Cursor.Visible"=TRUE) -> ()  [unwired: 1 in, 2 out]
                  }
                }
              }
            }
          }
          frame Enabled {
          }
        }
        n704 = event-data() -> ()  [unwired: 5 in, 1 out]
      }
      event "R-Plot 0", "R-Plot 1", "R-Plot 2", "R-Plot 3", "R-Plot 4", "R-Plot 5", "R-Plot 6", "R-Plot 7", "R-Plot 8", "R-Plot 9": Mouse Down {
        # "Process (double) click on plots in special modes (\"Cursor\", \"Erase\")"
        n705 = event-data() -> ("CtlRef"=w1066:refnum<vi>, "Coords"=w1069:T70, "Button"=w1065:u16, "Mods.Double Click"=w1068:bool, "PlatMods"=w1064:T71)  [unwired: 1 in, 3 out]
        n706 = property on="Mode Buttons" class="RadioBtnsControl (strict)"() -> ("Value"=w1067:T7)  [unwired: 2 in, 2 out]
        n707 = case shown="1" w1065 {
          tunnel: w1069 -> [_ _ w1074]
          tunnel: w1068 -> [_ _ w1073]
          tunnel: w1067 -> [_ _ w1072]
          tunnel: w1066 -> [_ _ w1071]
          tunnel: w1064 -> [_ _ _]
          frame 2 {
          }
          frame Default {
          }
          frame 1 {
            n708 = case shown="\"Cursor mode\"" w1072 {
              tunnel: w1071 -> [_ w1077 w1098 w1106]
              tunnel: w1074 -> [_ w1076 w1097 w1108]
              tunnel: w1073 -> [_ w1075 w1099 w1107]
              frame "No Selection", Default {
              }
              frame "Cursor mode" {
                n709 = case shown="True" w1075 {
                  tunnel: w1077 -> [_ w1087]
                  tunnel: w1076 -> [_ w1085]
                  frame False {
                  }
                  frame True {
                    n710 = invoke class="XYGraph (strict)" method="Map Coords To XY"(reference=w1087, "Coords"=w1085) -> (reference out=w1086:refnum<vi>, "XY"=w1084:cluster{"X":dbl, "Y":dbl})  [unwired: 5 in, 5 out]
                    n711 = Unbundle By Name(w1084) -> ("X"=w1082:dbl)
                    n712 = local read "Data Array"() -> (w1083:T28)
                    n713 = property class="XYGraph (strict)"(reference=w1086, "Active Cursor"=u32 0, "Cursor.Cursor Position"=w1084) -> ()  [unwired: 1 in, 2 out]
                    n714 = for {
                      tunnel: w1083 -> [w1096] mode=indexing
                      tunnel: w1082 -> [w1094]
                      tunnel: [w1090] -> w1081 mode=indexing
                      tunnel: [w1089] -> w1080 mode=indexing
                      n715 = Unbundle By Name(w1096) -> ("R"=w1093:dbl[], "T"=w1092:dbl[], "Time"=w1095:dbl[])
                      n716 = Threshold 1D Array(2:w1094, 3:w1095) -> (0:w1091:dbl)  [unwired: 1 in]
                      n717 = Index Array(array=w1093, index=w1091) -> (element=w1090:dbl)
                      n718 = Index Array(array=w1092, index=w1091) -> (element=w1089:dbl)
                    }
                    n719 = Array To Cluster(array=w1080) -> (cluster=w1078:T62)
                    n720 = Array To Cluster(array=w1081) -> (cluster=w1079:T62)
                    n721 = property on="Time" class="DigNum (strict)"("Value"=w1082) -> ()  [unwired: 2 in, 2 out]
                    n722 = property on="Small R Cluster" class="Clust (strict)"("Value"=w1079) -> ()  [unwired: 2 in, 2 out]
                    n723 = property on="Small T Cluster" class="Clust (strict)"("Value"=w1078) -> ()  [unwired: 2 in, 2 out]
                  }
                }
              }
              frame "Erase range" {
                n724 = case shown="False" w1099 {
                  tunnel: w1098 -> [w1103 _]
                  tunnel: w1097 -> [w1102 _]
                  frame False {
                    n725 = invoke class="XYGraph (strict)" method="Map Coords To XY"(reference=w1103, "Coords"=w1102) -> (reference out=w1105:refnum<vi>, "XY"=w1100:cluster{"X":dbl, "Y":dbl})  [unwired: 5 in, 5 out]
                    n726 = property class="XYGraph (strict)"(reference=w1105, "Active Cursor"=u32 0, "Cursor.Cursor Position"=w1100, "Active Cursor"=u32 1, "Cursor.Cursor Position"=w1100) -> ()  [unwired: 1 in, 2 out]
                  }
                  frame True {
                  }
                }
              }
              frame "Erase point" {
                n727 = case shown="True" w1107 {
                  tunnel: w1106 -> [w1113 w1128]
                  tunnel: w1108 -> [w1112 _]
                  frame False {
                    n728 = invoke class="XYGraph (strict)" method="Map Coords To XY"(reference=w1113, "Coords"=w1112) -> (reference out=w1111:refnum<vi>, "XY"=w1110:cluster{"X":dbl, "Y":dbl})  [unwired: 5 in, 5 out]
                    n729 = property class="XYGraph (strict)"(reference=w1111, "Active Cursor"=u32 0, "Cursor.Cursor Position"=w1110) -> ()  [unwired: 1 in, 2 out]
                  }
                  frame True {
                    n730 = property class="XYGraph (strict)"(reference=w1128, "Active Cursor"=u32 0) -> ("Cursor.Cursor X"=w1116:dbl)  [unwired: 1 in, 2 out]
                    n731 = local read "Channels Panel"() -> (w1115:T8)
                    n732 = local read "Data Array"() -> (w1114:T28)
                    n733 = Index Array(array=w1114, index=w1115) -> (element=w1121:cluster{"R":dbl[], "T":dbl[], "Time":dbl[]})
                    n734 = Unbundle By Name(w1121) -> ("R"=w1117:dbl[], "T"=w1118:dbl[], "Time"=w1119:dbl[])
                    n735 = Threshold 1D Array(2:w1116, 3:w1119) -> (0:w1120:dbl)  [unwired: 1 in]
                    n736 = Delete From Array(array=w1117, index=w1120) -> (array with subset deleted=w1124:dbl[])  [unwired: 1 in, 1 out]
                    n737 = Delete From Array(array=w1118, index=w1120) -> (array with subset deleted=w1123:dbl[])  [unwired: 1 in, 1 out]
                    n738 = Delete From Array(array=w1119, index=w1120) -> (array with subset deleted=w1122:dbl[])  [unwired: 1 in, 1 out]
                    n739 = Bundle By Name(cluster=w1121, "R"=w1124, "T"=w1123, "Time"=w1122) -> (w1125:cluster{"R":dbl[], "T":dbl[], "Time":dbl[]})
                    n740 = Replace Array Subset(array=w1114, new element=w1125, index=w1115) -> (w1126:T28)
                    n741 = local write "Data Array"(w1126) -> ()
                  }
                }
              }
            }
            "_LMBDown" <- TRUE ("Mouse down")
          }
        }
      }
      event "R-Plot 0", "R-Plot 1", "R-Plot 2", "R-Plot 3", "R-Plot 4", "R-Plot 5", "R-Plot 6", "R-Plot 7", "R-Plot 8", "R-Plot 9": Mouse Move {
        # "Process mouse movement over plots in special modes (\"Cursor\", \"Erase\")"
        n742 = event-data() -> ("CtlRef"=w1131:refnum<vi>, "Coords"=w1132:T70)  [unwired: 1 in, 3 out]
        n743 = property on="Mode Buttons" class="RadioBtnsControl (strict)"() -> ("Value"=w1135:T7)  [unwired: 2 in, 2 out]
        n744 = local read "_LMBDown"() -> (w1136:bool)
        n745 = Equal?(x=w1135, y=Cursor_Controls."Erase range" ("Mode Buttons")) -> (x = y?=w1133:bool)
        n746 = And(x=w1136, y=w1133) -> (x .and. y?=w1134:bool)
        n747 = case shown="True" w1134 {
          tunnel: w1132 -> [_ w1138]
          tunnel: w1131 -> [_ w1137]
          frame False {
          }
          frame True {
            n748 = invoke class="XYGraph (strict)" method="Map Coords To XY"(reference=w1137, "Coords"=w1138) -> (reference out=w1141:refnum<vi>, "XY"=w1140:cluster{"X":dbl, "Y":dbl})  [unwired: 5 in, 5 out]
            n749 = property class="XYGraph (strict)"(reference=w1141, "Active Cursor"=u32 1, "Cursor.Cursor Position"=w1140) -> ()  [unwired: 1 in, 2 out]
          }
        }
      }
      event "R-Plot 0", "R-Plot 1", "R-Plot 2", "R-Plot 3", "R-Plot 4", "R-Plot 5", "R-Plot 6", "R-Plot 7", "R-Plot 8", "R-Plot 9": Mouse Up {
        n750 = event-data() -> ("CtlRef"=w1145:refnum<vi>, "Button"=w1143:u16)  [unwired: 1 in, 6 out]
        n751 = property on="Mode Buttons" class="RadioBtnsControl (strict)"() -> ("Value"=w1146:T7)  [unwired: 2 in, 2 out]
        n752 = property class="XYGraph (strict)"(reference=w1145) -> ("ActPaletteTool"=w1144:i32)  [unwired: 1 in, 2 out]
        n753 = case shown="1" w1143 {
          tunnel: w1146 -> [_ w1150]
          tunnel: w1145 -> [_ w1149]
          tunnel: w1144 -> [_ w1148]
          frame Default {
          }
          frame 1 {
            n754 = local read "_LMBDown"() -> (w1147:bool)
            n755 = case shown="0" w1148 {
              tunnel: w1150 -> [_ w1155]
              tunnel: w1149 -> [_ w1154]
              tunnel: w1147 -> [_ w1152]
              frame Default {
                n756 = property on="Mode Buttons" class="RadioBtnsControl (strict)"("Val(Sgnl)"=T56."No Selection" ("Value (Signaling)")) -> ()  [unwired: 2 in, 2 out]
              }
              frame 0 {
                n757 = Equal?(x=w1155, y=T56."Erase range") -> (x = y?=w1158:bool)
                n758 = And(x=w1152, y=w1158) -> (x .and. y?=w1157:bool)
                n759 = case shown="True" w1157 {
                  tunnel: w1154 -> [_ w1181]
                  frame False {
                  }
                  frame True {
                    n760 = local read "Channels Panel"() -> (w1180:T8)
                    n761 = property class="XYGraph (strict)"(reference=w1181, "Active Cursor"=u32 0, "Active Cursor"=u32 1) -> ("Cursor.Cursor X"=w1178:dbl, "Cursor.Cursor X"=w1159:dbl)  [unwired: 1 in, 2 out]
                    n762 = local read "Data Array"() -> (w1175:T28)
                    n763 = Max & Min(x=w1178, y=w1159) -> (max(x,y)=w1168:dbl, min(x,y)=w1161:dbl)
                    n764 = Index Array(array=w1175, index=w1180) -> (element=w1171:cluster{"R":dbl[], "T":dbl[], "Time":dbl[]})
                    n765 = Unbundle By Name(w1171) -> ("R"=w1169:dbl[], "T"=w1170:dbl[], "Time"=w1167:dbl[])
                    n766 = Threshold 1D Array(2:w1168, 3:w1167) -> (0:w1165:dbl)  [unwired: 1 in]
                    n767 = Threshold 1D Array(2:w1161, 3:w1167) -> (0:w1166:dbl)  [unwired: 1 in]
                    n768 = Subtract(x=w1165, y=w1166) -> (x-y=w1164:dbl)
                    n769 = Delete From Array(array=w1169, length=w1164, index=w1166) -> (array with subset deleted=w1174:dbl[])  [unwired: 1 out]
                    n770 = Delete From Array(array=w1170, length=w1164, index=w1166) -> (array with subset deleted=w1173:dbl[])  [unwired: 1 out]
                    n771 = Delete From Array(array=w1167, length=w1164, index=w1166) -> (array with subset deleted=w1172:dbl[])  [unwired: 1 out]
                    n772 = Bundle By Name(cluster=w1171, "R"=w1174, "T"=w1173, "Time"=w1172) -> (w1176:cluster{"R":dbl[], "T":dbl[], "Time":dbl[]})
                    n773 = Replace Array Subset(array=w1175, new element=w1176, index=w1180) -> (w1177:T28)
                    n774 = local write "Data Array"(w1177) -> ()
                    n775 = property class="XYGraph (strict)"(reference=w1181, "Active Cursor"=u32 0, "Cursor.Cursor X"=w1161, "Active Cursor"=u32 1, "Cursor.Cursor X"=w1161) -> ()  [unwired: 1 in, 2 out]
                  }
                }
                n776 = local write "_LMBDown"(FALSE ("Mouse down")) -> ()
              }
            }
          }
        }
      }
      event "R-Plot 0", "R-Plot 1", "R-Plot 2", "R-Plot 3", "R-Plot 4", "R-Plot 5", "R-Plot 6", "R-Plot 7", "R-Plot 8", "R-Plot 9": Mouse Leave {
        n777 = event-data() -> ()  [unwired: 1 in, 4 out]
        n778 = local write "_LMBDown"(FALSE ("Mouse down")) -> ()
      }
      event "R-Plot 0", "R-Plot 1", "R-Plot 2", "R-Plot 3", "R-Plot 4", "R-Plot 5", "R-Plot 6", "R-Plot 7", "R-Plot 8", "R-Plot 9": Scale Range Change {
        w1186 = u8 0 ("X Scale.Scale Fit")
        # "Disable plot autoscaling if the user has changed the scale of the plot manualy"
        n779 = event-data() -> ("CtlRef"=w1185:refnum<vi>)  [unwired: 1 in, 7 out]
        n780 = property class="XYGraph (strict)"(reference=w1185, "XScale.ScaleFit"=w1186, "YScale.ScaleFit"=w1186) -> ()  [unwired: 1 in, 2 out]
      }
      event "R-Plot 0", "R-Plot 1", "R-Plot 2", "R-Plot 3", "R-Plot 4", "R-Plot 5", "R-Plot 6", "R-Plot 7", "R-Plot 8", "R-Plot 9": Shortcut Menu Activation? {
        w1195 = string[] ["Log Y"] ("item names")
        w1197 = string[] ["Zoom In to Last Data", "Autoscale XY"] ("item names")
        # "Add extra options to the plots context menu"
        n781 = event-data() -> ("MenuRef"=w1199:refnum<k9>, "CtlRef"=w1191:refnum<vi>)  [unwired: 1 in]
        n782 = Insert Menu Items(4:10, 7:w1197, 8:w1197, 9:w1199) -> (3:w1193:refnum<k9>)  [unwired: 2 in, 2 out]
        n783 = property class="XYGraph (strict)"(reference=w1191) -> ("YScale.Mapping Mode"=w1190:u8)  [unwired: 1 in, 2 out]
        n784 = Insert Menu Items(4:14, 7:w1195, 8:w1195, 9:w1193) -> (3:w1192:refnum<k9>)  [unwired: 2 in, 2 out]
        n785 = Not Equal To 0?(x=w1190) -> (x != 0?=w1189:bool)
        n786 = Set Menu Item Info(6:w1189, 7:"Log Y", 11:w1192) -> ()  [unwired: 4 in, 2 out]
        n787 = local read "_LMBDown"() -> (w1196:bool)
        n788 = event-data("Discard?"=w1196) -> ()  [unwired: 1 in, 1 out]
      }
      event "R-Plot 0", "R-Plot 1", "R-Plot 2", "R-Plot 3", "R-Plot 4", "R-Plot 5", "R-Plot 6", "R-Plot 7", "R-Plot 8", "R-Plot 9": Shortcut Menu Selection (User) {
        # "Zoom in to last \"Miniplot points\". Zoom out a bit to have some space around the points"
        n789 = event-data() -> ("CtlRef"=w1205:refnum<vi>, "ItemTag"=w1203:string)  [unwired: 1 in]
        n790 = Type Cast(type=refnum<vi> refnum ("R-Plot 0"), x=w1205) -> (*(type *) &x=w1204:refnum<vi>)
        n791 = property on="Runtime Settings" class="Clust (strict)"() -> ("Value"=w1201:T27)  [unwired: 2 in, 2 out]
        n792 = case shown="\"Zoom In to Last Data\"" w1203 {
          tunnel: w1204 -> [_ w1207 w1236 w1242]
          tunnel: w1201 -> [_ _ w1208 _]
          frame Default {
          }
          frame "Autoscale XY" {
            w1206 = u8 2 ("X Scale.Scale Fit")
            n793 = property class="XYGraph (strict)"(reference=w1207, "XScale.ScaleFit"=w1206, "YScale.ScaleFit"=w1206) -> ()  [unwired: 1 in, 2 out]
          }
          frame "Zoom In to Last Data" {
            w1232 = u8 0 ("Y Scale.Scale Fit")
            n794 = property class="XYGraph (strict)"(reference=w1236) -> (reference out=w1233:refnum<vi>, "Value"=w1235:cluster{dbl[], dbl[]})  [unwired: 1 in, 1 out]
            n795 = Unbundle By Name(w1208) -> ("Miniplot Time"=w1231:dbl)
            n796 = Unbundle(w1235) -> (w1210:dbl[], w1234:dbl[])
            n797 = Multiply(x=w1231, y=60.0) -> (x*y=w1227:dbl)
            n798 = Reverse 1D Array(array=w1210) -> (reversed array=w1215:dbl[])
            n799 = Reverse 1D Array(array=w1234) -> (reversed array=w1223:dbl[])
            n800 = Index Array(array=w1215) -> (element=w1229:dbl)  [unwired: 1 in]
            n801 = Multiply(x=0.5, y=w1227) -> (x*y=w1228:dbl)
            n802 = Add(x=w1228, y=w1229) -> (x+y=w1226:dbl)
            n803 = Subtract(x=w1229, y=w1227) -> (x-y=w1224:dbl)
            n804 = call "Improved Threshold Detector.71.vi"("Threshold"=w1224, "Array"=w1210) -> ("Positive transition indices"=w1211:i32[])  [unwired: 8 in, 1 out]
            n805 = Index Array(array=w1211) -> (element=w1237:i32)  [unwired: 1 in]
            n806 = Array Size(array=w1210) -> (size(s)=w1213:i32)
            n807 = Index Array(array=w1210, index=w1237) -> (element=w1209:dbl)
            n808 = Subtract(x=w1213, y=w1237) -> (x-y=w1212:i32)
            n809 = Array Subset(array=w1223, length=w1212) -> (w1222:dbl[])  [unwired: 1 in]
            n810 = Array Max & Min(array=w1222) -> (max value=w1219:dbl, min value=w1218:dbl)  [unwired: 2 out]
            n811 = Subtract(x=w1219, y=w1218) -> (x-y=w1221:dbl)
            n812 = Divide(x=w1221, y=2.0) -> (x/y=w1217:dbl)
            n813 = Add(x=w1219, y=w1217) -> (x+y=w1214:dbl)
            n814 = Subtract(x=w1218, y=w1217) -> (x-y=w1216:dbl)
            n815 = property class="XYGraph (strict)"(reference=w1233, "XScale.ScaleFit"=w1232, "YScale.ScaleFit"=w1232, "XScale.Maximum"=w1226, "XScale.Minimum"=w1209, "YScale.Maximum"=w1214, "YScale.Minimum"=w1216) -> ()  [unwired: 1 in, 2 out]
          }
          frame "Log Y" {
            n816 = property class="XYGraph (strict)"(reference=w1242) -> (reference out=w1241:refnum<vi>, "YScale.Mapping Mode"=w1240:u8)  [unwired: 1 in, 1 out]
            n817 = Equal To 0?(x=w1240) -> (x = 0?=w1239:bool)
            n818 = Boolean To (0,1)(Boolean=w1239) -> (0, 1=w1238:i16)
            n819 = property class="XYGraph (strict)"(reference=w1241, "YScale.Mapping Mode"=w1238) -> ()  [unwired: 1 in, 2 out]
          }
        }
      }
      event "uPlots.uPlot 0", "uPlots.uPlot 1", "uPlots.uPlot 2", "uPlots.uPlot 3", "uPlots.uPlot 4", "uPlots.uPlot 5", "uPlots.uPlot 6", "uPlots.uPlot 7", "uPlots.uPlot 8", "uPlots.uPlot 9": Mouse Down {
        # "Switch to big plot on double click on small plot"
        n820 = event-data() -> ("Mods.Double Click"=w1245:bool, "CtlRef"=w1244:refnum<vi>)  [unwired: 1 in]
        n821 = case shown="True" w1245 {
          tunnel: w1244 -> [_ w1248]
          frame False {
          }
          frame True {
            n822 = property class="XYGraph (strict)"(reference=w1248) -> ("Label.Text"=w1249:string)  [unwired: 1 in, 2 out]
            n823 = Reverse String(1:w1249) -> (0:w1250:string)
            n824 = Decimal String To Number(string=w1250, default (0L)=8 ("default (0 I32)")) -> (number=w1247:i32)  [unwired: 1 in, 1 out]
            n825 = property on="Channels Panel" class="TabCtl (strict)"("Val(Sgnl)"=w1247) -> ()  [unwired: 2 in, 2 out]
          }
        }
      }
      event "Erase all": Value Change {
        # "Clear data array.\nReset PID."
        n826 = event-data() -> ()  [unwired: 1 in, 6 out]
        n827 = local read "Channels Panel"() -> (w1254:T8)
        n828 = local read "Data Array"() -> (w1255:T28)
        n829 = Replace Array Subset(array=w1255, new element=cluster{"R":dbl[], "T":dbl[], "Time":dbl[]} {"R"=[], "T"=[], "Time"=[]} ("new element/subarray"), index=w1254) -> (w1253:T28)
        n830 = local write "Data Array"(w1253) -> ()
        n831 = disable-structure shown="Disabled" {
          frame Disabled {
            n832 = Initialize Array(cluster{"R":dbl[], "T":dbl[], "Time":dbl[]} {"R"=[], "T"=[], "Time"=[]}, 10 ("dimension size")) -> ()  [unwired: 1 out]
          }
          frame Enabled {
          }
        }
      }
      event "Clear all plots": Value Change {
        n833 = event-data() -> ()  [unwired: 1 in, 6 out]
        n834 = Initialize Array(cluster{"R":dbl[], "T":dbl[], "Time":dbl[]} {"R"=[], "T"=[], "Time"=[]}, 10 ("dimension size")) -> (w1260:cluster{"R":dbl[], "T":dbl[], "Time":dbl[]}[])
        n835 = local write "Data Array"(w1260) -> ()
      }
      event "Bridge settings.Bridge Type": Value Change {
        # "Select bridge type (AVS/zBridge). Show/hide corresponding controls."
        n836 = event-data() -> ("NewVal"=w1264:T61)  [unwired: 1 in, 5 out]
        n837 = flat-sequence {
          tunnel: w1264 -> [w1273]
          frame #0 {
            w1269 = u8 0 ("Disabled")
            w1272 = u8 0 ("Disabled")
            w1271 = FALSE ("Visible")
            w1270 = u8 2 ("Disabled")
            n838 = property on="AVS RS232 Port" class="VISAName"("Visible"=w1271, "Disabled"=w1270) -> ()  [unwired: 2 in, 2 out]
            n839 = property on="zBridge settings" class="Bool"("Visible"=w1271, "Disabled"=w1270) -> ()  [unwired: 2 in, 2 out]
            n840 = property on="Lower Panel" class="TabCtl (strict)"("Disabled"=w1269) -> ()  [unwired: 2 in, 2 out]
            n841 = property on="AVS GPIB Address" class="VISAName"("Visible"=w1271, "Disabled"=w1270) -> ()  [unwired: 2 in, 2 out]
            n842 = property on="Main Panel" class="TabCtl (strict)"("Disabled"=w1269) -> ()  [unwired: 2 in, 2 out]
            n843 = property on="Read AVS channels from" class="DigNum (strict)"("Disabled"=w1272) -> ()  [unwired: 2 in, 2 out]
            n844 = property on="Last Channel" class="DigNum (strict)"("Disabled"=w1272) -> ()  [unwired: 2 in, 2 out]
            n845 = property on="Stabilisation Delay" class="DigNum (strict)"("Disabled"=w1272) -> ()  [unwired: 2 in, 2 out]
            n846 = property on="Averages" class="DigNum (strict)"("Disabled"=w1272) -> ()  [unwired: 2 in, 2 out]
            n847 = property on="Delay Between Scans" class="DigNum (strict)"("Disabled"=w1272) -> ()  [unwired: 2 in, 2 out]
            n848 = call "Build ranges list.vi"("Values"="-1\r\n0\r\n1\r\n2\r\n3\r\n4\r\n5\r\n6\r\n7", "Strings"="n.a.\r\nopen\r\n2 Ohm\r\n20 Ohm\r\n200 Ohm\r\n2k Ohm\r\n20k Ohm\r\n200k Ohm\r\n2M Ohm") -> ("Strings and Values"=w1268:cluster{"String":string, "Value":i32}[])  [unwired: 4 in]
            n849 = property on="Range 0" class="Ring (strict)"("StringsAndValues[]"=w1268) -> ()  [unwired: 2 in, 2 out]
            n850 = property on="Range 1" class="Ring (strict)"("StringsAndValues[]"=w1268) -> ()  [unwired: 2 in, 2 out]
            n851 = property on="Range 2" class="Ring (strict)"("StringsAndValues[]"=w1268) -> ()  [unwired: 2 in, 2 out]
            n852 = property on="Range 3" class="Ring (strict)"("StringsAndValues[]"=w1268) -> ()  [unwired: 2 in, 2 out]
            n853 = property on="Range 4" class="Ring (strict)"("StringsAndValues[]"=w1268) -> ()  [unwired: 2 in, 2 out]
            n854 = property on="Range 5" class="Ring (strict)"("StringsAndValues[]"=w1268) -> ()  [unwired: 2 in, 2 out]
            n855 = property on="Range 6" class="Ring (strict)"("StringsAndValues[]"=w1268) -> ()  [unwired: 2 in, 2 out]
            n856 = property on="Range 7" class="Ring (strict)"("StringsAndValues[]"=w1268) -> ()  [unwired: 2 in, 2 out]
          }
          frame #1 {
            n857 = case shown="\"AVS48SI (RS232 interface)\"" w1273 {
              frame "AVS47A (GPIB interface)" {
                n858 = local write "AVS Scan Parameters"(enum32{"Page 1", "Page 2"}."Page 1" ("Scan Parameters")) -> ()
                n859 = property on="AVS GPIB Address" class="VISAName"("Visible"=TRUE, "Disabled"=u8 0) -> ()  [unwired: 2 in, 2 out]
              }
              frame "AVS47B (RS232 interface)" {
                w1277 = u8 2 ("Disabled")
                n860 = local write "AVS Scan Parameters"(enum32{"Page 1", "Page 2"}."Page 1" ("Scan Parameters")) -> ()
                n861 = property on="AVS RS232 Port" class="VISAName"("Visible"=TRUE, "Disabled"=u8 0) -> ()  [unwired: 2 in, 2 out]
                n862 = property on="Read AVS channels from" class="DigNum (strict)"("Disabled"=w1277) -> ()  [unwired: 2 in, 2 out]
                n863 = property on="Last Channel" class="DigNum (strict)"("Disabled"=w1277) -> ()  [unwired: 2 in, 2 out]
              }
              frame "AVS48SI (RS232 interface)" {
                w1284 = u8 2 ("Disabled")
                n864 = property on="Read AVS channels from" class="DigNum (strict)"("Disabled"=w1284) -> ()  [unwired: 2 in, 2 out]
                n865 = property on="Last Channel" class="DigNum (strict)"("Disabled"=w1284) -> ()  [unwired: 2 in, 2 out]
                n866 = property on="AVS RS232 Port" class="VISAName"("Visible"=TRUE, "Disabled"=u8 0) -> ()  [unwired: 2 in, 2 out]
                n867 = local write "AVS Scan Parameters"(enum32{"Page 1", "Page 2"}."Page 1" ("Scan Parameters")) -> ()
                n868 = call "Build ranges list.vi"("Values"="-1\r\n0\r\n1\r\n2\r\n3\r\n4\r\n5\r\n6\r\n7", "Strings"="n.a.\r\n3 Ohm\r\n30 Ohm\r\n300 Ohm\r\n3k Ohm\r\n30k Ohm\r\n300k Ohm\r\n3M Ohm\r\n30m Ohm") -> ("Strings and Values"=w1282:cluster{"String":string, "Value":i32}[])  [unwired: 4 in]
                n869 = property on="Range 0" class="Ring (strict)"("StringsAndValues[]"=w1282) -> ()  [unwired: 2 in, 2 out]
                n870 = property on="Range 1" class="Ring (strict)"("StringsAndValues[]"=w1282) -> ()  [unwired: 2 in, 2 out]
                n871 = property on="Range 2" class="Ring (strict)"("StringsAndValues[]"=w1282) -> ()  [unwired: 2 in, 2 out]
                n872 = property on="Range 3" class="Ring (strict)"("StringsAndValues[]"=w1282) -> ()  [unwired: 2 in, 2 out]
                n873 = property on="Range 4" class="Ring (strict)"("StringsAndValues[]"=w1282) -> ()  [unwired: 2 in, 2 out]
                n874 = property on="Range 5" class="Ring (strict)"("StringsAndValues[]"=w1282) -> ()  [unwired: 2 in, 2 out]
                n875 = property on="Range 6" class="Ring (strict)"("StringsAndValues[]"=w1282) -> ()  [unwired: 2 in, 2 out]
                n876 = property on="Range 7" class="Ring (strict)"("StringsAndValues[]"=w1282) -> ()  [unwired: 2 in, 2 out]
              }
              frame "AVS Emulation" {
                n877 = local write "AVS Scan Parameters"(enum32{"Page 1", "Page 2"}."Page 1" ("Scan Parameters")) -> ()
              }
              frame "Impedance Bridge" {
                w1291 = u8 2 ("Disabled")
                n878 = local write "AVS Scan Parameters"(enum32{"Page 1", "Page 2"}."Page 2" ("Scan Parameters")) -> ()
                n879 = property on="zBridge settings" class="Bool"("Visible"=TRUE, "Disabled"=u8 0) -> ()  [unwired: 2 in, 2 out]
                n880 = property on="Read AVS channels from" class="DigNum (strict)"("Disabled"=w1291) -> ()  [unwired: 2 in, 2 out]
                n881 = property on="Last Channel" class="DigNum (strict)"("Disabled"=w1291) -> ()  [unwired: 2 in, 2 out]
                n882 = property on="Stabilisation Delay" class="DigNum (strict)"("Disabled"=w1291) -> ()  [unwired: 2 in, 2 out]
                n883 = property on="Averages" class="DigNum (strict)"("Disabled"=w1291) -> ()  [unwired: 2 in, 2 out]
                n884 = property on="Delay Between Scans" class="DigNum (strict)"("Disabled"=w1291) -> ()  [unwired: 2 in, 2 out]
              }
              frame "Disabled", Default {
                w1293 = u8 2 ("Disabled")
                n885 = property on="Lower Panel" class="TabCtl (strict)"("Disabled"=w1293) -> ()  [unwired: 2 in, 2 out]
                n886 = property on="Main Panel" class="TabCtl (strict)"("Disabled"=w1293) -> ()  [unwired: 2 in, 2 out]
              }
            }
          }
        }
      }
      event "Runtime Settings.Plot type": Value Change {
        # "Iterate through first 10 pages (plots only)"
        # "Switch between RxTime and TxTime plots"
        n887 = event-data() -> ("NewVal"=w1304:enum16{"R vs Time", "T vs Time"})  [unwired: 1 in, 5 out]
        n888 = Unbundle By Name(w1296) -> ("Reset PID loop"=w1295:refnum<user-event>)
        n889 = Equal To 0?(x=w1304) -> (x = 0?=w1303:bool)
        n890 = Select(t=u32 10532351, s=w1303, f=u32 16711680) -> (s? t:f=w1300:u32)
        n891 = property on="uPlots" class="Clust (strict)"() -> ("Controls[]"=w1298:refnum<vi>[])  [unwired: 2 in, 2 out]
        n892 = property on="Channels Panel" class="TabCtl (strict)"() -> ("Pages"=w1305:refnum<vi>[])  [unwired: 2 in, 2 out]
        n893 = for {
          N: 10 -> [_]
          tunnel: w1305 -> [w1315] mode=indexing
          tunnel: w1300 -> [w1308]
          tunnel: w1298 -> [w1306] mode=indexing
          # "!!NOTE:This routine assumes that graph is control #0 on page!!"
          n894 = property class="Page"(reference=w1315) -> ("ControlsOnPage"=w1313:refnum<vi>[])  [unwired: 1 in, 2 out]
          n895 = Type Cast(type=refnum<vi> refnum ("R-Plot 0"), x=w1306) -> (*(type *) &x=w1307:refnum<vi>)
          n896 = Index Array(array=w1313, index=0) -> (element=w1311:refnum<vi>)
          n897 = Type Cast(type=refnum<vi> refnum ("R-Plot 0"), x=w1311) -> (*(type *) &x=w1310:refnum<vi>)
          n898 = property class="XYGraph (strict)"(reference=w1310, "Plot.Plot Color"=w1308, "Plot.Fill/Pt. Color"=w1308) -> ()  [unwired: 1 in, 2 out]
          n899 = property class="XYGraph (strict)"(reference=w1307, "Plot.Plot Color"=w1308, "Plot.Fill/Pt. Color"=w1308) -> ()  [unwired: 1 in, 2 out]
        }
        n900 = Generate User Event(user event=w1295, event data cluster="" ("event data")) -> ()  [unwired: 2 in, 2 out]
      }
      event "Runtime Settings.Read AVS channels from", "Runtime Settings.Last Channel": Value Change {
        # "Change enabled channels for the AVS bridge"
        n901 = event-data() -> ()  [unwired: 1 in, 6 out]
        n902 = Unbundle By Name(w1318) -> ("UpdateChannelInfo"=w1317:refnum<user-event>)
        n903 = Generate User Event(user event=w1317, event data cluster=bool[] [] ("event data")) -> ()  [unwired: 2 in, 2 out]
      }
      event "Runtime Settings.Filter Graphs": Value Change {
        # "Graph filtering controls"
        n904 = event-data() -> ("NewVal"=w1321:bool)  [unwired: 1 in, 5 out]
        n905 = call "IsDisabled.vi"("Enabled?"=w1321) -> ("Numeric"=w1322:i16)
        n906 = property on="Y_min" class="DigNum (strict)"("Disabled"=w1322) -> ()  [unwired: 2 in, 2 out]
        n907 = property on="Y_max" class="DigNum (strict)"("Disabled"=w1322) -> ()  [unwired: 2 in, 2 out]
      }
      event "Channels Panel": Value Change {
        # "Show hide bottom Impedance/Temperature panel depending on the current tab page"
        n908 = event-data() -> ("NewVal"=w1325:T8)  [unwired: 1 in, 5 out]
        n909 = case shown="Default" w1325 {
          tunnel: [TRUE ("Visible") FALSE ("Visible")] -> w1324
          frame Default {
            n910 = property on="Mode Buttons" class="RadioBtnsControl (strict)"() -> ("Value"=w1327:T7)  [unwired: 2 in, 2 out]
            n911 = property on="Data History/RT Settings" class="TabCtl (strict)"("Value"=enum32{"History", "Settings"}."History" ("Data History")) -> ()  [unwired: 2 in, 2 out]
            n912 = property on="Mode Buttons" class="RadioBtnsControl (strict)"("Val(Sgnl)"=w1327) -> ()  [unwired: 2 in, 2 out]
          }
          frame "All", "PID loop" {
            n913 = property on="Data History/RT Settings" class="TabCtl (strict)"("Value"=enum32{"History", "Settings"}."Settings" ("Data History")) -> ()  [unwired: 2 in, 2 out]
          }
        }
        n914 = property on="Graph Controls Bar" class="TabCtl (strict)"("Visible"=w1324) -> ()  [unwired: 2 in, 2 out]
      }
      event Value Change {
        # "Calibration changed - update calibrations list"
        n915 = event-data() -> ()  [unwired: 1 in, 6 out]
        n916 = property on="Sensor Calibrations" class="Clust (strict)"() -> ("Controls[]"=w1334:refnum<vi>[])  [unwired: 2 in, 2 out]
        n917 = Array Size(array=w1334) -> (size(s)=w1335:i32)
        n918 = for {
          N: w1335 -> [_]
          tunnel: w1334 -> [w1339] mode=indexing
          tunnel: [w1336] -> w1333 mode=indexing
          w1338 = refnum<vi> refnum  # Ring
          n919 = Type Cast(type=w1338, x=w1339) -> (*(type *) &x=w1337:refnum<vi>)
          n920 = property class="Ring"(reference=w1337) -> ("RingText.Text"=w1336:string)  [unwired: 1 in, 2 out]
        }
        n921 = Array To Cluster(array=w1333) -> (cluster=→"_CurCalibrations":T33)
      }
      event "Data Logging Settings": Value Change {
        # "Log file settings changed. Generate new log file name"
        n922 = event-data() -> ()  [unwired: 1 in, 3 out]
        n923 = local read "Data Logging Settings"() -> (w1348:T37)
        n924 = Unbundle By Name(w1348) -> ("Run Description"=w1342:string, "Filenames Suffix"=w1343:string, "Log Files Folder"=w1349:path, "Log Files Name"=w1347:string, "Automode Files Name"=w1346:string)
        n925 = call "MGI Make String Filesafe.vi"("String In"=w1342) -> ("Filesafe String Out"=w1341:string)
        n926 = call "GeneratePaths.vi"("Filename Suffix"=w1343, "Run description"=w1341, "AVS_Path"=w1349, "AVS_FName"=w1347, "CAL_Path"=w1349, "CAL_FName"=w1346) -> ("Generated Log path"=w1345:path, "Generated Calib path"=w1344:path)  [unwired: 8 in]
        n927 = local write "_LogFilesPath"(w1345) -> ()
        n928 = local write "_CalibFilesPath"(w1344) -> ()
      }
      event "Convert R-T": Mouse Down; "QuickR": Value Change {
        # "Quick convert R->T"
        n929 = event-data() -> ()  [unwired: 1 in, 4 out]
        n930 = Unbundle By Name(w1350) -> ("Calibrations Folder"=w1351:path)
        n931 = property on="_QuickConvertCal" class="Ring (strict)"() -> ("Strings []"=w1354:string[], "Value"=w1355:u16)  [unwired: 2 in, 2 out]
        n932 = Index Array(array=w1354, index=w1355) -> (element=w1353:string)
        n933 = call "SelectSensor-txt no ext.vi"("Path"=w1351, "Resistance"="QuickR", "Select sensor"=w1353) -> ("error out"=w1352:errorcluster, "Temperature"=→"T7":dbl)
      }
      event "T Sweep.Current": Value Change {
        # "Current/ Setpoint value is changed"
        n934 = event-data() -> ("NewVal"=→"_I3SetPnt":dbl)  [unwired: 1 in, 5 out]
        n935 = Unbundle By Name(w1360) -> ("Reset PID loop"=w1359:refnum<user-event>)
        n936 = Generate User Event(user event=w1359, event data cluster="" ("event data")) -> ()  [unwired: 2 in, 2 out]
      }
      event Value Change {
        w1364 = FALSE ("Value (Signaling)")
        # "Changed Channel1 automatic mode"
        n937 = event-data() -> ("NewVal"=w1366:T39)  [unwired: 1 in, 5 out]
        n938 = Unbundle By Name(w1368) -> ("TempStabilized"=w1367:refnum<user-event>)
        n939 = property on="CS.Mode1.Start" class="Bool (strict)"("Val(Sgnl)"=w1364) -> ()  [unwired: 2 in, 2 out]
        n940 = property on="CS.Mode2.Start" class="Bool (strict)"("Val(Sgnl)"=w1364) -> ()  [unwired: 2 in, 2 out]
        n941 = case shown="\"Mode 1\"" w1366 {
          tunnel: [FALSE ("Automatic mode ON") TRUE ("Automatic mode ON") TRUE ("Automatic mode ON")] -> w1369
          tunnel: w1367 -> [_ w1379 _]
          tunnel: [0 1 2] -> w1365
          frame "Manual" {
            # "Set manual mode currents \nequal to last automode \nvalues."
            n942 = local read "CS.Automode Current"() -> (w1372:T23[])
            n943 = Index Array(array=w1372) -> (element #1=w1376:T23, element #2=w1375:T23, element #3=w1374:T23, element #4=w1373:T23)  [unwired: 4 in]
            n944 = property on="I" class="DigNum (strict)"("Val(Sgnl)"=w1376) -> ()  [unwired: 2 in, 2 out]
            n945 = property on="I" class="DigNum (strict)"("Val(Sgnl)"=w1375) -> ()  [unwired: 2 in, 2 out]
            n946 = property on="I" class="DigNum (strict)"("Val(Sgnl)"=w1374) -> ()  [unwired: 2 in, 2 out]
            n947 = property on="I" class="DigNum (strict)"("Val(Sgnl)"=w1373) -> ()  [unwired: 2 in, 2 out]
          }
          frame "Mode 1" {
            # "Set automatic mode currents equal to last manual values."
            n948 = local read "CS.Current Value"() -> (w1382:dbl[])
            n949 = Multiply(x=1000.0, y=w1382) -> (x*y=w1380:dbl[])
            n950 = local write "CS.Automode Current"(w1380) -> ()
            n951 = Generate User Event(user event=w1379, event data cluster=FALSE ("event data")) -> ()  [unwired: 2 in, 2 out]
          }
          frame "Mode2" {
            # "Set automatic mode currents equal to last manual values."
            n952 = local read "CS.Current Value"() -> (w1387:dbl[])
            n953 = Multiply(x=1000.0, y=w1387) -> (x*y=w1385:dbl[])
            n954 = local write "CS.Automode Current"(w1385) -> ()
          }
        }
        "CS.Automode 1" <- w1369
        "CS.Automode 2" <- w1369
        "CS.Automode 3" <- w1369
        "CS.Automode 0" <- w1369
        n955 = property on="CS Modes Panel" class="TabCtl (strict)"("Value"=w1365) -> ()  [unwired: 2 in, 2 out]
      }
      event "Data Logging Settings.External VI Path": Value Change {
        # "Set path for the external VI to call on TempStabilised event"
        n956 = event-data() -> ("NewVal"=w1392:path)  [unwired: 1 in, 5 out]
        n957 = vi-ref "OnTempStabilizedRef.vi"() -> (w1393:refnum<vi>)
        n958 = Open VI Reference(type specifier VI Refnum (for type only)=w1393, vi path=w1392) -> (vi reference=w1391:refnum<vi>)  [unwired: 4 in, 1 out]
        n959 = local write "_ExtVIReference"(w1391) -> ()
      }
      event "CS Settings.CS type": Value Change {
        # "Set CS type"
        n960 = event-data() -> ("NewVal"=w1395:T57)  [unwired: 1 in, 5 out]
        n961 = flat-sequence {
          tunnel: w1395 -> [w1422]
          frame #0 {
            w1407 = u8 2 ("Disabled")
            w1402 = u8 0 ("Disabled")
            w1417 = TRUE ("Visible")
            n962 = control-ref of="CS Indicators Panel"() -> (w1403:refnum<vi>)
            n963 = control-ref of="I0"() -> (w1414:refnum<vi>)
            n964 = control-ref of="I1"() -> (w1406:refnum<vi>)
            n965 = control-ref of="CS.I0"() -> (w1413:refnum<vi>)
            n966 = control-ref of="CS.I1"() -> (w1405:refnum<vi>)
            n967 = control-ref of="I2"() -> (w1401:refnum<vi>)
            n968 = control-ref of="I3"() -> (w1400:refnum<vi>)
            n969 = control-ref of="CS Mode"() -> (w1404:refnum<vi>)
            n970 = control-ref of="QCS. I0 Mapping"() -> (w1412:refnum<vi>)
            n971 = property class="TabCtl (strict)"(reference=w1403, "Disabled"=w1402) -> ()  [unwired: 1 in, 2 out]
            n972 = property class="Clust (strict)"(reference=w1414, "Disabled"=w1402) -> ()  [unwired: 1 in, 2 out]
            n973 = property class="Clust (strict)"(reference=w1406, "Disabled"=w1402) -> ()  [unwired: 1 in, 2 out]
            n974 = property class="Clust (strict)"(reference=w1401, "Disabled"=w1402) -> ()  [unwired: 1 in, 2 out]
            n975 = property class="Clust (strict)"(reference=w1400, "Disabled"=w1402) -> ()  [unwired: 1 in, 2 out]
            n976 = property class="Clust (strict)"(reference=w1413, "Disabled"=w1402) -> ()  [unwired: 1 in, 2 out]
            n977 = property class="Clust (strict)"(reference=w1405, "Disabled"=w1402) -> ()  [unwired: 1 in, 2 out]
            n978 = property class="Enum (strict)"(reference=w1412, "Disabled"=w1402) -> ()  [unwired: 1 in, 2 out]
            n979 = property class="Enum (strict)"(reference=w1404, "Disabled"=w1402) -> ()  [unwired: 1 in, 2 out]
            n980 = property on="Side Panel" class="TabCtl (strict)"() -> ("Pages"=w1396:refnum<vi>[])  [unwired: 2 in, 2 out]
            n981 = control-ref of="TCS RS232 Port"() -> (w1416:refnum<vi>)
            n982 = Index Array(array=w1396, index=1) -> (element=w1397:refnum<vi>)
            n983 = control-ref of="Toggle Gated"() -> (w1408:refnum<vi>)
            n984 = control-ref of="Toggle Gated"() -> (w1409:refnum<vi>)
            n985 = control-ref of="Toggle Gated"() -> (w1410:refnum<vi>)
            n986 = control-ref of="Toggle Gated"() -> (w1411:refnum<vi>)
            n987 = control-ref of="CS.QCS Device Nr"() -> (w1419:refnum<vi>)
            n988 = control-ref of="CS.QCS I0 Output"() -> (w1418:refnum<vi>)
            n989 = property class="Page"(reference=w1397, "PageVis"=TRUE ("Page Visible")) -> ()  [unwired: 1 in, 2 out]
            n990 = property class="Bool (strict)"(reference=w1408, "Disabled"=w1407) -> ()  [unwired: 1 in, 2 out]
            n991 = property class="Bool (strict)"(reference=w1409, "Disabled"=w1407) -> ()  [unwired: 1 in, 2 out]
            n992 = property class="Bool (strict)"(reference=w1410, "Disabled"=w1407) -> ()  [unwired: 1 in, 2 out]
            n993 = property class="Bool (strict)"(reference=w1411, "Disabled"=w1407) -> ()  [unwired: 1 in, 2 out]
            n994 = property class="DigNum (strict)"(reference=w1419, "Visible"=w1417) -> ()  [unwired: 1 in, 2 out]
            n995 = property class="Enum (strict)"(reference=w1418, "Visible"=w1417) -> ()  [unwired: 1 in, 2 out]
            n996 = property class="VISAName"(reference=w1416, "Visible"=FALSE) -> ()  [unwired: 1 in, 2 out]
          }
          frame #1 {
            n997 = case shown="\"PCS (n.a.)\"" w1422 {
              tunnel: [refnum<class "TCS.lvclass"> refnum ("TCS.lvclass") refnum<class "QCS.lvclass"> refnum ("QCS.lvclass") w1442 w1456 refnum<class "PCS.lvclass"> refnum ("PCS.lvclass")] -> w1421
              tunnel: [w1423 w1441 u16 255 ("Value") u16 255 ("Value") w1461] -> w1420
              frame "TCS" {
                w1426 = u8 2 ("Disabled")
                w1439 = u8 0 ("Disabled")
                n998 = control-ref of="TCS RS232 Port"() -> (w1429:refnum<vi>)
                n999 = control-ref of="Toggle Gated"() -> (w1438:refnum<vi>)
                n1000 = control-ref of="Toggle Gated"() -> (w1437:refnum<vi>)
                n1001 = control-ref of="Toggle Gated"() -> (w1436:refnum<vi>)
                n1002 = control-ref of="Toggle Gated"() -> (w1435:refnum<vi>)
                n1003 = control-ref of="CS.QCS Device Nr"() -> (w1431:refnum<vi>)
                n1004 = control-ref of="I0"() -> (w1434:refnum<vi>)
                n1005 = control-ref of="CS.I0"() -> (w1427:refnum<vi>)
                n1006 = control-ref of="QCS. I0 Mapping"() -> (w1428:refnum<vi>)
                n1007 = property class="Bool (strict)"(reference=w1438, "Disabled"=w1439) -> ()  [unwired: 1 in, 2 out]
                n1008 = property class="Bool (strict)"(reference=w1437, "Disabled"=w1439) -> ()  [unwired: 1 in, 2 out]
                n1009 = property class="Bool (strict)"(reference=w1436, "Disabled"=w1439) -> ()  [unwired: 1 in, 2 out]
                n1010 = property class="Bool (strict)"(reference=w1435, "Disabled"=w1439) -> ()  [unwired: 1 in, 2 out]
                n1011 = property class="Clust (strict)"(reference=w1427, "Disabled"=w1426) -> ()  [unwired: 1 in, 2 out]
                n1012 = property class="Clust (strict)"(reference=w1434, "Disabled"=u8 2) -> ()  [unwired: 1 in, 2 out]
                n1013 = property class="DigNum (strict)"(reference=w1431, "Visible"=FALSE) -> ()  [unwired: 1 in, 2 out]
                n1014 = property class="VISAName"(reference=w1429, "Visible"=TRUE) -> ()  [unwired: 1 in, 2 out]
                n1015 = property class="Enum (strict)"(reference=w1428, "Disabled"=w1426) -> ()  [unwired: 1 in, 2 out]
                n1016 = property on="TCS RS232 Port" class="VISAName"() -> ("Value"=w1424:refnum<visa-resource-name>)  [unwired: 2 in, 2 out]
                n1017 = call "VISA to RS232 Port Nr.vi"("VISA Resource Name"=w1424) -> ("Port Number"=w1423:u8)  [unwired: 1 in]
              }
              frame "QCS v1" {
                n1018 = property on="CS.QCS Device Nr" class="DigNum (strict)"() -> ("Value"=w1441:u16)  [unwired: 2 in, 2 out]
              }
              frame "CS Emulation" {
                w1442 = refnum<class "CS Emulation.lvclass"> refnum  # CS Emulation.lvclass
                n1019 = control-ref of="CS.QCS Device Nr"() -> (w1445:refnum<vi>)
                n1020 = property class="DigNum (strict)"(reference=w1445, "Visible"=FALSE) -> ()  [unwired: 1 in, 2 out]
              }
              frame "Disabled", Default {
                w1446 = u8 2 ("Disabled")
                w1456 = refnum<class "CS Emulation.lvclass"> refnum  # CS Emulation.lvclass
                n1021 = control-ref of="CS Indicators Panel"() -> (w1455:refnum<vi>)
                n1022 = control-ref of="I0"() -> (w1450:refnum<vi>)
                n1023 = control-ref of="I1"() -> (w1449:refnum<vi>)
                n1024 = control-ref of="I2"() -> (w1448:refnum<vi>)
                n1025 = control-ref of="I3"() -> (w1447:refnum<vi>)
                n1026 = control-ref of="CS.QCS Device Nr"() -> (w1459:refnum<vi>)
                n1027 = property class="DigNum (strict)"(reference=w1459, "Visible"=FALSE) -> ()  [unwired: 1 in, 2 out]
                n1028 = property class="Clust (strict)"(reference=w1450, "Disabled"=w1446) -> ()  [unwired: 1 in, 2 out]
                n1029 = property class="Clust (strict)"(reference=w1449, "Disabled"=w1446) -> ()  [unwired: 1 in, 2 out]
                n1030 = property class="Clust (strict)"(reference=w1448, "Disabled"=w1446) -> ()  [unwired: 1 in, 2 out]
                n1031 = property class="Clust (strict)"(reference=w1447, "Disabled"=w1446) -> ()  [unwired: 1 in, 2 out]
                n1032 = property class="TabCtl (strict)"(reference=w1455, "Disabled"=w1446) -> ()  [unwired: 1 in, 2 out]
                n1033 = property on="Side Panel" class="TabCtl (strict)"() -> ("Pages"=w1454:refnum<vi>[])  [unwired: 2 in, 2 out]
                n1034 = Index Array(array=w1454, index=1) -> (element=w1453:refnum<vi>)
                n1035 = property class="Page"(reference=w1453, "PageVis"=FALSE ("Page Visible")) -> ()  [unwired: 1 in, 2 out]
              }
              frame "PCS (n.a.)" {
                w1462 = u8 2 ("Disabled")
                n1036 = control-ref of="I0"() -> (w1468:refnum<vi>)
                n1037 = control-ref of="I1"() -> (w1467:refnum<vi>)
                n1038 = control-ref of="CS.I0"() -> (w1466:refnum<vi>)
                n1039 = control-ref of="CS.I1"() -> (w1465:refnum<vi>)
                n1040 = control-ref of="CS Mode"() -> (w1464:refnum<vi>)
                n1041 = control-ref of="QCS. I0 Mapping"() -> (w1463:refnum<vi>)
                n1042 = property class="Clust (strict)"(reference=w1466, "Disabled"=w1462) -> ()  [unwired: 1 in, 2 out]
                n1043 = property class="Clust (strict)"(reference=w1465, "Disabled"=w1462) -> ()  [unwired: 1 in, 2 out]
                n1044 = property class="Clust (strict)"(reference=w1468, "Disabled"=w1462) -> ()  [unwired: 1 in, 2 out]
                n1045 = property class="Clust (strict)"(reference=w1467, "Disabled"=w1462) -> ()  [unwired: 1 in, 2 out]
                n1046 = property class="Enum (strict)"(reference=w1464, "Disabled"=w1462) -> ()  [unwired: 1 in, 2 out]
                n1047 = property class="Enum (strict)"(reference=w1463, "Disabled"=w1462) -> ()  [unwired: 1 in, 2 out]
                n1048 = property on="CS.QCS Device Nr" class="DigNum (strict)"() -> ("Value"=w1461:u16)  [unwired: 2 in, 2 out]
              }
            }
            "_CSClassRef" <- w1421
            n1049 = property on="_CS_Address" class="DigNum (strict)"("Value"=w1420) -> ()  [unwired: 2 in, 2 out]
          }
        }
      }
      event "CS Settings.CS.QCS Device Nr": Value Change {
        # "Set CS port"
        n1050 = event-data() -> ("NewVal"=w1470:u16)  [unwired: 1 in, 5 out]
        n1051 = property on="CS type" class="Enum (strict)"() -> ("Value"=w1471:T57)  [unwired: 2 in, 2 out]
        n1052 = case shown="Default" w1471 {
          tunnel: w1470 -> [_ w1474 _]
          frame Default {
          }
          frame "QCS v1" {
            n1053 = Variant To Data(type=u32 255 ("HW Address"), Variant=w1474) -> (data=w1472:u32)  [unwired: 1 in, 1 out]
            n1054 = property on="_CS_Address" class="DigNum (strict)"("Value"=w1472) -> ()  [unwired: 2 in, 2 out]
          }
          frame "CS Emulation" {
            n1055 = property on="_CS_Address" class="DigNum (strict)"("Value"=u32 255 ("HW Address")) -> ()  [unwired: 2 in, 2 out]
          }
        }
      }
      event "CS Settings.TCS RS232 Port": Value Change {
        # "Set TCS port"
        n1056 = event-data() -> ("NewVal"=w1477:refnum<visa-resource-name>)  [unwired: 1 in, 5 out]
        n1057 = property on="CS type" class="Enum (strict)"() -> ("Value"=w1478:T57)  [unwired: 2 in, 2 out]
        n1058 = case shown="\"TCS\"" w1478 {
          tunnel: w1477 -> [w1481 _]
          frame "TCS" {
            n1059 = Type Cast(type=refnum<visa-resource-name> refnum ("Value"), x=w1481) -> (*(type *) &x=w1480:refnum<visa-resource-name>)
            n1060 = call "VISA to RS232 Port Nr.vi"("VISA Resource Name"=w1480) -> ("Port Number"=w1482:u8)  [unwired: 1 in]
            n1061 = property on="_CS_Address" class="DigNum (strict)"("Value"=w1482) -> ()  [unwired: 2 in, 2 out]
          }
          frame Default {
          }
        }
      }
      event "Load Data": Value Change {
        # "Load data from log files"
        n1062 = event-data() -> ()  [unwired: 1 in, 6 out]
        n1063 = property on="Log Files Folder" class="Path"() -> ("Value"=w1486:path)  [unwired: 2 in, 2 out]
        n1064 = call "File Dialog4"("start path"=w1486) -> ("selected paths"=w1485:path[], "cancelled"=w1484:bool)  [unwired: 11 in, 2 out]
        n1065 = case shown="False" w1484 {
          tunnel: w1485 -> [w1500 _]
          frame False {
            n1066 = property on="Bridge Type" class="Enum (strict)"() -> ("Value"=w1490:T61)  [unwired: 2 in, 2 out]
            n1067 = case shown="Default" w1490 {
              tunnel: [2 ("index")] -> w1489
              tunnel: [10 ("length")] -> w1487
              tunnel: [12 ("index")] -> w1488
              frame Default {
              }
            }
            n1068 = for {
              tunnel: w1500 -> [w1524] mode=indexing
              shift-right: [w1522] -> w1497
              shift-left: string[][] [] ("all rows") -> [w1523]
              # "skip header"
              n1069 = call <vilib>:"Read From Spreadsheet File (string).vi"("file path (dialog if empty)"=w1524) -> ("all rows"=w1520:string[][])  [unwired: 6 in, 4 out]
              n1070 = Array Subset(array=w1520, index (row)=5 ("index")) -> (w1519:string[][])  [unwired: 3 in]
              n1071 = Insert Into Array(array=w1523, new element=w1519) -> (w1522:string[][])  [unwired: 2 in]
            }
            n1072 = Index Array(array=w1497, index (col)=1 ("disabled index (col)")) -> (element=w1494:string[])  [unwired: 1 in]
            n1073 = Array Subset(array=w1497, index (col)=w1489, length (col)=w1487) -> (w1496:string[][])  [unwired: 2 in]
            n1074 = Array Subset(array=w1497, index (col)=w1488, length (col)=w1487) -> (w1495:string[][])  [unwired: 2 in]
            n1075 = Transpose 2D Array(2D array=w1496) -> (transposed array=w1492:string[][])
            n1076 = Transpose 2D Array(2D array=w1495) -> (transposed array=w1491:string[][])
            n1077 = for {
              tunnel: w1492 -> [w1516] mode=indexing
              tunnel: w1491 -> [w1515] mode=indexing
              tunnel: w1494 -> [w1517]
              tunnel: [w1514] -> w1493 mode=indexing
              # "Sort data by date and remove duplicate points"
              n1078 = Fract/Exp String To Number(string=w1516) -> (number=w1511:dbl[])  [unwired: 3 in, 1 out]
              n1079 = Fract/Exp String To Number(string=w1517) -> (number=w1513:dbl[])  [unwired: 3 in, 1 out]
              n1080 = Fract/Exp String To Number(string=w1515) -> (number=w1512:dbl[])  [unwired: 3 in, 1 out]
              n1081 = call "Sort 1D Array (DBL)__ogtk.vi"("Array in"=w1513) -> ("Sorted Pointers"=w1518:i32[], "Sorted Array out"=w1506:dbl[])  [unwired: 9 in]
              n1082 = call "Reorder 1D Array2 (DBL)__ogtk.vi"("indices"=w1518, "array"=w1511) -> ("reordered array"=w1510:dbl[])  [unwired: 9 in]
              n1083 = call "Reorder 1D Array2 (DBL)__ogtk.vi"("indices"=w1518, "array"=w1512) -> ("reordered array"=w1508:dbl[])  [unwired: 9 in]
              n1084 = call "Remove Duplicates from 1D Array (DBL)__ogtk.vi"("Input Array"=w1510) -> ("Output Array"=w1509:dbl[], "indices of removed elements"=w1504:i32[])
              n1085 = call "Delete Elements from 1D Array (DBL)__ogtk.vi"("indices"=w1504, "array"=w1508) -> ("array w/ subset deleted"=w1507:dbl[])  [unwired: 8 in, 1 out]
              n1086 = call "Delete Elements from 1D Array (DBL)__ogtk.vi"("indices"=w1504, "array"=w1506) -> ("array w/ subset deleted"=w1505:dbl[])  [unwired: 8 in, 1 out]
              n1087 = Bundle("Output Array"=w1509, "array w/ subset deleted"=w1507, "array w/ subset deleted"=w1505) -> (w1514:T72)  [unwired: 1 in]
            }
            n1088 = local write "Data Array"(w1493) -> ()
          }
          frame True {
          }
        }
      }
      event "Save Data 2": Value Change {
        # "Load data from log files"
        n1089 = event-data() -> ()  [unwired: 1 in, 6 out]
        n1090 = property on="Log Files Folder" class="Path"() -> ("Value"=w1530:path)  [unwired: 2 in, 2 out]
        n1091 = call "File Dialog"("start path"=w1530, "pattern (all files)"="*.dat", "pattern label"="Log files") -> ("selected path"=w1528:path, "cancelled"=w1529:bool)  [unwired: 9 in, 2 out]
        n1092 = case shown="False" w1529 {
          tunnel: w1528 -> [w1535 _]
          frame False {
            (unwired) 30 ("dimension size")
            n1093 = local read "Data Array"() -> (w1536:T28)
            n1094 = for {
              tunnel: w1536 -> [w1549] mode=indexing
              tunnel: [w1540] -> w1534 mode=indexing
              shift-right: [w1538] -> w1532
              shift-left: string[][] [] -> [w1539]
              n1095 = Unbundle By Name(w1549) -> ("Time"=w1546:dbl[], "R"=w1545:dbl[], "T"=w1541:dbl[])
              n1096 = property on="Data Logging Settings" class="Clust (strict)"() -> ("Value"=w1548:T37)  [unwired: 2 in, 2 out]
              n1097 = Unbundle By Name(w1548) -> ("Date Format"=w1547:string)
              n1098 = Array Size(array=w1541) -> (size(s)=w1540:i32)
              n1099 = for {
                tunnel: w1547 -> [w1552]
                tunnel: [w1551] -> w1544 mode=indexing
                tunnel: w1546 -> [w1550] mode=indexing
                n1100 = Format Date/Time String(time format string (%c)=w1552, seconds (now)=w1550) -> (date/time string=w1551:string)  [unwired: 1 in]
              }
              n1101 = Number To Fractional String(number=w1545) -> (F-format string=w1543:string[])  [unwired: 3 in]
              n1102 = Number To Fractional String(number=w1541) -> (F-format string=w1542:string[])  [unwired: 3 in]
              n1103 = Build Array(w1544, w1543, w1542) -> (w1537:string[][])
              n1104 = Build Array (concatenate)(w1539, w1537) -> (w1538:string[][])
            }
            n1105 = Array Max & Min(array=w1534) -> ()  [unwired: 4 out]
            n1106 = call "Write To Spreadsheet File (string) w Error.vi"("transpose? (no:F)"=TRUE, "2D data"=w1532, "file path (dialog if empty)"=w1535) -> ()  [unwired: 7 in, 2 out]
          }
          frame True {
          }
        }
      }
      event "Plot-save-screen": Value Change {
        n1107 = event-data() -> ()  [unwired: 1 in, 6 out]
        n1108 = property on="Log Files Folder" class="Path"() -> ("Value"=w1558:path)  [unwired: 2 in, 2 out]
        n1109 = call "File Dialog7"("start path"=w1558, "pattern (all files)"="*.dat", "pattern label"="Log files") -> ("selected path"=w1556:path, "cancelled"=w1557:bool)  [unwired: 9 in, 2 out]
        n1110 = case shown="False" w1557 {
          tunnel: w1556 -> [w1583 _]
          frame False {
            # "!!NOTE:This routine assumes that XY graph is \ncontrol #0 on tab page!!"
            n1111 = property on="Channels Panel" class="TabCtl (strict)"() -> ("Pages"=w1581:refnum<vi>[], "Value"=w1580:T8)  [unwired: 2 in, 2 out]
            n1112 = Index Array(array=w1581, index=w1580) -> (element=w1579:refnum<vi>)
            n1113 = property class="Page"(reference=w1579) -> ("ControlsOnPage"=w1576:refnum<vi>[])  [unwired: 1 in, 2 out]
            n1114 = Index Array(array=w1576, index=0) -> (element=w1578:refnum<vi>)
            n1115 = control-ref of="R-Plot 0"() -> (w1574:refnum<vi>)
            n1116 = Type Cast(type=w1574, x=w1578) -> (*(type *) &x=w1575:refnum<vi>)
            n1117 = property class="XYGraph (strict)"(reference=w1575) -> ("Value"=w1573:cluster{dbl[], dbl[]}, "XScale.Maximum"=w1572:dbl, "XScale.Minimum"=w1571:dbl)  [unwired: 1 in, 2 out]
            n1118 = Unbundle(w1573) -> (w1570:dbl[], w1569:dbl[])
            n1119 = call "MGI Threshold 1D Array Extended.vi"("Threshold Y"=w1572, "Y Value[]"=w1570) -> ("Extended Fractional Index"=w1560:dbl)  [unwired: 1 in]
            n1120 = call "MGI Threshold 1D Array Extended.vi"("Threshold Y"=w1571, "Y Value[]"=w1570) -> ("Extended Fractional Index"=w1559:dbl)  [unwired: 1 in]
            n1121 = Subtract(x=w1560, y=w1559) -> (x-y=w1582:dbl)
            n1122 = Array Subset(array=w1570, index=w1559, length=w1582) -> (w1564:dbl[])
            n1123 = Array Subset(array=w1569, index=w1559, length=w1582) -> (w1562:dbl[])
            n1124 = property on="Data Logging Settings" class="Clust (strict)"() -> ("Value"=w1566:T37)  [unwired: 2 in, 2 out]
            n1125 = Unbundle By Name(w1566) -> ("Date Format"=w1565:string)
            n1126 = Number To Fractional String(number=w1562) -> (F-format string=w1561:string[])  [unwired: 3 in]
            n1127 = for {
              tunnel: w1565 -> [w1586]
              tunnel: [w1585] -> w1563 mode=indexing
              tunnel: w1564 -> [w1584] mode=indexing
              n1128 = Format Date/Time String(time format string (%c)=w1586, seconds (now)=w1584) -> (date/time string=w1585:string)  [unwired: 1 in]
            }
            n1129 = Build Array(w1563, w1561) -> (w1568:string[][])
            n1130 = call <vilib>:"Write To Spreadsheet File (string).vi"("transpose? (no:F)"=TRUE, "2D data"=w1568, "file path (dialog if empty)"=w1583) -> ()  [unwired: 5 in, 1 out]
          }
          frame True {
          }
        }
      }
      event "Plot-Save All": Value Change {
        n1131 = event-data() -> ()  [unwired: 1 in, 6 out]
        n1132 = property on="Log Files Folder" class="Path"() -> ("Value"=w1592:path)  [unwired: 2 in, 2 out]
        n1133 = call "File Dialog8"("start path"=w1592, "pattern (all files)"="*.dat", "pattern label"="Log files") -> ("selected path"=w1590:path, "cancelled"=w1591:bool)  [unwired: 9 in, 2 out]
        n1134 = case shown="False" w1591 {
          tunnel: w1590 -> [w1610 _]
          frame False {
            # "!!NOTE:This routine assumes that XY graph is \ncontrol #0 on tab page!!"
            n1135 = property on="Channels Panel" class="TabCtl (strict)"() -> ("Pages"=w1609:refnum<vi>[], "Value"=w1608:T8)  [unwired: 2 in, 2 out]
            n1136 = Index Array(array=w1609, index=w1608) -> (element=w1607:refnum<vi>)
            n1137 = property class="Page"(reference=w1607) -> ("ControlsOnPage"=w1604:refnum<vi>[])  [unwired: 1 in, 2 out]
            n1138 = Index Array(array=w1604, index=0) -> (element=w1606:refnum<vi>)
            n1139 = control-ref of="R-Plot 0"() -> (w1602:refnum<vi>)
            n1140 = Type Cast(type=w1602, x=w1606) -> (*(type *) &x=w1603:refnum<vi>)
            n1141 = property class="XYGraph (strict)"(reference=w1603) -> ("Value"=w1601:cluster{dbl[], dbl[]})  [unwired: 1 in, 2 out]
            n1142 = Unbundle(w1601) -> (w1594:dbl[], w1593:dbl[])
            n1143 = property on="Data Logging Settings" class="Clust (strict)"() -> ("Value"=w1598:T37)  [unwired: 2 in, 2 out]
            n1144 = Unbundle By Name(w1598) -> ("Date Format"=w1597:string)
            n1145 = Number To Fractional String(number=w1593) -> (F-format string=w1595:string[])  [unwired: 3 in]
            n1146 = for {
              tunnel: w1597 -> [w1613]
              tunnel: [w1612] -> w1596 mode=indexing
              tunnel: w1594 -> [w1611] mode=indexing
              n1147 = Format Date/Time String(time format string (%c)=w1613, seconds (now)=w1611) -> (date/time string=w1612:string)  [unwired: 1 in]
            }
            n1148 = Build Array(w1596, w1595) -> (w1600:string[][])
            n1149 = call <vilib>:"Write To Spreadsheet File (string).vi"("transpose? (no:F)"=TRUE, "2D data"=w1600, "file path (dialog if empty)"=w1610) -> ()  [unwired: 5 in, 1 out]
          }
          frame True {
          }
        }
      }
      event "_CurrentsChanged": Value Change {
        # "New values for currents were entered by user/automode-> write new data to CS"
        n1150 = event-data() -> ()  [unwired: 1 in, 6 out]
        n1151 = local read "_CSClassRef"() -> (w1619:refnum<class "CS.lvclass">)
        n1152 = property on="CS status" class="Clust (strict)"() -> ("Value"=w1616:errorcluster)  [unwired: 2 in, 2 out]
        n1153 = call-dynamic "Read.vi"("CS in"=w1619, "error in (no error)"=w1616, "Optional"=TRUE ("Unused")) -> ("CS out"=w1618:refnum<class "CS.lvclass">, "error out"=w1615:errorcluster)  [unwired: 11 in, 4 out]
        n1154 = local write "_CSClassRef"(w1618) -> ()
        n1155 = property on="CS status" class="Clust (strict)"("Value"=w1615) -> ()  [unwired: 2 in, 2 out]
      }
      event "CS.QCS I0 Output": Value Change {
        # "Switch QCS channel 0 to aux output"
        n1156 = event-data() -> ("OldVal"=w1627:T38, "NewVal"=w1622:T38)  [unwired: 1 in, 4 out]
        n1157 = To Long Integer(number=w1622) -> (32bit integer=→"QCS. I0 Mapping":i32)
        n1158 = local read "_CSClassRef"() -> (w1625:refnum<class "CS.lvclass">)
        n1159 = property on="CS status" class="Clust (strict)"() -> ("Value"=w1626:errorcluster)  [unwired: 2 in, 2 out]
        n1160 = call-dynamic "Switch Output Channel.vi"("error in (no error)"=w1626, "New Channel"=w1622, "Old Channel"=w1627, "CS in"=w1625) -> ("error out"=w1623:errorcluster, "CS out"=w1624:refnum<class "CS.lvclass">)  [unwired: 6 in]
        n1161 = local write "_CSClassRef"(w1624) -> ()
        n1162 = property on="CS status" class="Clust (strict)"("Value"=w1623) -> ()  [unwired: 2 in, 2 out]
      }
      event "T Sweep.Start": Value Change {
        # "Setup and Start Current/Temperature sweep for CS channel 3"
        n1163 = event-data() -> ("CtlRef"=w1629:refnum<vi>, "NewVal"=w1630:bool)  [unwired: 1 in, 4 out]
        n1164 = case shown="False" w1630 {
          tunnel: w1629 -> [w1631 w1634]
          frame False {
            n1165 = property class="Bool (strict)"(reference=w1631, "Caption.Text"="Start") -> ()  [unwired: 1 in, 2 out]
          }
          frame True {
            n1166 = property on="Start value" class="DigNum (strict)"() -> ("Value"=w1635:dbl)  [unwired: 2 in, 2 out]
            n1167 = property class="Bool (strict)"(reference=w1634, "Caption.Text"="Stop") -> ()  [unwired: 1 in, 2 out]
            n1168 = property on="Current" class="DigNum (strict)"("Val(Sgnl)"=w1635) -> ()  [unwired: 2 in, 2 out]
          }
        }
      }
      event "T Sweep.I_next": Value Change {
        # "Go to next step in Current/Temperature sweep for CS channel 3"
        n1169 = event-data() -> ()  [unwired: 1 in, 6 out]
        n1170 = property on="I_next" class="Bool (strict)"("Value"=FALSE) -> ()  [unwired: 2 in, 2 out]
        n1171 = call "Current Time(double).vi"() -> ("Current Time (double)"=w1637:dbl)  [unwired: 6 in, 1 out]
        n1172 = local write "_TimeOld"(w1637) -> ()
        n1173 = property on="Current" class="DigNum (strict)"() -> ("Value"=w1638:dbl)  [unwired: 2 in, 2 out]
        n1174 = property on="Step" class="DigNum (strict)"() -> ("Value"=w1643:dbl)  [unwired: 2 in, 2 out]
        n1175 = Add(x=w1638, y=w1643) -> (x+y=w1642:dbl)
        n1176 = property on="End value" class="DigNum (strict)"() -> ("Value"=w1641:dbl)  [unwired: 2 in, 2 out]
        n1177 = property on="Start value" class="DigNum (strict)"() -> ("Value"=w1640:dbl)  [unwired: 2 in, 2 out]
        n1178 = In Range and Coerce(upper limit=w1641, x=w1642, lower limit=w1640) -> (coerced(x)=w1639:dbl)  [unwired: 1 out]
        n1179 = property on="Current" class="DigNum (strict)"("Val(Sgnl)"=w1639) -> ()  [unwired: 2 in, 2 out]
      }
      event "T Sweep.I_prev": Value Change {
        # "Go to previous step in Current/Temperature sweep for CS channel 3"
        n1180 = event-data() -> ()  [unwired: 1 in, 6 out]
        n1181 = call "Current Time(double).vi"() -> ("Current Time (double)"=w1646:dbl)  [unwired: 6 in, 1 out]
        n1182 = property on="I_prev" class="Bool (strict)"("Value"=FALSE) -> ()  [unwired: 2 in, 2 out]
        n1183 = local write "_TimeOld"(w1646) -> ()
        n1184 = property on="Current" class="DigNum (strict)"() -> ("Value"=w1648:dbl)  [unwired: 2 in, 2 out]
        n1185 = property on="Step" class="DigNum (strict)"() -> ("Value"=w1653:dbl)  [unwired: 2 in, 2 out]
        n1186 = Subtract(x=w1648, y=w1653) -> (x-y=w1652:dbl)
        n1187 = property on="End value" class="DigNum (strict)"() -> ("Value"=w1651:dbl)  [unwired: 2 in, 2 out]
        n1188 = property on="Start value" class="DigNum (strict)"() -> ("Value"=w1650:dbl)  [unwired: 2 in, 2 out]
        n1189 = In Range and Coerce(upper limit=w1651, x=w1652, lower limit=w1650) -> (coerced(x)=w1649:dbl)  [unwired: 1 out]
        n1190 = property on="Current" class="DigNum (strict)"("Val(Sgnl)"=w1649) -> ()  [unwired: 2 in, 2 out]
      }
      event User Event {
        # "Reset the PID loop"
        n1191 = event-data() -> ()  [unwired: 1 in, 5 out]
        n1192 = local write "CS.Mode1.PID Error"(0.0 ("T_error")) -> ()
      }
      event "Minimize UI 1", "Minimize UI 2": Value Change {
        (unwired) 29 ("Splitter Position")
        (unwired) 534 ("Numeric 2")
        # "Shrink/restore the program window"
        # "726"
        # "222"
        # "1243"
        # "816"
        n1193 = event-data() -> ()  [unwired: 1 in, 6 out]
        n1194 = case shown="True" "Minimize UI 1" {
          tunnel: "Minimize UI 2" -> [_ w1684]
          frame True {
            (unwired) T54."Disabled" ("Value")
            n1195 = property on="CS type" class="Enum (strict)"() -> ("Value"=w1670:T57)  [unwired: 2 in, 2 out]
            n1196 = property on="Bridge Type" class="Enum (strict)"() -> ("Value"=w1665:T61)  [unwired: 2 in, 2 out]
            n1197 = Equal?(x=w1665, y=T54."Disabled" ("Value")) -> (x = y?=w1663:bool)
            n1198 = Equal?(x=w1670, y=T57."Disabled" ("Value")) -> (x = y?=w1669:bool)
            n1199 = property on="Data History/RT Settings" class="TabCtl (strict)"("Value"=enum32{"History", "Settings"}."History" ("Data History")) -> ()  [unwired: 2 in, 2 out]
            n1200 = Exclusive Or(1:w1663, 2:w1669) -> (0:w1662:bool)
            n1201 = property on="Mode Buttons" class="RadioBtnsControl (strict)"("Disabled"=u8 2, "Val(Sgnl)"=T56."No Selection" ("Value (Signaling)")) -> ()  [unwired: 2 in, 2 out]
            n1202 = property class="VI"() -> ("Front Panel.PanelBounds"=w1672:T73)  [unwired: 2 in, 2 out]
            n1203 = Select(t=i16 105 ("y"), s=w1662, f=i16 169 ("y")) -> (s? t:f=w1666:i16)
            n1204 = Unbundle By Name(w1672) -> ("Left"=w1678:i16, "Top"=w1675:i16)
            n1205 = property on="Splitter 3" class="Splitter"("Position"=29 ("Splitter Position")) -> (error out=w1664:errorcluster)  [unwired: 2 in, 1 out]
            n1206 = Add(x=i16 806 ("right"), y=w1678) -> (x+y=w1677:i16)
            n1207 = Add(x=w1675, y=w1666) -> (x+y=w1674:i16)
            n1208 = Bundle By Name(cluster=w1672, "Right"=w1677, "Bottom"=w1674) -> (w1679:T73)
            n1209 = case shown="True" w1663 {
              tunnel: w1664 -> [_ w1682]
              frame False {
              }
              frame True {
                n1210 = property on="Splitter 4" class="Splitter"(error in=w1682, "Position"=32 ("Splitter Position")) -> ()  [unwired: 1 in, 2 out]
              }
            }
            n1211 = property class="VI"("Front Panel.PanelBounds"=w1679) -> ()  [unwired: 2 in, 2 out]
          }
          frame False {
            n1212 = property class="VI"() -> ("Front Panel.PanelBounds"=w1691:T73)  [unwired: 2 in, 2 out]
            n1213 = property on="Channels Panel" class="TabCtl (strict)"() -> ("Value"=w1699:T8)  [unwired: 2 in, 2 out]
            n1214 = Unbundle By Name(w1691) -> ("Left"=w1697:i16, "Top"=w1695:i16)
            n1215 = property on="Channels Panel" class="TabCtl (strict)"("Val(Sgnl)"=w1699) -> ()  [unwired: 2 in, 2 out]
            n1216 = Select(t=i16 806 ("right"), s=w1684, f=i16 1206 ("right")) -> (s? t:f=w1688:i16)
            n1217 = Add(x=w1688, y=w1697) -> (x+y=w1696:i16)
            n1218 = Add(x=w1695, y=i16 702) -> (x+y=w1693:i16)
            n1219 = Bundle By Name(cluster=w1691, "Right"=w1696, "Bottom"=w1693) -> (w1698:T73)
            n1220 = property on="Mode Buttons" class="RadioBtnsControl (strict)"("Disabled"=u8 0) -> ()  [unwired: 2 in, 2 out]
            n1221 = property class="VI"("Front Panel.PanelBounds"=w1698) -> (error out=w1685:errorcluster)  [unwired: 2 in, 1 out]
            n1222 = property on="Splitter 3" class="Splitter"(error in=w1685, "Position"=559 ("Splitter Position")) -> (error out=w1689:errorcluster)  [unwired: 1 in, 1 out]
            n1223 = property on="Splitter 4" class="Splitter"(error in=w1689, "Position"=635 ("Splitter Position")) -> ()  [unwired: 1 in, 2 out]
          }
        }
        n1224 = property on="Splitter 2" class="Splitter"("Position"=805 ("Splitter Position")) -> ()  [unwired: 2 in, 2 out]
      }
      event "Copy to Clipboard": Value Change {
        # "Copy current values to the clipboard"
        n1225 = event-data() -> ()  [unwired: 1 in, 6 out]
        n1226 = property on="_ScanData" class="Arr (strict)"() -> ("Value"=w1705:dbl[])  [unwired: 2 in, 2 out]
        n1227 = property on="T Array" class="Arr (strict)"() -> ("Value"=w1704:dbl[])  [unwired: 2 in, 2 out]
        n1228 = Build Array(w1705, w1704) -> (w1703:dbl[][])
        n1229 = Transpose 2D Array(2D array=w1703) -> (transposed array=w1702:dbl[][])
        n1230 = Array To Spreadsheet String(delimiter (Tab)="\t", array=w1702, 3:"%.4g" ("format string")) -> (spreadsheet string=w1708:string)
        n1231 = invoke class="App" method="Clipboard.Write"("Param 0"=w1708) -> ()  [unwired: 3 in, 4 out]
      }
      event "Show PID graph?": Value Change {
        # "Display plots with the PID parameters vs time for debugging"
        n1232 = event-data() -> ("NewVal"=w1710:bool)  [unwired: 1 in, 5 out]
        n1233 = property on="Channels Panel" class="TabCtl (strict)"() -> ("Pages"=w1713:refnum<vi>[])  [unwired: 2 in, 2 out]
        n1234 = Reverse 1D Array(array=w1713) -> (reversed array=w1712:refnum<vi>[])
        n1235 = Index Array(array=w1712) -> (element=w1711:refnum<vi>)  [unwired: 1 in]
        n1236 = property class="Page"(reference=w1711, "PageVis"=w1710) -> ()  [unwired: 1 in, 2 out]
      }
      event "I0.uA", "I1.uA", "I2.uA", "I3.uA": Mouse Up {
        # "Show curent edit filed on double clicking the current indicator. Set the field to the actual current value."
        n1237 = event-data() -> ("Mods.Double Click"=w1716:bool, "CtlRef"=w1715:refnum<vi>)  [unwired: 1 in, 5 out]
        n1238 = case shown="True" w1716 {
          tunnel: w1715 -> [_ w1727]
          frame False {
          }
          frame True {
            w1723 = TRUE ("Visible")
            n1239 = property class="Str"(reference=w1727) -> ("Owner"=w1726:refnum<vi>)  [unwired: 1 in, 2 out]
            n1240 = control-ref of="uA 0"() -> (w1733:refnum<vi>)
            n1241 = control-ref of="uA 1"() -> (w1736:refnum<vi>)
            n1242 = control-ref of="uA 2"() -> (w1735:refnum<vi>)
            n1243 = control-ref of="uA 3"() -> (w1734:refnum<vi>)
            n1244 = control-ref of="I0"() -> (w1724:refnum<vi>)
            n1245 = control-ref of="I1"() -> (w1730:refnum<vi>)
            n1246 = control-ref of="I2"() -> (w1729:refnum<vi>)
            n1247 = control-ref of="I3"() -> (w1722:refnum<vi>)
            n1248 = property on="CS.Current Value" class="Arr (strict)"() -> ("Value"=w1721:dbl[])  [unwired: 2 in, 2 out]
            n1249 = Type Cast(type=w1722, x=w1726) -> (*(type *) &x=w1725:refnum<vi>)
            n1250 = Build Array(w1733, w1736, w1735, w1734) -> (w1732:refnum<vi>[])
            n1251 = Build Array(w1724, w1730, w1729, w1722) -> (w1728:refnum<vi>[])
            n1252 = Search 1D Array(1D array=w1728, element=w1725) -> (index of element=w1720:i32)  [unwired: 1 in]
            n1253 = Index Array(array=w1721, index=w1720) -> (element=w1719:dbl)
            n1254 = Index Array(array=w1732, index=w1720) -> (element=w1731:refnum<vi>)
            n1255 = Multiply(x=1000.0, y=w1719) -> (x*y=w1718:dbl)
            n1256 = property on="Property Node" class="DigNum (strict)"(reference=w1731, "Value"=w1718, "Visible"=w1723, "Key Focus"=w1723) -> ()  [unwired: 1 in, 2 out]
          }
        }
      }
      event "I0.current flows", "I1.current flows", "I2.current flows", "I3.current flows": Mouse Up {
        # "Toggle the current channel by double clickin on the \"On\" led in the current indicator."
        n1257 = event-data() -> ("CtlRef"=w1738:refnum<vi>, "Mods.Double Click"=w1739:bool)  [unwired: 1 in, 5 out]
        n1258 = case shown="True" w1739 {
          tunnel: w1738 -> [_ w1748]
          frame False {
          }
          frame True {
            n1259 = control-ref of="current flows"() -> (w1753:refnum<vi>)
            n1260 = control-ref of="current flows"() -> (w1752:refnum<vi>)
            n1261 = control-ref of="current flows"() -> (w1751:refnum<vi>)
            n1262 = control-ref of="current flows"() -> (w1750:refnum<vi>)
            n1263 = control-ref of="Toggle ON/OFF"() -> (w1747:refnum<vi>)
            n1264 = control-ref of="Toggle ON/OFF"() -> (w1745:refnum<vi>)
            n1265 = control-ref of="Toggle ON/OFF"() -> (w1744:refnum<vi>)
            n1266 = control-ref of="Toggle ON/OFF"() -> (w1746:refnum<vi>)
            n1267 = Build Array(w1753, w1752, w1751, w1750) -> (w1749:refnum<vi>[])
            n1268 = Build Array(w1747, w1745, w1744, w1746) -> (w1743:refnum<vi>[])
            n1269 = Search 1D Array(1D array=w1749, element=w1748) -> (index of element=w1742:i32)  [unwired: 1 in]
            n1270 = Index Array(array=w1743, index=w1742) -> (element=w1741:refnum<vi>)
            n1271 = property class="Bool (strict)"(reference=w1741, "Val(Sgnl)"=TRUE ("Value (Signaling)")) -> ()  [unwired: 1 in, 2 out]
          }
        }
      }
      event "uA 0", "uA 1", "uA 2", "uA 3": Value Change {
        w1756 = refnum<vi> refnum  # Numeric
        w1760 = refnum<vi> refnum  # Enum
        # "User has entered the current by double clicking on the current indicators at the bottom. \nSet range to \"Auto\" and interpret the entered value as [uA]"
        # "!!NOTE:This routine assumes that Current and Range are controls #2 & #3 in current control cluster"
        n1272 = event-data() -> ("CtlRef"=w1768:refnum<vi>, "NewVal"=w1755:u32)  [unwired: 1 in, 4 out]
        n1273 = control-ref of="CS.I0"() -> (w1777:refnum<vi>)
        n1274 = control-ref of="CS.I1"() -> (w1775:refnum<vi>)
        n1275 = control-ref of="CS.I2"() -> (w1776:refnum<vi>)
        n1276 = control-ref of="CS.I3"() -> (w1778:refnum<vi>)
        n1277 = control-ref of="uA 0"() -> (w1770:refnum<vi>)
        n1278 = control-ref of="uA 1"() -> (w1773:refnum<vi>)
        n1279 = control-ref of="uA 2"() -> (w1772:refnum<vi>)
        n1280 = control-ref of="uA 3"() -> (w1771:refnum<vi>)
        n1281 = Build Array(w1777, w1775, w1776, w1778) -> (w1774:refnum<vi>[])
        n1282 = Build Array(w1770, w1773, w1772, w1771) -> (w1769:refnum<vi>[])
        n1283 = Search 1D Array(1D array=w1769, element=w1768) -> (index of element=w1767:i32)  [unwired: 1 in]
        n1284 = Index Array(array=w1774, index=w1767) -> (element=w1766:refnum<vi>)
        n1285 = property class="Clust (strict)"(reference=w1766) -> ("Controls[]"=w1765:refnum<vi>[])  [unwired: 1 in, 2 out]
        n1286 = Index Array(array=w1765, index #1=3 ("index"), index #2=2 ("index")) -> (element #1=w1762:refnum<vi>, element #2=w1758:refnum<vi>)
        n1287 = Type Cast(type=w1756, x=w1758) -> (*(type *) &x=w1757:refnum<vi>)
        n1288 = Type Cast(type=w1760, x=w1762) -> (*(type *) &x=w1761:refnum<vi>)
        n1289 = property on="Property Node" class="Num"(reference=w1757, "Value"=w1755) -> ()  [unwired: 1 in, 2 out]
        n1290 = property on="Property Node" class="Enum"(reference=w1761, "Value"=T58."Auto") -> ()  [unwired: 1 in, 2 out]
      }
      event "_AVSRanges": Value Change {
        # "If user has changed the exitation, update the AVS bridge settings."
        n1291 = event-data() -> ("NewVal"=w1781:T29)  [unwired: 1 in, 5 out]
        n1292 = property on="AVS Exc&Ranges" class="Clust (strict)"() -> ("Value"=w1780:T15)  [unwired: 2 in, 2 out]
        n1293 = call "Combine Excitation&Range.vi"("Ranges"=w1781, "Exc&Ranges In"=w1780) -> ("Exc&Ranges Out"=w1782:T74)
        n1294 = property on="AVS Exc&Ranges" class="Clust (strict)"("Value"=w1782) -> ()  [unwired: 2 in, 2 out]
      }
      event Panel Close? {
        # "Ask for confirmation is user is trying to close the program"
        n1295 = event-data() -> ()  [unwired: 1 in, 4 out]
        n1296 = Two Button Dialog(message="Are you sure you want to quit the program?") -> (T button?=w1785:bool)  [unwired: 2 in]
        n1297 = Not(x=w1785) -> (.not. x?=w1786:bool)
        n1298 = event-data("Discard?"=w1786) -> ()  [unwired: 1 in, 1 out]
      }
      event "Save config": Mouse Up {
        # "Save parameters to the configuration file"
        n1299 = event-data() -> ()  [unwired: 1 in, 8 out]
        n1300 = control-ref of="CS Cannel Names"() -> (w1798:refnum<vi>)
        n1301 = control-ref of="AVS names"() -> (w1797:refnum<vi>)
        n1302 = control-ref of="_CurCalibrations"() -> (w1792:refnum<vi>)
        n1303 = control-ref of="CS.Mode1.PID"() -> (w1790:refnum<vi>)
        n1304 = control-ref of="CS.Mode1.Settings"() -> (w1789:refnum<vi>)
        n1305 = control-ref of="zBridge.Active Channels"() -> (w1791:refnum<vi>)
        n1306 = control-ref of="Bridge settings"() -> (w1803:refnum<vi>)
        n1307 = control-ref of="Runtime Settings"() -> (w1804:refnum<vi>)
        n1308 = control-ref of="CS Settings"() -> (w1802:refnum<vi>)
        n1309 = control-ref of="Sensor Calibrations"() -> (w1805:refnum<vi>)
        n1310 = control-ref of="PID setup"() -> (w1806:refnum<vi>)
        n1311 = control-ref of="Data Logging Settings"() -> (w1801:refnum<vi>)
        n1312 = call "File Dialog3"("start path"=path "C:/LC Data/Configuration" ("Relative path (.)"), "pattern (all files)"="*.ini") -> ("selected path"=w1793:path)  [unwired: 10 in, 3 out]
        n1313 = Build Array(w1791, w1803, w1804, w1802, w1801, w1805, w1806, w1798, w1797, w1792, w1790, w1789) -> (w1799:refnum<vi>[])
        n1314 = call "Save Load Settings to File by Ref with path.vi"("Array of Cluster References"=w1799, "Action"=enum8{"Load", "Save"}."Save", "error in (no error)"=w1796, "Configuration file"=w1793) -> ("error out"=w1795:errorcluster)  [unwired: 5 in]
      }
      event "Load config": Mouse Up {
        # "Load parameters from the configuration file"
        n1315 = event-data() -> ()  [unwired: 1 in, 8 out]
        n1316 = Unbundle By Name(w1810) -> ("UpdateCalibrations"=w1809:refnum<user-event>)
        n1317 = flat-sequence {
          tunnel: [w1835] -> w1820
          tunnel: w1816 -> [w1830]
          tunnel: [w1822] -> w1811
          tunnel: w1807 -> [w1821]
          tunnel: w1820 -> [w1850]
          tunnel: [w1850] -> w1819
          tunnel: [w1848] -> w1812
          tunnel: w1811 -> [w1848]
          tunnel: [w1855] -> w1818
          tunnel: w1819 -> [w1854]
          tunnel: [w1852] -> w1813
          tunnel: w1812 -> [w1852]
          tunnel: w1818 -> [w1861]
          tunnel: [w1861] -> w1817
          tunnel: [w1859] -> w1814
          tunnel: w1813 -> [w1859]
          tunnel: w1817 -> [w1865]
          tunnel: [w1864] -> w1815
          tunnel: w1814 -> [w1863]
          tunnel: w1809 -> [w1862]
          frame #0 {
            n1318 = control-ref of="zBridge.Active Channels"() -> (w1825:refnum<vi>)
            n1319 = control-ref of="Bridge settings"() -> (w1836:refnum<vi>)
            n1320 = control-ref of="Runtime Settings"() -> (w1832:refnum<vi>)
            n1321 = control-ref of="CS Settings"() -> (w1833:refnum<vi>)
            n1322 = control-ref of="Data Logging Settings"() -> (w1834:refnum<vi>)
            n1323 = control-ref of="PID setup"() -> (w1831:refnum<vi>)
            n1324 = control-ref of="CS Cannel Names"() -> (w1829:refnum<vi>)
            n1325 = control-ref of="AVS names"() -> (w1828:refnum<vi>)
            n1326 = control-ref of="_CurCalibrations"() -> (w1826:refnum<vi>)
            n1327 = control-ref of="CS.Mode1.PID"() -> (w1824:refnum<vi>)
            n1328 = control-ref of="CS.Mode1.Settings"() -> (w1823:refnum<vi>)
            n1329 = Build Array(w1825, w1836, w1832, w1833, w1834, w1831, w1829, w1828, w1826, w1824, w1823) -> (w1838:refnum<vi>[])
            n1330 = call "File Dialog2"("start path"=w1821, "pattern (all files)"="*.ini") -> ("selected path"=w1822:path)  [unwired: 10 in, 3 out]
            n1331 = call "Save Load Settings to File by Ref with path.vi"("Array of Cluster References"=w1838, "Action"=enum8{"Load", "Save"}."Load", "error in (no error)"=w1830, "Configuration file"=w1822) -> ("error out"=w1839:errorcluster)  [unwired: 5 in]
            n1332 = disable-structure shown="Disabled" {
              disable-tunnel: w1839 -> [w1842 w1847]
              disable-tunnel: [w1840 w1847] -> w1835
              frame Disabled {
                n1333 = property on="Bridge Type" class="Enum (strict)"(error in=w1842) -> (error out=w1843:errorcluster, "Value"=w1845:T61)  [unwired: 1 in, 1 out]
                n1334 = Equal To 0?(x=w1845) -> (x = 0?=w1846:bool)
                n1335 = property on="AVS GPIB Address" class="VISAName"(error in=w1843, "Visible"=w1846) -> (error out=w1844:errorcluster)  [unwired: 1 in, 1 out]
                n1336 = Not(x=w1846) -> (.not. x?=w1841:bool)
                n1337 = property on="AVS RS232 Port" class="VISAName"(error in=w1844, "Visible"=w1841) -> (error out=w1840:errorcluster)  [unwired: 1 in, 1 out]
              }
              frame Enabled {
              }
            }
          }
          frame #1 {
            n1338 = Wait (ms)(milliseconds to wait=250) -> ()  [unwired: 1 out]
          }
          frame #2 {
            n1339 = control-ref of="Sensor Calibrations"() -> (w1853:refnum<vi>)
            n1340 = control-ref of="_CurCalibrations"() -> (w1851:refnum<vi>)
            n1341 = control-ref of="Calibrations Folder"() -> (w1857:refnum<vi>)
            n1342 = control-ref of="Sensor 1"() -> (w1858:refnum<vi>)
            n1343 = control-ref of="_QuickConvertCal"() -> (w1856:refnum<vi>)
            n1344 = call "ReloadCalibrations.vi"("error in (no error)"=w1854, "Quick convert sensors"=w1856, "CurCalibrations"=w1851, "Calibration files path"=w1857, "Channel1 sensors"=w1858, "Channels list"=w1853) -> ("error out"=w1855:errorcluster)  [unwired: 1 in]
          }
          frame #3 {
            n1345 = Wait (ms)(milliseconds to wait=250) -> ()  [unwired: 1 out]
          }
          frame #4 {
            n1346 = disable-structure shown="Enabled" {
              disable-tunnel: w1865 -> [w1868 w1874]
              disable-tunnel: [w1867 w1876] -> w1864
              disable-tunnel: w1863 -> [w1866 _]
              disable-tunnel: w1862 -> [_ w1873]
              frame Enabled {
                (unwired) T75."HKEY_CURRENT_USER" ("root key (HKEY_LOCAL_MACHINE) 2")
                n1347 = control-ref of="Sensor Calibrations"() -> (w1871:refnum<vi>)
                n1348 = Build Array(w1871) -> (w1870:refnum<vi>[])
                n1349 = call "Save Load Settings to File by Ref with path.vi"("Array of Cluster References"=w1870, "subkey"="SOFTWARE\\Leiden Cryogenics\\TC" ("subkey 2"), "Action"=enum8{"Load", "Save"}."Load", "error in (no error)"=w1868, "Configuration file"=w1866) -> ("error out"=w1867:errorcluster)  [unwired: 4 in]
              }
              frame Disabled {
                n1350 = Generate User Event(user event=w1873, event data cluster="" ("event data"), error in=w1874) -> (error out=w1876:errorcluster)  [unwired: 1 in, 1 out]
              }
            }
          }
        }
        n1351 = Unbundle By Name(w1808) -> ("Config folder"=w1807:path)
      }
      event "zBridge settings": Value Change {
        # "Show parameters menu. (only for zBridge)"
        n1352 = event-data() -> ()  [unwired: 1 in, 6 out]
        n1353 = Unbundle By Name(w1879) -> ("zBridge dll"=w1877:path, "Config folder"=w1878:path)
        n1354 = disable-structure shown="Disabled" {
          disable-tunnel: w1878 -> [w1881 w1886]
          disable-tunnel: w1877 -> [w1880 w1885]
          frame Enabled {
            w1884 = 0 ("Page")
            n1355 = call "SetParFilePath.vi"("path"=w1881, "zDll"=w1880) -> ("error out"=w1882:errorcluster, "zDll out"=w1883:path)  [unwired: 8 in]
            n1356 = call "ParamMenu.vi"("error in (no error)"=w1882, "Subpage"=w1884, "Page"=w1884, "path in"=w1883) -> ()  [unwired: 6 in, 2 out]
          }
          frame Disabled {
            n1357 = call "SetParFilePath.vi"("path"=w1886, "zDll"=w1885) -> ("zDll out"=w1887:path)  [unwired: 8 in, 1 out]
            n1358 = call "zBridgeSettings_1page.vi"("zDll"=w1887) -> ()  [unwired: 10 in, 1 out]
          }
        }
      }
      event "Edit Calibrations": Value Change {
        # "Show calibration files editor. Works with .cal and .cal2 files only"
        n1359 = event-data() -> ("NewVal"=w1899:T11)  [unwired: 1 in, 5 out]
        n1360 = Unbundle By Name(w1891) -> ("UpdateCalibrations"=w1890:refnum<user-event>)
        n1361 = Cluster To Array(cluster=w1899) -> (array=w1898:bool[])
        n1362 = Unbundle By Name(w1889) -> ("Calibrations Folder"=w1888:path)
        n1363 = local read "_CurCalibrations"() -> (w1894:T33)
        n1364 = Search 1D Array(1D array=w1898, element=TRUE) -> (index of element=w1896:i32)  [unwired: 1 in]
        n1365 = Cluster To Array(cluster=w1894) -> (array=w1893:string[])
        n1366 = Index Array(array=w1893, index=w1896) -> (element=w1895:string)
        n1367 = call "Edit Calibration Coefficients.vi"("Calibration Name"=w1895, "Calibration folder"=w1888) -> ("Cancelled?"=w1892:bool)  [unwired: 1 out]
        n1368 = case shown="False" w1892 {
          tunnel: w1890 -> [w1900 _]
          frame False {
            n1369 = Generate User Event(user event=w1900, event data cluster="" ("event data")) -> ()  [unwired: 2 in, 2 out]
          }
          frame True {
          }
        }
      }
      event "Edit calibration": Value Change {
        # "Show calibration files editor for quick convert R->T. Works with .cal and .cal2 files only"
        n1370 = event-data() -> ()  [unwired: 1 in, 6 out]
        n1371 = Unbundle By Name(w1905) -> ("UpdateCalibrations"=w1904:refnum<user-event>)
        n1372 = Unbundle By Name(w1903) -> ("Calibrations Folder"=w1902:path)
        n1373 = property on="_QuickConvertCal" class="Ring (strict)"() -> ("Strings []"=w1908:string[], "Value"=w1909:u16)  [unwired: 2 in, 2 out]
        n1374 = Index Array(array=w1908, index=w1909) -> (element=w1907:string)
        n1375 = call "Edit Calibration Coefficients.vi"("Calibration Name"=w1907, "Calibration folder"=w1902) -> ("Cancelled?"=w1906:bool)  [unwired: 1 out]
        n1376 = case shown="False" w1906 {
          tunnel: w1904 -> [w1910 _]
          frame False {
            n1377 = Generate User Event(user event=w1910, event data cluster="" ("event data")) -> ()  [unwired: 2 in, 2 out]
          }
          frame True {
          }
        }
      }
      event "zBridge params.AVS Name 0", "zBridge params.AVS Name 1", "zBridge params.AVS Name 2", "zBridge params.AVS Name 3", "zBridge params.AVS Name 4", "zBridge params.AVS Name 5", "zBridge params.AVS Name 6", "zBridge params.AVS Name 7", "zBridge params.AVS Name 8", "zBridge params.AVS Name 9": Mouse Down {
        # "Show parameters menu for the channel by double clicking on \"Channel parameters\". (only for zBridge)"
        n1378 = event-data() -> ("CtlRef"=w1916:refnum<vi>, "Mods.Double Click"=w1915:bool, "PlatMods.Alt"=w1914:bool)  [unwired: 1 in, 5 out]
        n1379 = Unbundle By Name(w1913) -> ("zBridge dll"=w1912:path)
        n1380 = case shown="False" w1915 {
          tunnel: w1916 -> [w1920 w1925]
          tunnel: w1914 -> [_ w1924]
          tunnel: w1912 -> [w1917 w1923]
          frame True {
            n1381 = control-ref of="zBridge params"() -> (w1922:refnum<vi>)
            n1382 = property class="Clust (strict)"(reference=w1922) -> ("Controls[]"=w1921:refnum<vi>[])  [unwired: 1 in, 2 out]
            n1383 = Search 1D Array(1D array=w1921, element=w1920) -> (index of element=w1918:i32)  [unwired: 1 in]
            n1384 = call "ParamMenu.vi"("Subpage"=w1918, "Page"=0, "path in"=w1917) -> ()  [unwired: 7 in, 2 out]
          }
          frame False {
            n1385 = case shown="True" w1924 {
              tunnel: w1925 -> [_ w1927]
              tunnel: w1923 -> [_ w1926]
              frame False {
              }
              frame True {
                n1386 = disable-structure shown="Disabled" {
                  disable-tunnel: w1927 -> [w1930 w1934]
                  disable-tunnel: w1926 -> [w1928 _]
                  frame Disabled {
                    # "Show information window.\nTends to crash the acquisition!"
                    n1387 = control-ref of="zBridge params"() -> (w1932:refnum<vi>)
                    n1388 = property class="Clust (strict)"(reference=w1932) -> ("Controls[]"=w1931:refnum<vi>[])  [unwired: 1 in, 2 out]
                    n1389 = Search 1D Array(1D array=w1931, element=w1930) -> (index of element=w1929:i32)  [unwired: 1 in]
                    n1390 = call "Show Info Window.vi"("Data set number"=w1929, "zDll"=w1928) -> ()  [unwired: 8 in, 2 out]
                  }
                  frame Enabled {
                    # "Show information window."
                    n1391 = control-ref of="zBridge params"() -> (w1936:refnum<vi>)
                    n1392 = property class="Clust (strict)"(reference=w1936) -> ("Controls[]"=w1935:refnum<vi>[])  [unwired: 1 in, 2 out]
                    n1393 = Search 1D Array(1D array=w1935, element=w1934) -> (index of element=w1933:i32)  [unwired: 1 in]
                    n1394 = call "Scan Parameters Window.vi"("index"=w1933) -> ()  [unwired: 11 in]
                  }
                }
              }
            }
          }
        }
      }
      event "zBridge.Active Channels.active Channel 0", "zBridge.Active Channels.active Channel 1", "zBridge.Active Channels.active Channel 2", "zBridge.Active Channels.active Channel 3", "zBridge.Active Channels.active Channel 4", "zBridge.Active Channels.active Channel 5", "zBridge.Active Channels.active Channel 6", "zBridge.Active Channels.active Channel 7", "zBridge.Active Channels.active Channel 8", "zBridge.Active Channels.active Channel 9": Mouse Down {
        # "Switch channels On/Off by double clicking on \"Active\" LED. (only for zBridge and AVS47B)"
        n1395 = event-data() -> ("CtlRef"=w1941:refnum<vi>, "Mods.Double Click"=w1939:bool)  [unwired: 1 in, 6 out]
        n1396 = Unbundle By Name(w1938) -> ("zBridge dll"=w1937:path)
        n1397 = property on="Bridge Type" class="Enum (strict)"() -> ("Value"=w1940:T61)  [unwired: 2 in, 2 out]
        n1398 = case shown="True" w1939 {
          tunnel: w1941 -> [_ w1944]
          tunnel: w1940 -> [_ w1948]
          tunnel: w1937 -> [_ w1942]
          frame False {
          }
          frame True {
            n1399 = control-ref of="zBridge.Active Channels"() -> (w1947:refnum<vi>)
            n1400 = property class="Clust (strict)"(reference=w1947) -> ("Controls[]"=w1945:refnum<vi>[])  [unwired: 1 in, 2 out]
            n1401 = property class="Bool (strict)"(reference=w1944) -> ("Value"=w1943:bool)  [unwired: 1 in, 2 out]
            n1402 = Search 1D Array(1D array=w1945, element=w1944) -> (index of element=w1946:i32)  [unwired: 1 in]
            n1403 = case shown="\"Impedance Bridge\"" w1948 {
              tunnel: w1946 -> [_ w1953 w1955]
              tunnel: w1945 -> [_ w1952 _]
              tunnel: w1943 -> [_ w1949 _]
              tunnel: w1942 -> [_ _ w1954]
              frame Default {
              }
              frame "AVS47B (RS232 interface)" {
                n1404 = Index Array(array=w1952, index=w1953) -> (element=w1951:refnum<vi>)
                n1405 = Not(x=w1949) -> (.not. x?=w1950:bool)
                n1406 = property class="Ctl"(reference=w1951, "Value"=w1950) -> ()  [unwired: 1 in, 2 out]
              }
              frame "Impedance Bridge" {
                w1957 = Byte_Params."Active" ("Enum")
                # "Invert Active flag"
                n1407 = call "GetByteParam.vi"("ParNo"=w1957, "SetNo"=w1955, "zDll"=w1954) -> ("return type"=w1959:u8)  [unwired: 6 in, 2 out]
                n1408 = Decrement(x=w1959) -> (x-1=w1958:i8)
                n1409 = Absolute Value(x=w1958) -> (abs(x)=w1956:i8)
                n1410 = call "SetByteParam.vi"("SetNo"=w1955, "ParNo"=w1957, "Data"=w1956, "zDll"=w1954) -> ()  [unwired: 6 in, 2 out]
              }
            }
          }
        }
      }
      event "Small R Cluster.R0", "Small R Cluster.R1", "Small R Cluster.R2", "Small R Cluster.R3", "Small R Cluster.R4", "Small R Cluster.R5", "Small R Cluster.R6", "Small R Cluster.R7", "Small R Cluster.R8", "Small R Cluster.R9", "Small T Cluster.T0", "Small T Cluster.T1", "Small T Cluster.T2", "Small T Cluster.T3", "Small T Cluster.T4", "Small T Cluster.T5", "Small T Cluster.T6", "Small T Cluster.T7", "Small T Cluster.T8", "Small T Cluster.T9": Mouse Down {
        n1411 = event-data() -> ()  [unwired: 1 in, 8 out]
      }
      event Mouse Down {
        n1412 = event-data() -> ()  [unwired: 1 in, 8 out]
      }
      event Value Change {
        # "Update channel names on the small bottom panel when the names are changed."
        n1413 = event-data() -> ("NewVal"=→"AVS names small":T10)  [unwired: 1 in, 5 out]
      }
      event "CS.Mode1.Next": Value Change {
        # "Go to next step in CS auto mode."
        n1414 = event-data() -> ()  [unwired: 1 in, 6 out]
        n1415 = Unbundle By Name(w1967) -> ("TempStabilized"=w1966:refnum<user-event>)
        n1416 = flat-sequence {
          tunnel: w1966 -> [w1969]
          frame #0 {
            n1417 = call "Current Time(double).vi"() -> ("Current Time (double)"=w1968:dbl)  [unwired: 6 in, 1 out]
            n1418 = local write "_TimeOld"(w1968) -> ()
          }
          frame #1 {
            n1419 = Generate User Event(user event=w1969, event data cluster=TRUE ("event data")) -> ()  [unwired: 2 in, 2 out]
          }
        }
      }
      event "CS.Mode1.Auto Advance": Value Change {
        n1420 = event-data() -> ("NewVal"=w1972:bool)  [unwired: 1 in, 5 out]
        n1421 = case shown="True" w1972 {
          frame False {
          }
          frame True {
            # "Set timer to zero (01-01-1904) so the first point is set immediately, w/o wainting for time delay."
            # "If automatic mode is enabled- fire TempStabilized event to record current R,T,I values and start sweeping through TCS channels arrays"
            n1422 = disable-structure shown="Disabled" {
              frame Disabled {
                n1423 = Generate User Event(event data cluster="" ("event data")) -> ()  [unwired: 3 in, 2 out]
                "_TimeOld" <- 0.0 ("Timer")
              }
              frame Enabled {
              }
            }
          }
        }
      }
      event "CS.Mode1.Start", "CS.Mode2.Start": Value Change {
        n1424 = event-data() -> ("NewVal"=w1976:bool)  [unwired: 1 in, 5 out]
        n1425 = case shown="True" w1976 {
          frame False {
          }
          frame True {
            w1977 = TRUE
            # "Switch on the current sources."
            n1426 = property on="ON" class="Bool (strict)"() -> ("Value"=w1981:bool)  [unwired: 2 in, 2 out]
            n1427 = property on="ON" class="Bool (strict)"() -> ("Value"=w1980:bool)  [unwired: 2 in, 2 out]
            n1428 = property on="ON" class="Bool (strict)"() -> ("Value"=w1979:bool)  [unwired: 2 in, 2 out]
            n1429 = property on="ON" class="Bool (strict)"() -> ("Value"=w1978:bool)  [unwired: 2 in, 2 out]
            n1430 = Exclusive Or(1:w1981, 2:w1977) -> (0:w1985:bool)
            n1431 = Exclusive Or(1:w1980, 2:w1977) -> (0:w1983:bool)
            n1432 = Exclusive Or(1:w1979, 2:w1977) -> (0:w1982:bool)
            n1433 = Exclusive Or(1:w1978, 2:w1977) -> (0:w1984:bool)
            n1434 = property on="Toggle ON/OFF" class="Bool (strict)"("Value"=w1985) -> ()  [unwired: 2 in, 2 out]
            n1435 = property on="Toggle ON/OFF" class="Bool (strict)"("Value"=w1983) -> ()  [unwired: 2 in, 2 out]
            n1436 = property on="Toggle ON/OFF" class="Bool (strict)"("Value"=w1982) -> ()  [unwired: 2 in, 2 out]
            n1437 = property on="Toggle ON/OFF" class="Bool (strict)"("Value"=w1984) -> ()  [unwired: 2 in, 2 out]
          }
        }
      }
      event "CS.Mode1.PID.Enabled": Value Change {
        # "Enable/disable the PID loop"
        n1438 = event-data() -> ("NewVal"=w2000:bool)  [unwired: 1 in, 5 out]
        n1439 = Unbundle By Name(w1989) -> ("Reset PID loop"=w1988:refnum<user-event>)
        n1440 = call "IsDisabled.vi"("Enabled?"=w2000) -> ("Numeric"=w2003:i16)
        n1441 = Generate User Event(user event=w1988, event data cluster="" ("event data")) -> ()  [unwired: 2 in, 2 out]
        n1442 = property on="PID setup" class="Clust (strict)"("Disabled"=w2003) -> ()  [unwired: 2 in, 2 out]
        n1443 = property on="FB on" class="Enum (strict)"() -> ("Value"=w1997:enum16{"Resistance", "Temperature"})  [unwired: 2 in, 2 out]
        n1444 = property on="CS.Mode1.PID Channel" class="Enum (strict)"() -> ("Value"=w1987:enum16{"0", "1", "2", "3"})  [unwired: 2 in, 2 out]
        n1445 = property on="Enabled" class="Bool (strict)"() -> ("Value"=w1991:bool)  [unwired: 2 in, 2 out]
        n1446 = Initialize Array(FALSE, 4 ("dimension size")) -> (w1993:bool[])
        n1447 = And(x=TRUE ("new element/subarray"), y=w1991) -> (x .and. y?=w1990:bool)
        n1448 = Index Array(array=string[] ["%#_g uA", "%#_g mK"], index=w1997) -> (element=w1999:string)
        n1449 = Replace Array Subset(array=w1993, new element=w1990, index=w1987) -> (w1996:bool[])
        n1450 = local write "CS.Mode1.PID Column"(w1996) -> ()
        n1451 = Select(t=w1999, s=w2000, f="%#_g uA") -> ()  [unwired: 1 out]
      }
      event "CS.Mode1.Reset PID": Value Change {
        # "Reset the PID loop"
        n1452 = event-data() -> ()  [unwired: 1 in, 6 out]
        n1453 = Unbundle By Name(w2006) -> ("Reset PID loop"=w2005:refnum<user-event>)
        n1454 = Generate User Event(user event=w2005, event data cluster="" ("event data")) -> ()  [unwired: 2 in, 2 out]
      }
      event Value Change {
        n1455 = event-data() -> ("NewVal"=w2012:dbl)  [unwired: 1 in, 5 out]
        n1456 = Unbundle By Name(w2010) -> ("Reset PID loop"=w2009:refnum<user-event>)
        n1457 = Generate User Event(user event=w2009, event data cluster="" ("event data")) -> ()  [unwired: 2 in, 2 out]
        n1458 = property on="Enabled" class="Bool (strict)"() -> ("Value"=w2014:bool)  [unwired: 2 in, 2 out]
        n1459 = Initialize Array(FALSE, 4 ("dimension size")) -> (w2016:bool[])
        n1460 = And(x=TRUE ("new element/subarray"), y=w2014) -> (x .and. y?=w2013:bool)
        n1461 = Replace Array Subset(array=w2016, new element=w2013, index=w2012) -> (→"CS.Mode1.PID Column":bool[])
        n1462 = Index Array(array=string[] ["%#_g uA", "%#_g mK"], index=w2012) -> ()  [unwired: 1 out]
      }
      event "CS.Mode1.List": Value Change {
        n1463 = event-data() -> ("NewVal"=w2025:T23[][])  [unwired: 1 in, 5 out]
        n1464 = local read "CS.Mode1.List:Index"() -> (w2024:i32)
        n1465 = Decrement(x=w2024) -> (x-1=w2023:i32)
        n1466 = Array Size(array=w2025) -> (size(s)=w2027:i32[])
        n1467 = Index Array(array=w2027) -> (element=→"CS.Mode1.List:Count":i32)  [unwired: 1 in]
        n1468 = Index Array(array=w2025, index (row)=w2023) -> (element=→"_CSMode1List[i]":T23[])  [unwired: 1 in]
      }
      event "CS.Mode1.List": Shortcut Menu Activation? {
        n1469 = event-data() -> ()  [unwired: 1 in, 7 out]
        n1470 = event-data() -> ()  [unwired: 2 in, 1 out]
      }
      event "CS.Mode1.List": Shortcut Menu Selection (App) {
        n1471 = event-data() -> ("ItemTag"=w2030:string)  [unwired: 1 in, 7 out]
        n1472 = case shown="\"APP_SC_COPY_DATA\"" w2030 {
          frame Default {
          }
          frame "APP_SC_PASTE_DATA" {
            n1473 = invoke class="App" method="Clipboard.Read"() -> ("Read Clipbrd"=w2033:string)  [unwired: 3 in, 2 out]
            n1474 = Spreadsheet String To Array(format string="%d", spreadsheet string=w2033) -> (array=w2031:dbl[][])  [unwired: 2 in]
            n1475 = local write "CS.Mode1.List"(w2031) -> ()
          }
          frame "APP_SC_COPY_DATA" {
            n1476 = local read "CS.Mode1.List"() -> (w2036:T23[][])
            n1477 = Array To Spreadsheet String(array=w2036, 3:"%d" ("format string")) -> (spreadsheet string=w2034:string)  [unwired: 1 in]
            n1478 = invoke class="App" method="Clipboard.Write"("Param 0"=w2034) -> ()  [unwired: 3 in, 4 out]
          }
        }
      }
      event "CS.Mode1.List:To First": Value Change {
        n1479 = event-data() -> ("OldVal"=w2038:bool)  [unwired: 1 in, 5 out]
        n1480 = local write "CS.Mode1.List:To First"(w2038) -> ()
        n1481 = property on="CS.Mode1.List:Index" class="DigNum (strict)"("Val(Sgnl)"=1 ("Value (Signaling)")) -> ()  [unwired: 2 in, 2 out]
      }
      event "CS.Mode1.List:Next": Value Change {
        n1482 = event-data() -> ("OldVal"=w2041:bool)  [unwired: 1 in, 5 out]
        n1483 = local write "CS.Mode1.List:Next"(w2041) -> ()
        n1484 = local read "CS.Mode1.List:Index"() -> (w2043:i32)
        n1485 = Increment(x=w2043) -> (x+1=w2042:i32)
        n1486 = property on="CS.Mode1.List:Index" class="DigNum (strict)"("Val(Sgnl)"=w2042) -> ()  [unwired: 2 in, 2 out]
      }
      event "CS.Mode1.List:Prev": Value Change {
        n1487 = event-data() -> ("OldVal"=w2045:bool)  [unwired: 1 in, 5 out]
        n1488 = local write "CS.Mode1.List:Prev"(w2045) -> ()
        n1489 = local read "CS.Mode1.List:Index"() -> (w2047:i32)
        n1490 = Decrement(x=w2047) -> (x-1=w2046:i32)
        n1491 = property on="CS.Mode1.List:Index" class="DigNum (strict)"("Val(Sgnl)"=w2046) -> ()  [unwired: 2 in, 2 out]
      }
      event "CS.Mode1.List:Clear": Value Change {
        n1492 = event-data() -> ()  [unwired: 1 in, 6 out]
        n1493 = flat-sequence {
          frame #0 {
            n1494 = local write "CS.Mode1.List"(T23[][] [] ("I_list")) -> ()
          }
          frame #1 {
            n1495 = property on="CS.Mode1.List:To First" class="Bool (strict)"("Val(Sgnl)"=TRUE ("Value (Signaling)")) -> ()  [unwired: 2 in, 2 out]
          }
        }
      }
      event "CS.Mode1.List:Index": Value Change {
        w2072 = 10  # Lines to scroll
        n1496 = event-data() -> ("NewVal"=w2055:i32)  [unwired: 1 in, 5 out]
        n1497 = Array Size(array="CS.Mode1.List") -> (size(s)=w2058:i32[])
        n1498 = Index Array(array=w2058) -> (element=w2056:i32)  [unwired: 1 in]
        n1499 = call "Current Time(double).vi"() -> ("Current Time (double)"=w2052:dbl)  [unwired: 6 in, 1 out]
        n1500 = local write "CS.Mode1.List:Count"(w2056) -> ()
        n1501 = local write "_TimeOld"(w2052) -> ()
        n1502 = In Range and Coerce(upper limit=w2056, x=w2055, lower limit=1) -> (coerced(x)=w2053:i32)  [unwired: 1 out]
        "CS.Mode1.List:Index" <- w2053
        n1503 = Decrement(x=w2053) -> (x-1=w2054:i32)
        n1504 = Initialize Array(FALSE, w2072) -> (w2073:bool[])
        n1505 = Index Array(array="CS.Mode1.List", index (row)=w2054) -> (element=w2075:T23[])  [unwired: 1 in]
        n1506 = local write "_CSMode1List[i]"(w2075) -> ()
        n1507 = Subtract(x=w2054, y=w2072) -> (x-y=w2062:i32)
        n1508 = Increment(x=w2062) -> (x+1=w2061:i32)
        n1509 = Decrement(x=w2072) -> (x-1=w2070:i32)
        n1510 = In Range and Coerce(upper limit=inf, x=w2061, lower limit=0) -> (coerced(x)=w2060:dbl)  [unwired: 1 out]
        n1511 = In Range and Coerce(upper limit=w2070, x=w2054, lower limit=0) -> (coerced(x)=w2067:i32)  [unwired: 1 out]
        n1512 = control-ref of="CS.Mode1.List"() -> (w2065:refnum<vi>)
        n1513 = Build Array(w2060, 0 ("element")) -> (w2066:dbl[])
        n1514 = Replace Array Subset(array=w2073, new element=TRUE ("new element/subarray"), index=w2067) -> (→"CS.Mode1.Row":bool[])
        n1515 = property class="Arr (strict)"(reference=w2065, "Index Values"=w2066) -> ()  [unwired: 1 in, 2 out]
      }
      event "CS.Mode1.List:Save": Value Change {
        n1516 = event-data() -> ()  [unwired: 1 in, 6 out]
        n1517 = call "File Dialog6"() -> ("selected path"=w2079:path, "cancelled"=w2078:bool)  [unwired: 12 in, 2 out]
        n1518 = case shown="False" w2078 {
          tunnel: w2079 -> [w2080 _]
          frame False {
            n1519 = local read "CS.Mode1.List"() -> (w2082:T23[][])
            n1520 = call <vilib>:"Write To Spreadsheet File (DBL).vi"("format (%.3f)"="%.1f", "2D data"=w2082, "file path (dialog if empty)"=w2080) -> ()  [unwired: 5 in, 1 out]
          }
          frame True {
          }
        }
      }
      event "CS.Mode1.List:Load": Value Change {
        n1521 = event-data() -> ()  [unwired: 1 in, 6 out]
        n1522 = call "File Dialog5"() -> ("selected path"=w2084:path, "cancelled"=w2085:bool)  [unwired: 12 in, 2 out]
        n1523 = case shown="False" w2085 {
          tunnel: w2084 -> [w2086 _]
          frame False {
            n1524 = call <vilib>:"Read From Spreadsheet File (DBL).vi"("file path (dialog if empty)"=w2086) -> ("all rows"=w2087:dbl[][])  [unwired: 6 in, 4 out]
            n1525 = local write "CS.Mode1.List"(w2087) -> ()
          }
          frame True {
          }
        }
      }
      event "CS.Mode1.Write To Log": Value Change {
        n1526 = event-data() -> ()  [unwired: 1 in, 6 out]
        n1527 = Unbundle By Name(w2090) -> ("TempStabilized"=w2089:refnum<user-event>)
        n1528 = Generate User Event(user event=w2089, event data cluster=FALSE ("event data")) -> ()  [unwired: 2 in, 2 out]
      }
      event "CS.Mode2.Add Row": Value Change {
        n1529 = event-data() -> ()  [unwired: 1 in, 6 out]
        n1530 = call "Currents-Temp list  - add new range.vi"("List in"="CS.Mode2.List", "Array"="CS.Mode2.New Row") -> ("Sorted list out"=w2094:dbl[][])  [unwired: 3 in, 1 out]
        n1531 = local write "CS.Mode2.List"(w2094) -> ()
      }
      event "CS.Mode2.List": Shortcut Menu Selection (User) {
        n1532 = event-data() -> ("CtlRef"=w2099:refnum<vi>, "Coords"=w2098:T70, "ItemPath"=w2097:string)  [unwired: 1 in]
        n1533 = case shown="\"Erase Range\"" w2097 {
          tunnel: w2099 -> [_ w2105 _ w2111 w2112]
          tunnel: w2098 -> [_ w2104 _ _ _]
          frame Default {
          }
          frame "Erase Range" {
            (unwired) TRUE
            n1534 = call "Get Clicked Array Index.vi"("Coords"=w2104, "Array 2"=w2105) -> ("Clicked Index"=w2101:i32[])  [unwired: 9 in]
            n1535 = local read "CS.Mode2.List"() -> (w2103:dbl[][])
            n1536 = Index Array(array=w2101) -> (element=w2100:i32)  [unwired: 1 in]
            n1537 = call "Currents-Temp list - delete range.vi"("Numeric"=w2100, "I_list 2"=w2103) -> ("I_list"=w2102:dbl[][])  [unwired: 2 in]
            n1538 = local write "CS.Mode2.List"(w2102) -> ()
          }
          frame "Clear List" {
            n1539 = call "Currents-Temp list - check ranges.vi"() -> ("I_list out"=w2106:dbl[][])  [unwired: 5 in]
            n1540 = local write "CS.Mode2.List"(w2106) -> ()
          }
          frame "Copy Data" {
            n1541 = property class="Arr (strict)"(reference=w2111) -> ("Value"=w2107:dbl[][])  [unwired: 1 in, 2 out]
            n1542 = Array To Spreadsheet String(delimiter (Tab)="\t", array=w2107, 3:"%.4g" ("format string")) -> (spreadsheet string=w2110:string)
            n1543 = invoke class="App" method="Clipboard.Write"("Param 0"=w2110) -> ()  [unwired: 3 in, 4 out]
          }
          frame "Paste Data" {
            n1544 = invoke class="App" method="Clipboard.Read"() -> ("Read Clipbrd"=w2113:string)  [unwired: 3 in, 2 out]
            n1545 = Spreadsheet String To Array(delimiter (Tab)="\t", format string="%.4g", spreadsheet string=w2113) -> (array=w2116:dbl[][])  [unwired: 1 in]
            n1546 = property class="Arr (strict)"(reference=w2112, "Value"=w2116) -> ()  [unwired: 1 in, 2 out]
          }
        }
      }
      event "Graph-open popup": Value Change {
        w2128 = 128  # call and forget
        n1547 = event-data() -> ()  [unwired: 1 in, 6 out]
        n1548 = vi-ref "Graph popup.vi"() -> (w2124:refnum<vi>)
        n1549 = property class="VI"(reference=w2124) -> (error out=w2126:errorcluster, "Name"=w2127:string)  [unwired: 1 in, 1 out]
        n1550 = Open VI Reference(type specifier VI Refnum (for type only)=refnum<vi> refnum, vi path=w2127, options=w2128, error in (no error)=w2126) -> (vi reference=w2125:refnum<vi>, error out=w2119:errorcluster)  [unwired: 2 in]
        n1551 = control-ref of="Data"() -> (w2122:refnum<vi>)
        n1552 = local read "Sensor Names"() -> (w2121:T10)
        n1553 = call-by-ref "Start Asynchronous Call"(reference=w2125, error in=w2119, "Data"=w2122, "AVS names"=w2121) -> (reference out=w2120:refnum<vi>, error out=w2118:errorcluster)  [unwired: 18 in]
        n1554 = Close Reference(reference=w2120, error in (no error)=w2118) -> ()  [unwired: 1 out]
      }
      event "ColorBox": Mouse Move {
        n1555 = event-data() -> ("Coords"=w2132:T70)  [unwired: 1 in]
        n1556 = call <vilib>:"Picture to Pixmap.vi"("picture"="Colors") -> ("image data"=w2138:T69)  [unwired: 9 in, 1 out]
        n1557 = property on="Colors" class="Pict"() -> ("Position"=w2131:T77)  [unwired: 2 in, 2 out]
        n1558 = call <vilib>:"Unflatten Pixmap.vi"("image data"=w2138) -> ("24-bit pixmap"=w2133:u32[][])  [unwired: 4 in, 6 out]
        n1559 = Subtract(x=w2132, y=w2131) -> (x-y=w2136:T70)
        n1560 = Unbundle(w2136) -> ("Horizontal"=w2135:i32, "Vertical"=w2134:i32)
        n1561 = Index Array(array=w2133, index (row)=w2134, index (col)=w2135) -> (element=→"Color":u32)
      }
      event "ColorBox": Mouse Down {
        n1562 = event-data() -> ()  [unwired: 1 in, 8 out]
        n1563 = property on="ColorBox" class="TabCtl (strict)"("Visible"=FALSE) -> ()  [unwired: 2 in, 2 out]
      }
      event "Set Color": Value Change {
        n1564 = event-data() -> ()  [unwired: 1 in, 6 out]
        n1565 = property on="ColorBox" class="TabCtl (strict)"("Visible"=TRUE) -> ()  [unwired: 2 in, 2 out]
      }
    }
    "General Error" <- w70
  }
  n1566 = flat-sequence {
    tunnel: w36 -> [w2143]
    frame #0 {
      n1567 = Wait on Occurrence(2:w2143) -> ()  [unwired: 2 in, 1 out]
    }
    frame #1 {
      n1568 = while {
        i -> [w2154]
        stop <- "Stop" stop-if-true
        # "AVS/zBridge read-out"
        n1569 = case shown="False" "Pause" {
          tunnel: w2154 -> [w2157 _]
          frame False {
            # "For the first measurement set Stab.Time=12 s to do autoranging"
            n1570 = property on="Runtime Settings" class="Clust (strict)"() -> ("Value"=w2179:T27)  [unwired: 2 in, 2 out]
            n1571 = local read "zBridge.Active Channels"() -> (w2162:T21)
            n1572 = Unbundle By Name(w2179) -> ("Stabilisation Delay"=w2171:dbl, "Averages"=w2164:u16, "Last Channel"=w2178:i8, "Read AVS channels from"=w2177:i8)
            n1573 = property on="Bridge Type" class="Enum (strict)"() -> ("Value"=w2175:T61)  [unwired: 2 in, 2 out]
            n1574 = call "Split Exc&Range.vi"("Excitations 2"="AVS Exc&Ranges") -> ("Excitations"=w2168:T29, "Ranges"=w2163:T78)  [unwired: 4 in]
            n1575 = property on="_AVS_VISA" class="VISAName"() -> ("Value"=w2176:refnum<visa-resource-name>)  [unwired: 2 in, 2 out]
            n1576 = Cluster To Array(cluster=w2162) -> (array=w2161:bool[])
            n1577 = call "If First Iteration.vi"("Iteration"=w2157, "Value In"=w2171, "Default"=12.0) -> ("Value Out"=w2170:dbl)
            n1578 = case shown="\"AVS47A (GPIB interface)\"" w2175 {
              tunnel: w2176 -> [w2189 w2200 _ _ _]
              tunnel: w2170 -> [w2185 w2203 w2210 _ _]
              tunnel: w2164 -> [w2186 w2202 _ _ _]
              tunnel: w2178 -> [w2187 w2198 _ _ _]
              tunnel: w2177 -> [w2188 w2199 _ _ _]
              tunnel: w2168 -> [w2190 w2194 _ _ _]
              tunnel: [w2182 w2193 errorcluster {"status"=FALSE, "code"=0, "source"=""} ("error out") w2226 errorcluster {"status"=FALSE, "code"=0, "source"=""} ("error out")] -> w2167
              tunnel: w2163 -> [w2184 w2196 w2211 w2227 w2231]
              tunnel: TRUE ("Autorange") -> [w2180 w2197 _ _ _]
              tunnel: [w2183 w2195 w2211 w2227 w2231] -> w2160
              tunnel: [w2181 w2192 w2209 w2220 dbl[] [] ("Data array")] -> w2165
              tunnel: w2161 -> [_ w2191 _ _ _]
              tunnel: "_ScanData" -> [_ _ _ w2216 _]
              frame "AVS47A (GPIB interface)" {
                # "AVS 47 (GPIB)"
                n1579 = call "AVS47IB_do_single_scan.vi"("AVS Port"=w2189, "Stabilization Delay"=w2185, "Autorange"=w2180, "Number of Averages"=w2186, "Last Channel"=w2187, "First Channel"=w2188, "Excitations"=w2190, "Ranges"=w2184) -> ("error out"=w2182:errorcluster, "R"=w2181:dbl[], "Ranges"=w2183:T79)  [unwired: 3 in, 2 out]
              }
              frame "AVS47B (RS232 interface)" {
                # "AVS 47B (RS232)"
                n1580 = Type Cast(type=refnum<visa-resource-name> refnum ("dup VISA session"), x=w2200) -> (*(type *) &x=w2204:refnum<visa-resource-name>)
                n1581 = call "Scanner.vi"("STABILIZATION  DELAY"=w2203, "FIRST CH TO SCAN"=w2199, "LAST CH TO SCAN"=w2198, "Autorange"=w2197, "AVERAGE COUNT"=w2202, "Excitation"=w2194, "Range"=w2196, "VISA resource"=w2204, "array"=w2191) -> ("RI"=w2192:dbl[], "Range out"=w2195:T80, "error out 2"=w2193:errorcluster)  [unwired: 1 in, 3 out]
              }
              frame "AVS Emulation" {
                (unwired) dbl[] [0.0, 0.0, 0.0, 0.0] ("I")
                n1582 = local read "CS.Automode Current"() -> (w2207:T23[])
                n1583 = Multiply(x=w2210, y=u32 1000 ("milliseconds to wait")) -> (x*y=w2214:dbl)
                n1584 = Wait (ms)(milliseconds to wait=w2214) -> ()  [unwired: 1 out]
                n1585 = Index Array(array=w2207, index=3) -> ()  [unwired: 1 out]
                n1586 = property on="CS.Current Value" class="Arr (strict)"() -> ("Value"=w2213:dbl[])  [unwired: 2 in, 2 out]
                n1587 = Multiply(x=1000.0, y=w2213) -> (x*y=w2205:dbl[])
                n1588 = call "AVS Emulate.vi"("Currents"=w2205, "Sampling time"=w2210) -> ("R"=w2209:dbl[])  [unwired: 1 in, 1 out]
              }
              frame "Impedance Bridge" {
                n1589 = local read "Bridge status"() -> (w2221:errorcluster)
                n1590 = local read "_zBridgeDll"() -> (w2228:path)
                n1591 = call "Read Data from Single Channel.vi"("error in (no error)"=w2221, "zDll"=w2228) -> ("error out"=w2226:errorcluster, "Value"=w2225:dbl, "Scan parameters/Error string"=→"_zBridgeParText":string, "Set number"=w2218:u8, "Error code"=→"Error code":u8, "Unit"=→"_ZBridgeUnit":string, "ScanParameters out"=w2219:T81)  [unwired: 3 in]
                "_zBridgeSetNr" <- w2218
                n1592 = call "ScanParameters FGV.vi"("Action"=Action."Write", "index"=w2218, "ScanParameters in"=w2219) -> ()  [unwired: 8 in, 1 out]
                n1593 = Replace Array Subset(array=w2216, new element=w2225, index=w2218) -> (w2220:dbl[])
              }
              frame "Disabled", Default {
              }
            }
            "Bridge status" <- w2167
            n1594 = property on="_AVSRanges" class="Clust (strict)"("Val(Sgnl)"=w2160) -> ()  [unwired: 2 in, 2 out]
            n1595 = property on="_ScanData" class="Arr (strict)"("Val(Sgnl)"=w2165) -> ()  [unwired: 2 in, 2 out]
            n1596 = property on="Delay" class="DigNum (strict)"() -> ("Value"=w2159:u32)  [unwired: 2 in, 2 out]
            n1597 = Multiply(x=u32 1000, y=w2159) -> (x*y=w2174:u32)
            n1598 = Wait (ms)(milliseconds to wait=w2174) -> ()  [unwired: 1 out]
          }
          frame True {
          }
        }
      }
      n1599 = while {
        stop <- w2233 stop-if-true
        (unwired) errorcluster {"status"=FALSE, "code"=0, "source"=""} ("Value")
        # "Current source control"
        n1600 = property on="CS status" class="Clust (strict)"() -> ("Value"=w2232:errorcluster)  [unwired: 2 in, 2 out]
        n1601 = stacked-sequence {
          seq-local: [w2261 _ _ _] -> [_ w2270 _ _]
          seq-local: [w2260 _ _ _] -> [_ w2269 _ _]
          seq-local: [_ w2270 _ _] -> [_ _ w2280 _]
          seq-local: [_ w2268 _ _] -> [_ _ w2279 _]
          tunnel: w2232 -> [w2259 _ _ _]
          frame #0 {
            # "Write 0 instead of the actual \ncurrent value to log if there \nis no current flowing."
            # "Read current CS status"
            n1602 = local read "_CSClassRef"() -> (w2249:refnum<class "CS.lvclass">)
            n1603 = call-dynamic "Read.vi"("CS in"=w2249, "error in (no error)"=w2259, "Optional"=FALSE) -> ("CS out"=w2261:refnum<class "CS.lvclass">, "I0"=w2252:T82, "I1"=w2253:T82, "I2"=w2254:T82, "I3"=w2255:T82, "error out"=w2260:errorcluster)  [unwired: 11 in]
            n1604 = Unbundle By Name(w2252) -> ("Current (string)"=w2247:string, "I?"=w2246:bool)
            n1605 = Unbundle By Name(w2253) -> ("Current (string)"=w2262:string, "I?"=w2245:bool)
            n1606 = Unbundle By Name(w2254) -> ("Current (string)"=w2250:string, "I?"=w2244:bool)
            n1607 = Unbundle By Name(w2255) -> ("Current (string)"=w2263:string, "I?"=w2243:bool)
            n1608 = call "CS Data Converter.vi"("CS Data"=w2252) -> ("CS Indicator"=→"I0":T83)
            n1609 = call "CS Data Converter.vi"("CS Data"=w2253) -> ("CS Indicator"=→"I1":T83)
            n1610 = call "CS Data Converter.vi"("CS Data"=w2254) -> ("CS Indicator"=→"I2":T83)
            n1611 = call "CS Data Converter.vi"("CS Data"=w2255) -> ("CS Indicator"=→"I3":T83)
            n1612 = Fract/Exp String To Number(string=w2247) -> (number=w2251:dbl)  [unwired: 3 in, 1 out]
            n1613 = Fract/Exp String To Number(string=w2262) -> (number=w2258:dbl)  [unwired: 3 in, 1 out]
            n1614 = Fract/Exp String To Number(string=w2250) -> (number=w2257:dbl)  [unwired: 3 in, 1 out]
            n1615 = Fract/Exp String To Number(string=w2263) -> (number=w2256:dbl)  [unwired: 3 in, 1 out]
            n1616 = Build Array(w2246, w2245, w2244, w2243) -> (w2242:bool[])
            n1617 = Not(x=w2242) -> (.not. x?=w2238:bool[])
            n1618 = Build Array(w2251, w2258, w2257, w2256) -> (w2241:dbl[])
            "CS.Current Value" <- w2241
            n1619 = for {
              tunnel: w2238 -> [w2267] mode=indexing
              tunnel: w2241 -> [w2266] mode=indexing
              tunnel: dbl[] [0.0, 0.0, 0.0, 0.0] ("t") -> [w2265] mode=indexing
              tunnel: [w2264] -> w2239 mode=indexing
              n1620 = Select(t=w2265, s=w2267, f=w2266) -> (s? t:f=w2264:dbl)
            }
            "CS.Actual Current" <- w2239
          }
          frame #1 {
            n1621 = Wait (ms)(milliseconds to wait=100) -> ()  [unwired: 1 out]
            n1622 = call <vilib>:"Clear Errors.vi"("error in (no error)"=w2269) -> ("error out"=w2268:errorcluster)  [unwired: 6 in]
          }
          frame #2 {
            # "Only send data to CS if\nnew value was entered"
            # "Set CS status"
            n1623 = call "CS OnOff & Gated and Current & Range.vi"("I in"="CS.I0") -> ("OnOff & Gated"=w2291:T84, "Current & Range"=w2276:T85, "I out"=w2284:T86)  [unwired: 2 in]
            n1624 = call "CS OnOff & Gated and Current & Range.vi"("I in"="CS.I1") -> ("OnOff & Gated"=w2290:T84, "Current & Range"=w2275:T85, "I out"=w2281:T86)  [unwired: 2 in]
            n1625 = call "CS OnOff & Gated and Current & Range.vi"("I in"="CS.I2") -> ("OnOff & Gated"=w2287:T84, "Current & Range"=w2274:T85, "I out"=w2282:T86)  [unwired: 2 in]
            n1626 = call "CS OnOff & Gated and Current & Range.vi"("I in"="CS.I3") -> ("OnOff & Gated"=w2286:T84, "Current & Range"=w2273:T85, "I out"=w2283:T86)  [unwired: 2 in]
            n1627 = local write "CS.I0"(w2284) -> ()
            n1628 = local write "CS.I1"(w2281) -> ()
            n1629 = local write "CS.I2"(w2282) -> ()
            n1630 = local write "CS.I3"(w2283) -> ()
            n1631 = local read "CS.Automode Current"() -> (w2272:T23[])
            n1632 = Equal To 0?(x="CS.Mode") -> (x = 0?=w2277:bool)
            n1633 = call "CS_set_channels.vi"("CS in"=w2280, "Current & Range0"=w2276, "Current & Range1"=w2275, "Current & Range 2"=w2274, "Current & Range3"=w2273, "error out"=w2279, "I_automode"=w2272, "Auto?"=w2277) -> ("CS.lvclass out"=w2296:refnum<class "CS.lvclass">, "Current Changed?"=w2293:bool, "error out 2"=w2297:errorcluster)  [unwired: 9 in]
            n1634 = call-dynamic "Set Mode.vi"("CS.lvclass in"=w2296, "On&G 0"=w2291, "On&G 1"=w2290, "On&G 2"=w2287, "On&G 3"=w2286, "error in (no error)"=w2297) -> ("CS.lvclass out"=w2294:refnum<class "CS.lvclass">, "error out"=w2295:errorcluster)  [unwired: 12 in]
            n1635 = case shown="True" w2293 {
              selector: w2293 -> [_ w2298]
              frame False {
              }
              frame True {
                n1636 = property on="_CurrentsChanged" class="Bool (strict)"("Val(Sgnl)"=w2298) -> ()  [unwired: 2 in, 2 out]
              }
            }
            n1637 = local write "_CSClassRef"(w2294) -> ()
            n1638 = property on="CS status" class="Clust (strict)"("Value"=w2295) -> ()  [unwired: 2 in, 2 out]
          }
          frame #3 {
            n1639 = Wait (ms)(milliseconds to wait=100) -> ()  [unwired: 1 out]
          }
        }
        n1640 = local read "Stop"() -> (w2233:bool)
      }
      n1641 = while {
        stop <- w2146 stop-if-true
        # "zBridge status read-out"
        n1642 = property on="Bridge Type" class="Enum (strict)"() -> ("Value"=w2144:T61)  [unwired: 2 in, 2 out]
        n1643 = case shown="\"Impedance Bridge\"" w2144 {
          frame Default {
          }
          frame "Impedance Bridge" {
            n1644 = local read "_zBridgeDll"() -> (w2152:path)
            n1645 = local read "Bridge status"() -> (w2151:errorcluster)
            n1646 = call "ScanStatus.vi"("error in (no error)"=w2151, "zDll"=w2152) -> ("error out"=w2150:errorcluster, "Status"=w2148:i32, "Channel"=w2149:i32)  [unwired: 7 in]
            n1647 = local write "Bridge status"(w2150) -> ()
            n1648 = call "zBridge Format Status.vi"("Status"=w2148, "Channel"=w2149) -> ("Status"=→"zBridge.Scan Phase":T87, "Active channel"=→"zBridge.Active channel":T88)  [unwired: 2 in]
          }
        }
        n1649 = Wait (ms)(milliseconds to wait=u32 200) -> ()  [unwired: 1 out]
        n1650 = local read "Stop"() -> (w2146:bool)
      }
    }
  }
  n1651 = disable-structure shown="Disabled" {
    frame Disabled {
      w2313 = string[] ["Paste Data from Clipboard"] ("item names")
      (unwired) enum32{"Page 1"}."Page 1" ("Tab Control 4")
      n1652 = local read "CS.Automode Current"() -> (w2308:T23[])
      n1653 = local read "zBridge.Active Channels"() -> ()  [unwired: 1 in]
      n1654 = property on="Bridge Channel" class="DigNum (strict)"() -> ("Value"=w2301:i32)  [unwired: 2 in, 2 out]
      n1655 = local read item#-1() -> ()  [unwired: 1 out]
      n1656 = Index Array(array=w2308) -> (element #1=w2304:T23, element #2=w2305:T23, element #3=w2306:T23, element #4=w2307:T23)  [unwired: 4 in]
      n1657 = property class="XYGraph (strict)" props=["YScale", "Mapping Mode"]() -> ()  [unwired: 2 in, 3 out]
      n1658 = property on="I" class="DigNum (strict)"("Val(Sgnl)"=w2304) -> ()  [unwired: 2 in, 2 out]
      n1659 = property on="I" class="DigNum (strict)"("Val(Sgnl)"=w2305) -> ()  [unwired: 2 in, 2 out]
      n1660 = property on="I" class="DigNum (strict)"("Val(Sgnl)"=w2306) -> ()  [unwired: 2 in, 2 out]
      n1661 = property on="I" class="DigNum (strict)"("Val(Sgnl)"=w2307) -> ()  [unwired: 2 in, 2 out]
      n1662 = Insert Menu Items(4:4, 7:w2313, 8:w2313) -> ()  [unwired: 3 in, 3 out]
      n1663 = Equal?(y=w2301) -> (x = y?=w2300:bool)  [unwired: 1 in]
      n1664 = Equal?(x=w2301, y=-1) -> (x = y?=w2303:bool)
      n1665 = Or(x=w2300, y=w2303) -> ()  [unwired: 1 out]
      n1666 = property on="ON" class="Boolean (strict)"() -> ("Value"=w2320:bool)  [unwired: 2 in, 2 out]
      n1667 = control-ref of="zBridge.Active Channels"() -> ()  [unwired: 1 out]
      n1668 = Exclusive Or(1:w2320, 2:TRUE ("x")) -> (0:w2319:bool)
      n1669 = property on="Toggle ON/OFF" class="Bool (strict)"("Value"=w2319) -> ()  [unwired: 2 in, 2 out]
      n1670 = control-ref of="CS.Mode1.List"() -> (w2315:refnum<vi>)
      n1671 = property class="Arr (strict)"(reference=w2315) -> ("Index Values"=w2316:u32[])  [unwired: 1 in, 2 out]
      n1672 = Index Array(array=w2316) -> (element=w2317:u32)  [unwired: 1 in]
      n1673 = property on="Side Panel" class="TabCtl (strict)"() -> ("Pages"=w2321:refnum<vi>[])  [unwired: 2 in, 2 out]
      n1674 = property on="CS.Mode1.List:Index" class="DigNum (strict)"("Val(Sgnl)"=w2317) -> ()  [unwired: 2 in, 2 out]
      n1675 = Index Array(array=w2321, index=1) -> (element=w2322:refnum<vi>)
      n1676 = Generate User Event(event data cluster="" ("event data")) -> ()  [unwired: 3 in, 2 out]
      n1677 = property class="Page"(reference=w2322, "PageVis"=TRUE ("Page Visible")) -> ()  [unwired: 1 in, 2 out]
      n1678 = property on="FB on" class="Enum (strict)" props=["Value"]() -> ()  [unwired: 2 in, 3 out]
      n1679 = Initialize Array(0.0 ("element"), 4 ("dimension size")) -> (w2309:dbl[])
      n1680 = local write "CS.Automode Current"(w2309) -> ()
    }
    frame Enabled {
    }
  }
